vi "COD主界面（列队使用）.vi"() -> (8 "多列列表框":i32(listbox))   [LabVIEW 2016, in "斯坦道CODMn.lvlib"]
uses:
  <vilib>/Analysis/6fits.llb/Curve Fitting Criteria.ctl
  <vilib>/Utility/miscctls.llb/LVPointTypeDef.ctl
  <vilib>/Utility/config.llb/Read Key (I32).vi
  <vilib>/Utility/config.llb/Read Key (Double).vi
  <vilib>/Utility/config.llb/Read Key (Boolean).vi
  <vilib>/Utility/config.llb/Write Key (Double).vi
  <vilib>/Utility/config.llb/Write Key (Boolean).vi
  <vilib>/Utility/config.llb/Write Key (I32).vi
  <vilib>/Waveform/WDTFileIO.llb/Read Waveform from File.vi
  <vilib>/ptbypt/NI_PtbyPt.lvlib
  <vilib>/Utility/config.llb/NI_LVConfig.lvlib
  <vilib>/Analysis/NI_AALPro.lvlib
panel:
  out "CODMn序列号":string
  out "CODMn软件版本：":string
  in  "标样核查量程选择":enum32{"H", "L", "AUTO"}(ring)=enum."AUTO"
  in  "标样浓度":dbl
  in  "零点核查量程选择":enum32{"H", "L", "AUTO"}(ring)=enum."AUTO"
  in  "零点核查浓度":dbl
  out "序列号":string
  in  "采水泵排液时间/s:":i32
  in  "采水泵润洗时间/s:":i32
  in  "采水泵沉淀时间/s:":i32
  in  "采水泵进样时间/s:":i32
  in  "常规版/认证版":enum16{"常规版", "认证版", "浮台版"}(ring)
  in  "释放串口":bool
  in  "打开串口":bool
  in  "保存参数":dbl[](array[numeric])
  out "报警数字":i16
  out "CODMn工作状态":T1(ring)
  out "ORP-K":string
  out "ORP-B":string
  out "ORP-A":string
  out "x = y?":bool
  out "稀释倍数解释":string
  in  "跨度量程选择":enum32{"H", "L", "AUTO"}(ring)=enum."AUTO"
  in  "跨度液浓度":dbl
  in  "水样":dbl
  in  "蒸馏水":dbl
  in  "标液":dbl
  in  "质控样":dbl
  in  "加标回收":dbl
  in  "草酸钠":dbl
  in  "高锰酸钾":dbl
  in  "硫酸":dbl
  out "量程解释说明":string
  in  "高切低阈值:":dbl
  in  "低切高阈值:":dbl
  in  "自动切换量程:":enum16{"关闭", "自动切换测一次", "自动切换测两次"}(ring)
  in  "修正系数":dbl
  in  "标准液浓度":dbl
  in  "温度":dbl
  in  "恒温时间":dbl
  in  "基本量程":enum16{"L", "H"}(ring)
  in  "CODMn零点核查选择":enum16{"零点核查走纯水管", "零点核查走零漂管"}(ring)
  in  "锁定按钮":bool
  in  "低量程稀释倍数:":i8=1
  out "切换量程连续测两次":bool
  in  "高量程稀释倍数:":i8=2
  in  "一键写入":bool
  in  "测量模式(公式)":u16(ring)=1 items=["水样测试"=1, "标样核查"=2, "零点核查"=3, "跨度核查"=4, "空白测试"=5, "平行样"=6, "加标回收"=7]
  out "基本量程(显示)":string
  out "测量模式(显示)":string
  in  "量程切换次数":u8
  out "数据时间":string
  out "断电排液标记":bool
  out "COM":string
  in  "启用5":bool
  in  "校准5":bool
  in  "泵滴定数5":dbl
  in  "浓度5":dbl
  in  "启用4":bool
  in  "校准4":bool
  in  "泵滴定数4":dbl
  in  "浓度4":dbl
  out "波形时间":timestamp
  in  "历史波形":bool
  out "滴定数-ORP值":u16[](array[numeric]) caption="数组"
  in  "关闭 3":bool
  in  "滴定曲线":bool
  out "ORP滴定曲线":u16[](graph)
  out "空白测试标记":bool
  out "跨度核查标记":bool
  out "启动选择 2":u16(ring) items=["水样测试", "标样核查", "零点核查", "跨度核查", "空白测试", "加标回收", "平行样", "校零", "校标"]
  in  "量程选择":enum16{"低量程", "高量程", "0-2量程"}(ring)
  in  "手动控制":bool
  in  "选用水样":enum16{"葡萄糖", "草酸钠"}(ring)
  in  "方程系数":cluster{"K":dbl, "b":dbl, "X^2":dbl} {"X^2" format="%#.6g"; "b" format="%#.6g"; "K" format="%#.6g"}
  out "多项式系数":dbl[](array[numeric])
  out "XY图":cluster{"X Values":dbl[], "Y Values":dbl[]}[](graph)
  in  "模型":enum32{"线性", "多项式"}(ring)
  out "启动时间":timestamp format="%<%Y/%m/%d %H:%M:%S>T"
  in  "关闭 2":bool
  out "r^2":dbl format="%.8g"
  out "拟合公式":string
  out "b":dbl format="%#.4g"
  out "K":dbl format="%#.4f"
  out "当前校准":i32
  in  "启用3":bool
  in  "启用2":bool
  in  "启用1":bool
  in  "校准3":bool
  in  "校准2":bool
  in  "校准1":bool
  in  "泵滴定数3":dbl
  in  "泵滴定数2":dbl
  in  "泵滴定数1":dbl
  in  "浓度3":dbl
  in  "浓度2":dbl
  in  "浓度1":dbl
  in  "写入":bool
  out "测量模式数字":i32
  out "零点核查标记":bool
  out "排液故障":bool
  out "进水样超量程":bool
  out "标样核查标记":bool
  out "平行样测量":bool
  out "加标回收测量":bool
  out "质控样测量":bool
  out "待机":bool
  out "校标错误":bool
  out "校零错误":bool
  out "测量错误":bool
  out "草酸钠报警":bool
  out "高锰酸钾报警":bool
  out "加热故障":bool
  out "温控器故障":bool
  out "ORP故障":bool
  out "排液标记":bool
  out "故障标记":bool
  out "校标标记":bool
  out "校零标记":bool
  out "通讯状态":bool
  out "水样测量":bool
  in  "读取":bool
  in  "返回":bool
  in  "校准配置":bool
  in  "零点泵计量数 2":dbl
  in  "标度泵计量数 2":dbl
  out "标度滴定值":dbl
  out "零点滴定值":dbl
  in  "保存":bool
  in  "关闭":bool
  out "仪器时间":timestamp format="%<%Y/%m/%d %H:%M:%S>T"
  out "秒":u16
  out "分":u16
  out "COD浓度（mg/L)":dbl format="%.2g"
  out "进样管":dbl
  out "高锰酸钾":dbl
  out "草酸钠":dbl
  out "硫酸":dbl
  out "ORP显示":dbl
  out "温度":dbl
  out "加热":bool
  out "搅拌":bool
  out "进硫酸":bool
  out "进加标回收样":bool
  out "进零点核查样":bool
  out "进标液":bool
  out "进蒸馏水":bool
  out "进水样":bool
  out "进草酸钠":bool
  out "进高锰酸钾":bool
  out "定时启动":bool
  in  "启动":bool
  in  "故障清除":bool
  in  "参数配置":bool
  in  "停止":bool
  in  "单步启动":bool
  out "系统时间":timestamp
  in  "时间校准":bool
  out "报警簇":T2
  out "模式（受控）":u16
  # "测量时间："
  # "(水样~加标回收)"
  # "mV"
  # "℃"
  # "注：遇到加热故障和排液故障时仪器不能正常启动，\n必须排查故障并点击报警清除按钮方可运行。"
  # "mg/L"
  # "基本参数设置"
  # "校零校标结果"
  # "泵计量参数设置"
  # "校零结果："
  # "校零滴定值："
  # "加热恒温温度(℃):"
  # "水样："
  # "高锰酸钾："
  # "校标结果："
  # "标度滴定值："
  # "恒温时间(分钟):"
  # "草酸钠："
  # "蒸馏水："
  # "零点泵计量值："
  # "标准液浓度(mg/L):"
  # "硫酸："
  # "标液："
  # "标度泵计量值："
  # "修正系数："
  # "跨度核查浓度："
  # "零点核查样:"
  # "基本量程(L、H)可选:"
  # "跨度量程选择："
  # "加标回收样："
  # "零点核查浓度："
  # "标样浓度："
  # "零点量程选择："
  # "标样量程选择："
  # "是否启用"
  # "泵滴定数"
  # "浓度"
  # "辅\n助\n计\n算\n区"
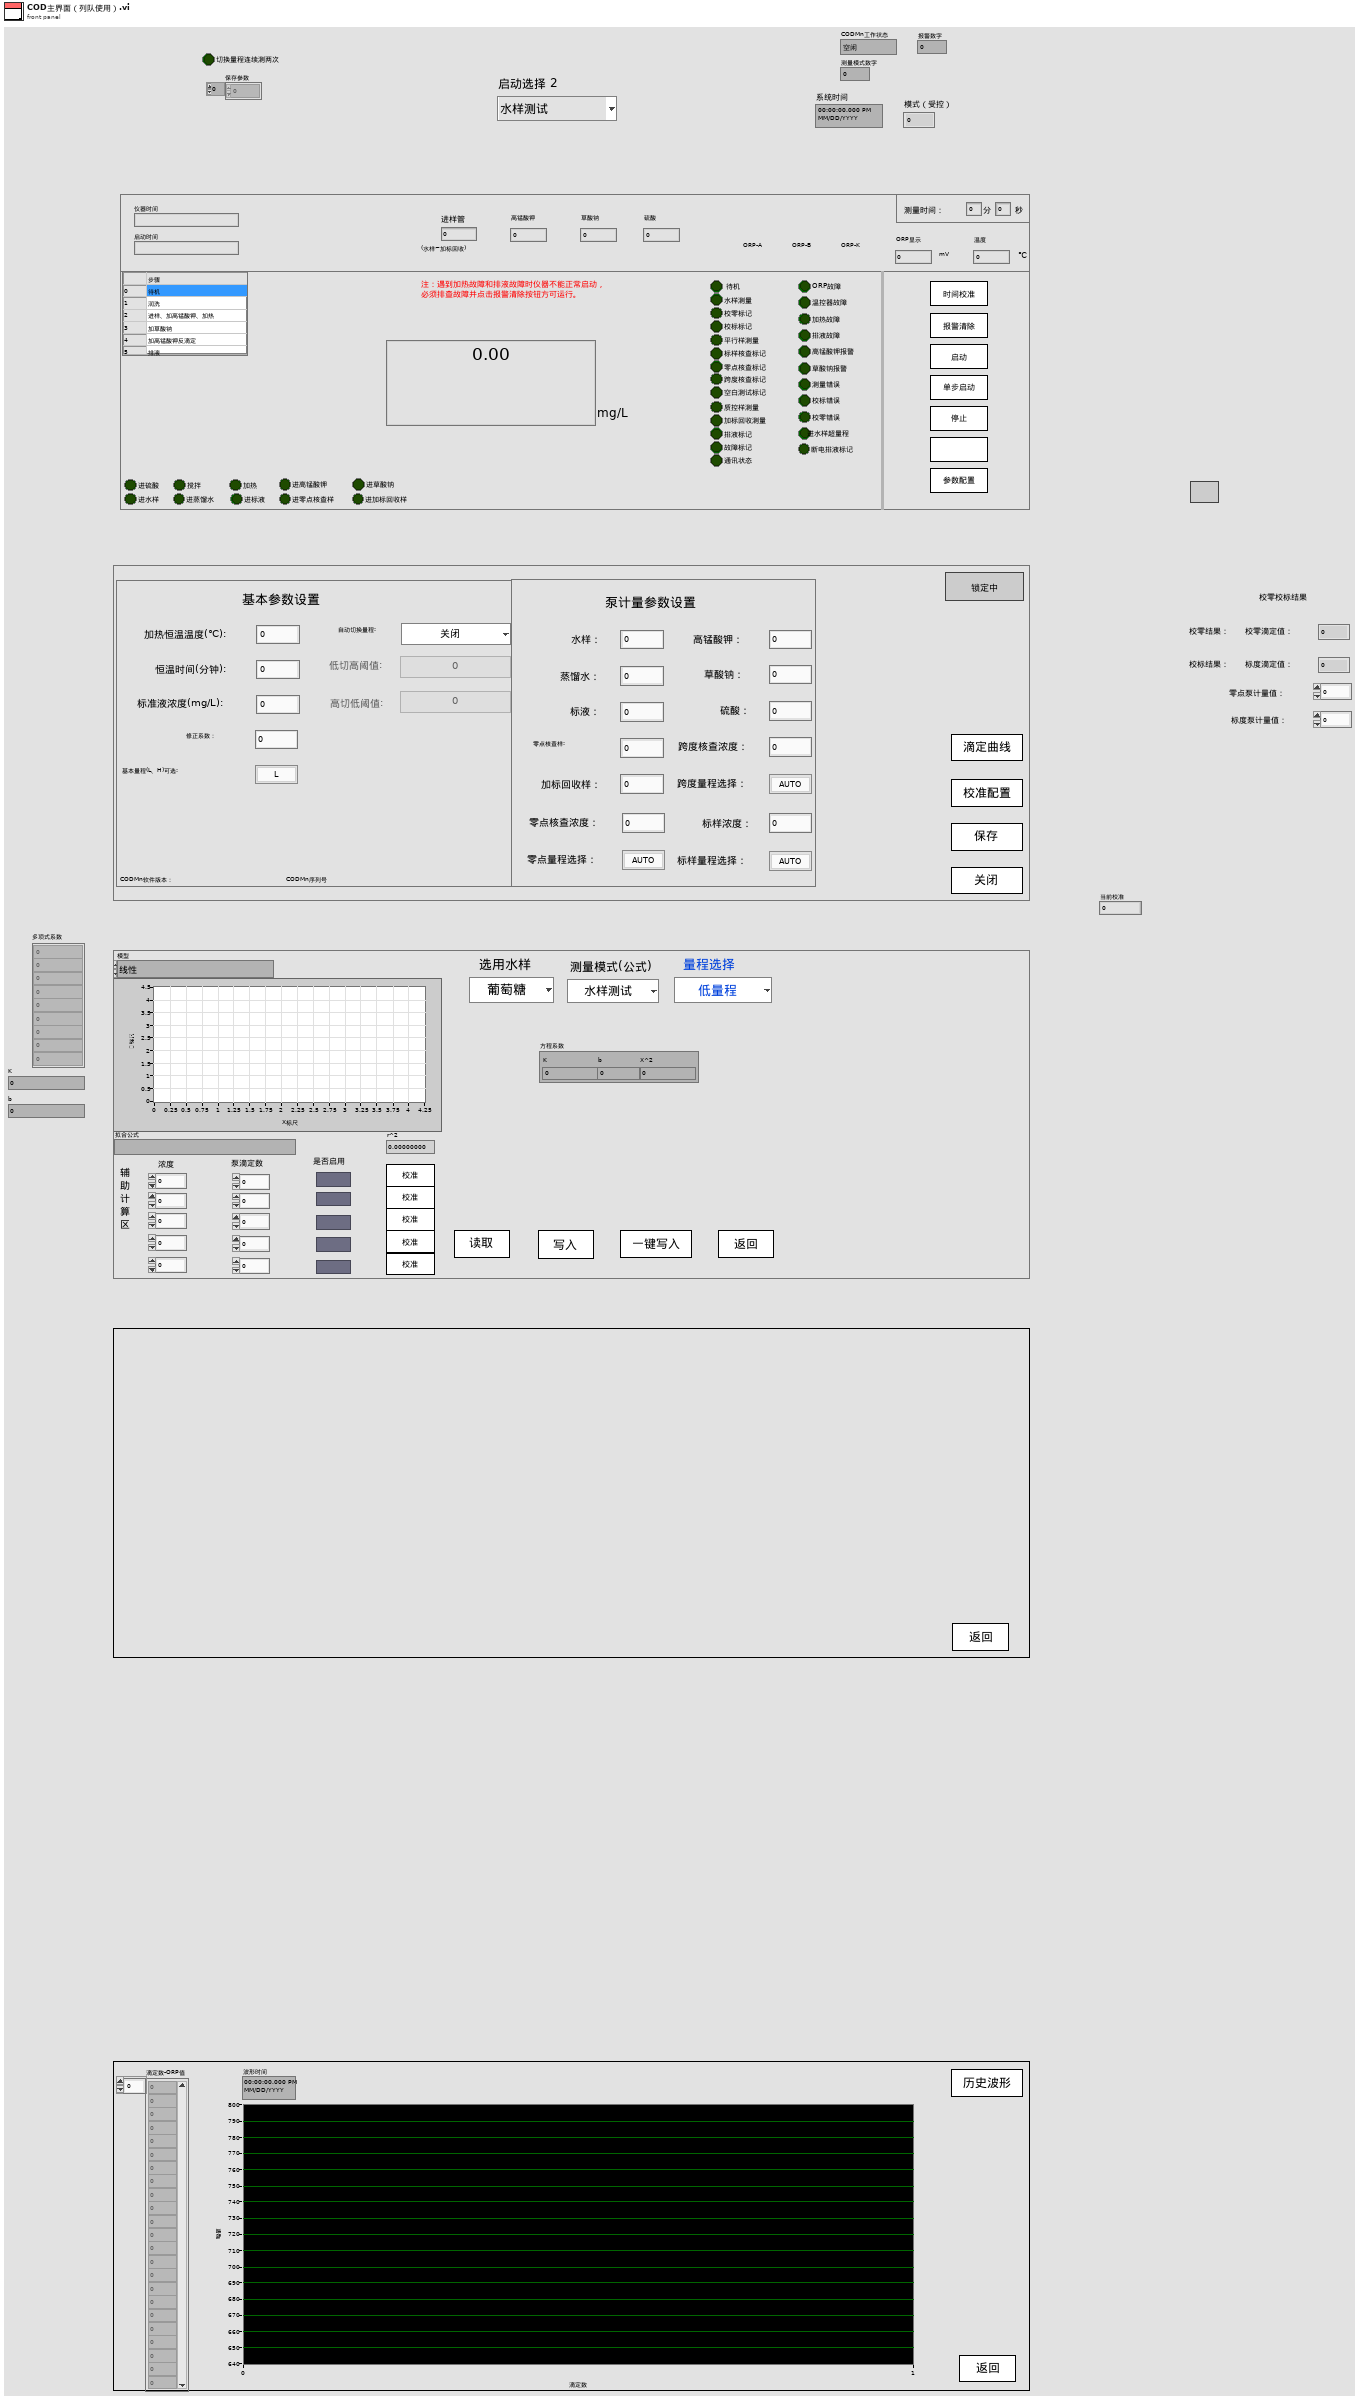
[diagram p1: front panel]
types:
  T1 = enum16{"空闲", "水样测试", "标样核查", "零点核查", "跨度核查", "空白测试", "平行样测试", "质控样", "空白校准", "标样校准", "加标回收"}
  T2 = cluster{"ORP故障":bool, "温控器故障":bool, "加热故障":bool, "高锰酸钾报警":bool, "草酸钠报警":bool, "测量错误":bool, "校零错误":bool, "校标错误":bool, " 进水样超量程":bool, "排液阀故障":bool}
  T3 = cluster{"命令":string, "测量模式":enum16{"水样测量", "标样核查", "零点核查", "跨度核查", "空白测试", "加标回收", "平行样", "校零", "校标"}, "CODMn量程切换":enum32{"H", "L", "AUTO"}}
  T4 = cluster{"时间":timestamp, "测量模式":string, "数据类型":string, "检测值":sgl, "单位":string, "数据标识":string, "因子编码":string, "标样参考值":sgl, "ORP-A":sgl, "ORP-B":sgl, "ORP-K":sgl, "COD滴定值":sgl, "高锰酸钾滴定数":sgl, "温度":sgl, "量程":sgl, "LastTime":timestamp}
  T5 = cluster{"因子编码":u32, "单位":u16, "标样参考值":sgl, "水样数据时间":timestamp, "水样实测值":sgl, "水样数据标识":string, "标样数据时间":timestamp, "标样实测值":sgl, "标样数据标识":string, "空白数据时间":timestamp, "空白实测值":sgl, "空白数据标识":string, "零点核查数据时间":timestamp, "零点核查实测值":sgl, "零点核查数据标识":string, "跨度核查数据时间":timestamp, "跨度核查实测值":sgl, "跨度核查数据标识":string, "加标回收数据时间":timestamp, "加标回收实测值":sgl, "加标回收数据标识":string, "平行样数据时间":timestamp, "平行样实测值":sgl, "平行样数据标识":string}
  T6 = enum8{"Enabled", "Disabled", "Disabled and Grayed Out"}
  T7 = typedef "NI_LVConfig.lvlib/Config Data RefNum.ctl" = refnum<k1>
  T8 = cluster{"数组 2[0]":sgl, "数组 2[1]":sgl, "数组 2[2]":sgl, "数组 2[3]":sgl, "数组 2[4]":sgl, "数组 2[5]":sgl, "数组 2[6]":sgl, "数组 2[7]":sgl, "数组 2[8]":sgl, "数组 2[9]":sgl, "数组 2[10]":sgl, "数组 2[11]":sgl, "数组 2[12]":sgl, "数组 2[13]":sgl, "数组 2[14]":sgl, "数组 2[15]":sgl, "数组 2[16]":sgl, "数组 2[17]":sgl, "数组 2[18]":sgl, "数组 2[19]":sgl, "数组 2[20]":sgl, "数组 2[21]":sgl, "数组 2[22]":sgl, "数组 2[23]":sgl, "数组 2[24]":sgl, "数组 2[25]":sgl, "数组 2[26]":sgl, "数组 2[27]":sgl, "数组 2[28]":sgl, "数组 2[29]":sgl, "数组 2[30]":sgl, "数组 2[31]":sgl, "数组 2[32]":sgl, "数组 2[33]":sgl, "数组 2[34]":sgl, "数组 2[35]":sgl, "数组 2[36]":sgl, "数组 2[37]":sgl, "数组 2[38]":sgl, "数组 2[39]":sgl, "数组 2[40]":sgl, "数组 2[41]":sgl}
  T9 = typedef "NI_AALPro.lvlib/Curve Fitting Criteria.ctl" = u16
  T10 = cluster{"测量模式":enum16{"水样测量", "标样核查", "零点核查", "跨度核查", "空白测试", "加标回收", "平行样", "校零", "校标"}}
  T11 = cluster{"仪器测试类型":enum16{"水样测试", "零点核查", "标样核查", "空白测试", "跨度核查", "加标回收", "平行样", "校零", "校标"}, "周期设置类型":enum16{"定点启动", "间隔启动"}, "定时功能启用":bool, "定时间隔":dbl, "24H周期设置":bool[]}
  T12 = typedef "LVDateTimeRec.ctl" = cluster{"秒数的小数部分":dbl, "秒":i32, "分":i32, "时":i32, "日":i32, "月":i32, "年":i32, "天数（周）":i32, "天数（年）":i32, "DST":i32}
  T13 = enum16{"水样测试", "零点核查", "标样核查", "空白测试", "跨度核查", "加标回收", "平行样", "校零", "校标"}
  T14 = cluster{"时间标识":timestamp, "设备":string, "日志信息":string}
  T15 = cluster{"时间标识":timestamp, "参数":string, "日志信息":string, "流程参数":string}
  T16 = cluster{"时间标识":timestamp, "设备":string, "日志信息":string, "流程参数":string}
  T17 = typedef "LVPointTypeDef.ctl" = cluster{"Horizontal":i16, "Vertical":i16}
  T18 = enum16{"水样测量", "标样核查", "零点核查", "跨度核查", "空白测试", "加标回收", "平行样", "校零", "校标"}
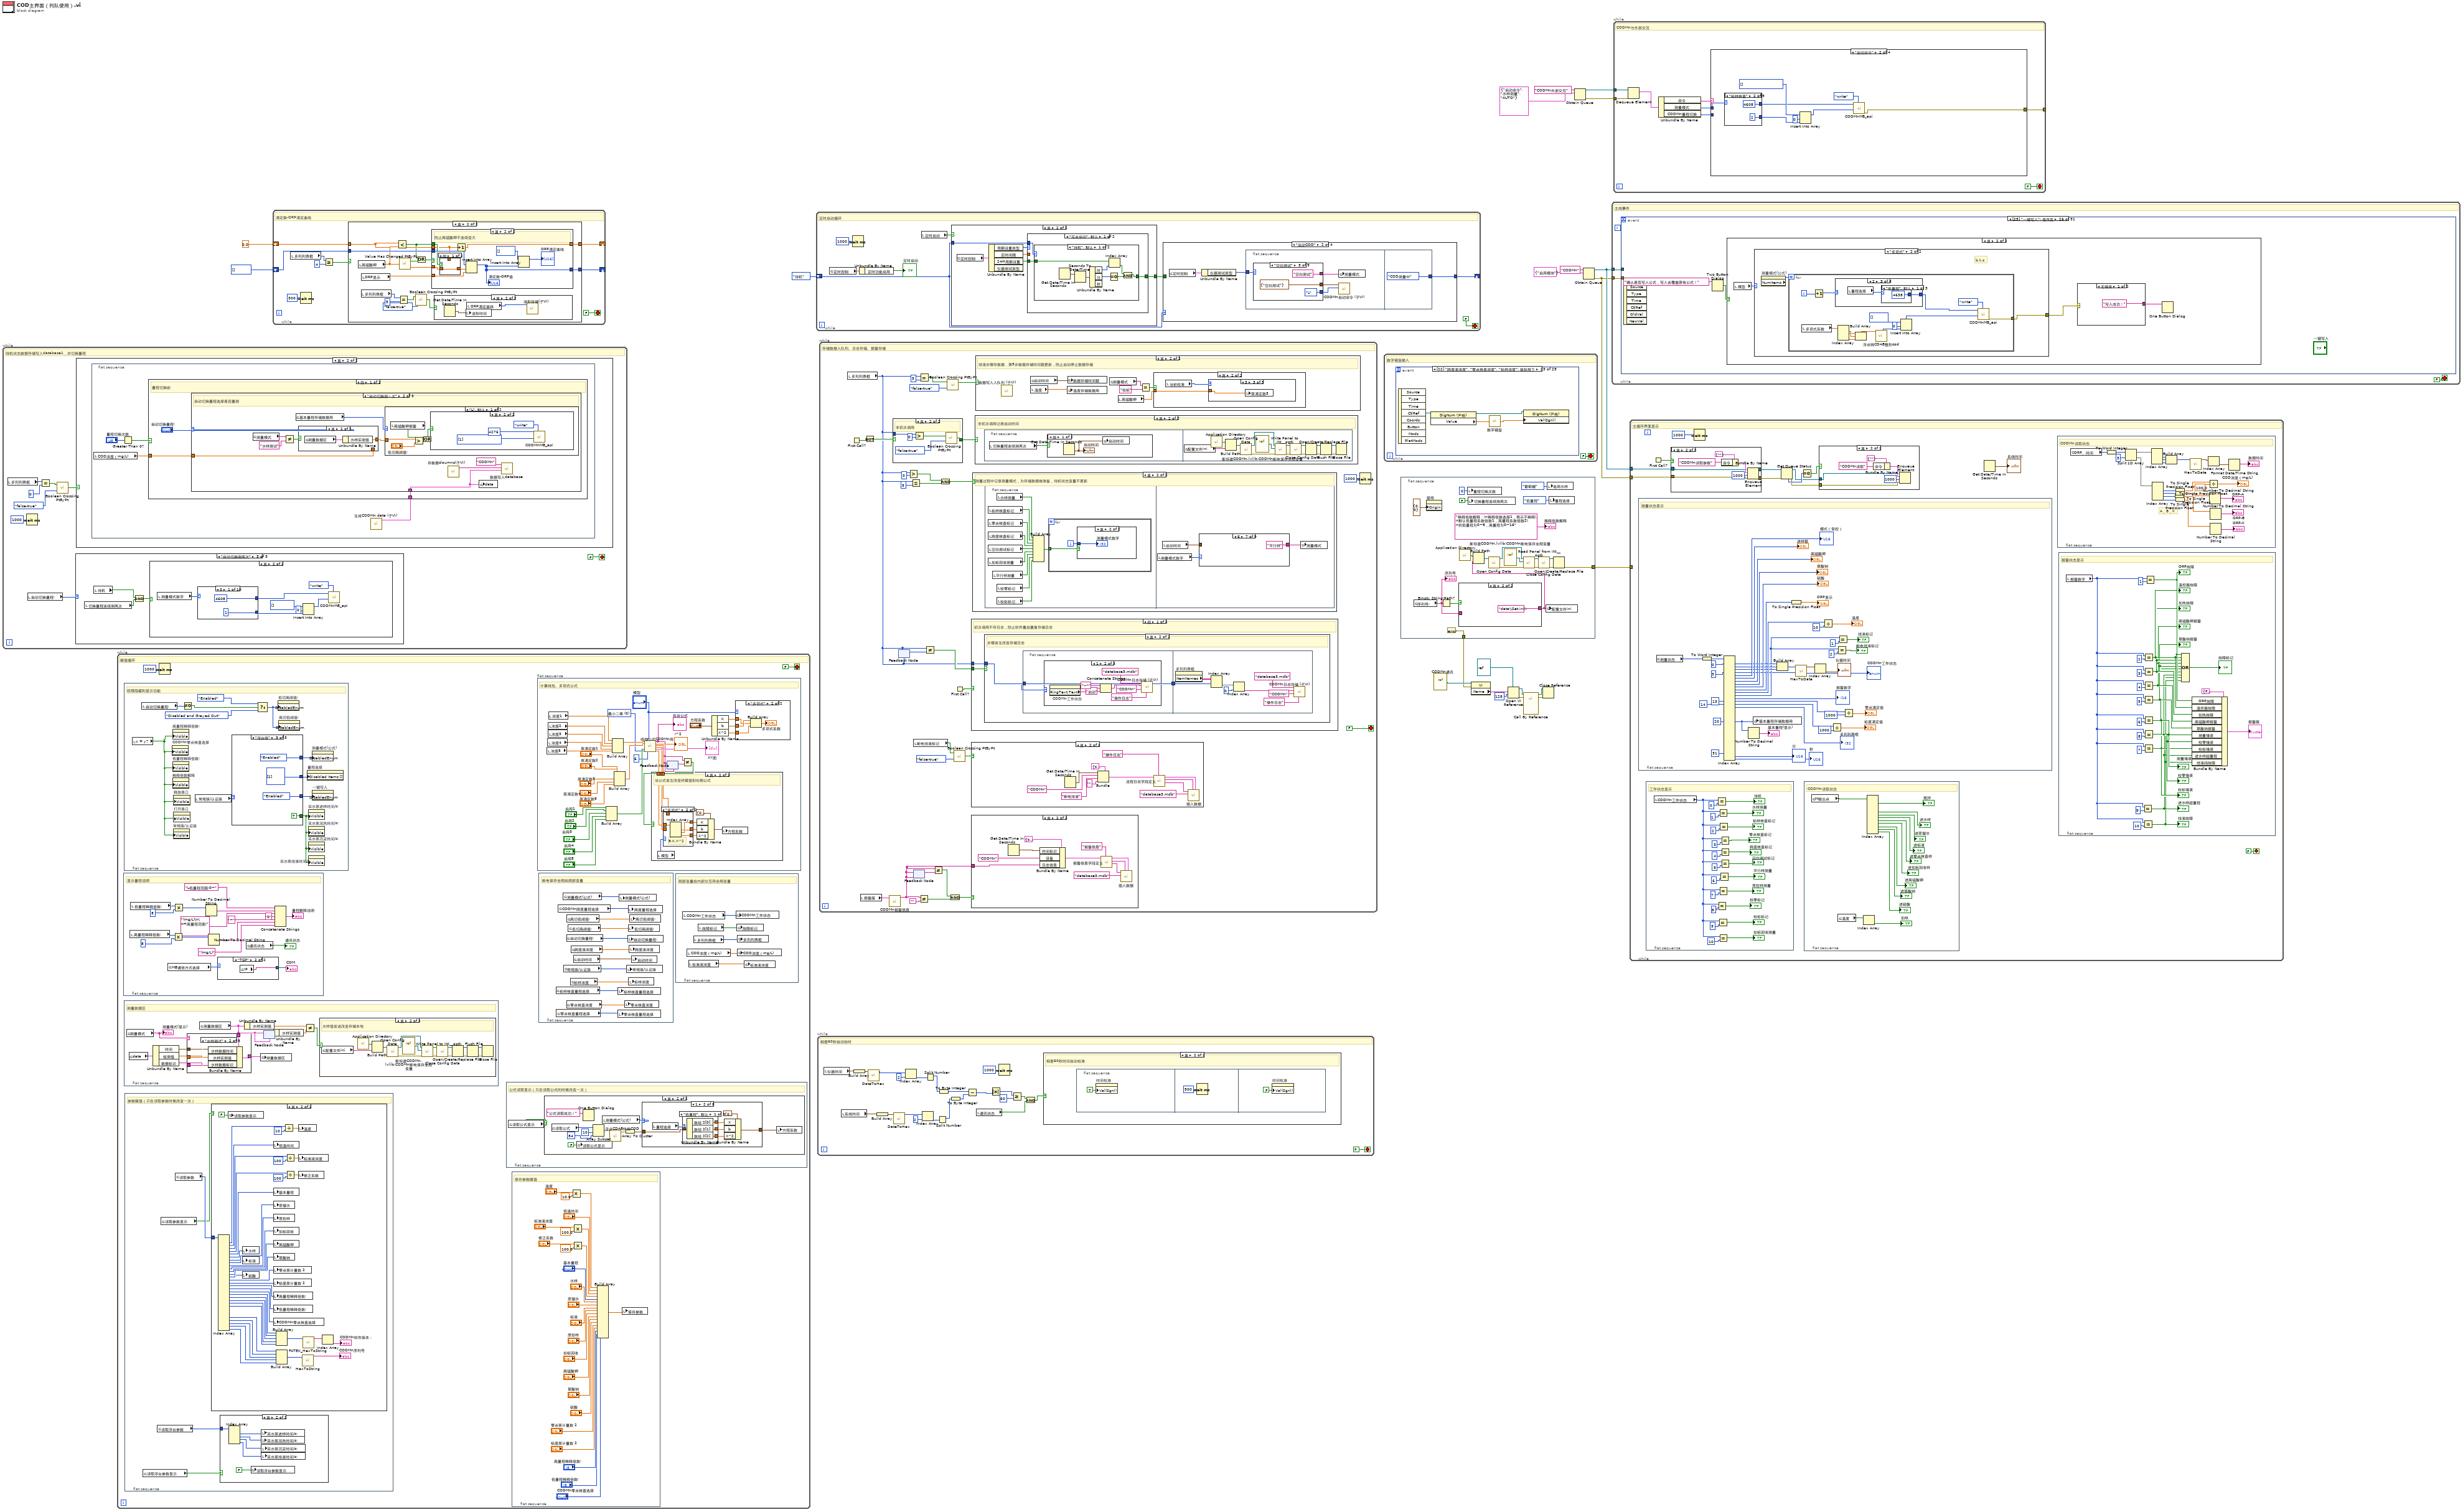
[diagram p0: block diagram]
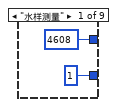
[diagram p3: hidden frame]
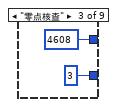
[diagram p4: hidden frame]
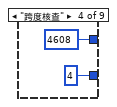
[diagram p5: hidden frame]
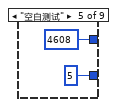
[diagram p6: hidden frame]
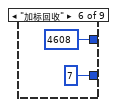
[diagram p7: hidden frame]
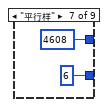
[diagram p8: hidden frame]
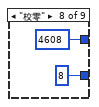
[diagram p9: hidden frame]
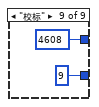
[diagram p10: hidden frame]
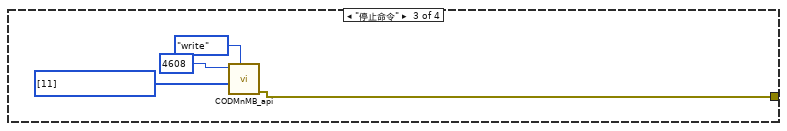
[diagram p11: hidden frame]
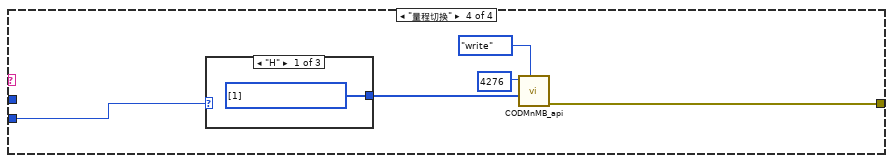
[diagram p12: hidden frame]
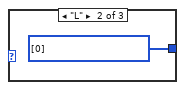
[diagram p13: hidden frame]
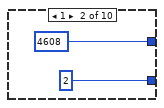
[diagram p19: hidden frame]
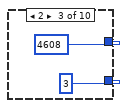
[diagram p20: hidden frame]
diagram:
  n1 = while {
    stop <- FALSE stop-if-true
    # "待机状态数据存储写入database1，并切换量程"
    n2 = local read "多列列表框"() -> (w27:i32)
    n3 = Wait (ms)(milliseconds to wait=u32 1000 ("等待时间（毫秒）")) -> ()  [unwired: 1 out]
    n4 = local read "自动切换量程:"() -> (w22:enum16{"关闭", "自动切换测一次", "自动切换测两次"})
    n5 = Equal?(x=w27, y=0) -> (x = y?=w25:bool)
    n6 = call <vilib>:"Boolean Crossing PtByPt.vi"("direction"=enum16{"either", "false-true", "true-false"}."false-true", "input"=w25) -> ("crossing"=w23:bool)  [unwired: 1 in]
    n7 = case shown="\"自动切换测两次\"" w22 {
      frame "关闭", Default {
      }
      frame "自动切换测一次" {
      }
      frame "自动切换测两次" {
        n8 = local read "切换量程连续测两次"() -> (w31:bool)
        n9 = local read "待机"() -> (w32:bool)
        n10 = Compound Arithmetic op=AND ("复合运算")(w32, w31) -> (w30:bool)
        n11 = case shown="真" w30 {
          frame False {
          }
          frame True {
            n12 = local read "测量模式数字"() -> (w36:i32)
            n13 = case shown="0" w36 {
              tunnel: [u16 4608 ("address") u16 4608 ("address") u16 4608 ("address") u16 4608 ("address") u16 4608 ("address") u16 4608 ("address") u16 4608 ("address") u16 4608 ("address") u16 4608 ("address") u16 4608 ("address")] -> w33
              tunnel: [u16 1 ("address") u16 2 ("address") u16 3 ("address") u16 4 ("address") u16 5 ("address") u16 7 ("address") u16 6 ("address") u16 8 ("address") u16 9 ("address") u16 0 ("address")] -> w39
              frame 0 {
              }
              frame 1 {
              }
              frame 2 {
              }
              frame 3 {
              }
              frame 4 {
              }
              frame 5 {
              }
              frame 6 {
              }
              frame 7 {
              }
              frame 8 {
              }
              frame 9, Default {
              }
            }
            n14 = Insert Into Array(array=u16[] [] ("values"), index=0 ("索引"), new element=w39) -> (w34:u16[])
            n15 = call "CODMnMB_api.vi"("STEP"=enum16{"open", "read", "write", "close"}."write", "values"=w34, "starting address"=w33) -> ()  [unwired: 6 in, 3 out]
          }
        }
      }
    }
    n16 = case shown="真" w23 {
      frame False {
      }
      frame True {
        n17 = flat-sequence {
          frame #0 {
            n18 = local read "COD浓度（mg/L)"() -> (w60:dbl)
            n19 = Greater Than 0?(x="量程切换次数") -> (x > 0?=w61:bool)
            n20 = call "生成CODMn data (子VI).vi"() -> ("data"=w63:T4)  [unwired: 11 in]
            n21 = case shown="假" w61 {
              tunnel: w63 -> [w65 w124]
              tunnel: w60 -> [w64 _]
              frame False {
                # "量程切换前"
                n22 = case shown="\"自动切换测一次\"" "自动切换量程:" {
                  tunnel: w65 -> [w67 w72 w98]
                  tunnel: w64 -> [_ w71 w97]
                  frame "关闭", Default {
                    # "关闭自动切换量程"
                    n23 = call "存数据cloumns(子VI).vi"() -> ("数组"=w69:string[])  [unwired: 11 in]
                    n24 = global write "COD读取DATA全局.vi" "data"(w67) -> ()
                    n25 = call "数据写入database.vi"("data"=w67, "columns"=w69, "table"="CODMn") -> ()  [unwired: 8 in, 1 out]
                  }
                  frame "自动切换测一次" {
                    # "自动切换量程选择是否重测"
                    n26 = global read "COD测量模式全局.vi" "测量模式"() -> (w78:string)
                    n27 = Not Equal?(x=w78, y="水样测试") -> (x != y?=w76:bool)
                    n28 = global read "COD读取DATA全局.vi" "基本量程存储数据用"() -> (w70:enum16{"L", "H"})
                    n29 = case shown="真" w76 {
                      tunnel: [w79 w80] -> w75
                      tunnel: w71 -> [w79 _]
                      frame False {
                      }
                      frame True {
                        n30 = global read "CODMn断电保存全局变量.vi" "测量数据区"() -> (w81:T5)
                        n31 = Unbundle By Name(w81) -> ("水样实测值"=w80:sgl)
                      }
                    }
                    n32 = case shown="\"L\", 默认" w70 {
                      tunnel: w75 -> [w84 w90]
                      frame "L", Default {
                        n33 = local read "高锰酸钾报警"() -> (w82:bool)
                        n34 = Greater?(x=w84, y="低切高阈值:") -> (0:w85:bool)
                        n35 = Or(x=w82, y=w85) -> (x .or. y?=w83:bool)
                        n36 = case shown="真" w83 {
                          frame False {
                          }
                          frame True {
                            n37 = call "CODMnMB_api.vi"("STEP"=enum16{"open", "read", "write", "close"}."write", "values"=u16[] [1], "starting address"=u16 4276) -> ()  [unwired: 6 in, 3 out]
                          }
                        }
                      }
                      frame "H" {
                        n38 = Less?(x=w90, y="高切低阈值:") -> (x < y?=w91:bool)
                        n39 = case shown="真" w91 {
                          frame False {
                          }
                          frame True {
                            n40 = call "CODMnMB_api.vi"("STEP"=enum16{"open", "read", "write", "close"}."write", "values"=u16[] [0], "starting address"=u16 4276) -> ()  [unwired: 6 in, 3 out]
                          }
                        }
                      }
                    }
                    n41 = call "存数据cloumns(子VI).vi"() -> ("数组"=w74:string[])  [unwired: 11 in]
                    n42 = global write "COD读取DATA全局.vi" "data"(w72) -> ()
                    n43 = call "数据写入database.vi"("data"=w72, "columns"=w74, "table"="CODMn") -> ()  [unwired: 8 in, 1 out]
                  }
                  frame "自动切换测两次" {
                    # "自动切换量程选择是否重测"
                    n44 = global read "COD读取DATA全局.vi" "基本量程存储数据用"() -> (w96:enum16{"L", "H"})
                    n45 = case shown="\"L\", 默认" w96 {
                      tunnel: w97 -> [w102 w113]
                      tunnel: w98 -> [w101 w112]
                      frame "L", Default {
                        n46 = local read "低切高阈值:"() -> (w103:dbl)
                        n47 = local read "高锰酸钾报警"() -> (w99:bool)
                        n48 = Greater?(x=w102, y=w103) -> (0:w104:bool)
                        n49 = Or(x=w104, y=w99) -> (x .or. y?=w100:bool)
                        n50 = case shown="真" w100 {
                          tunnel: w101 -> [w105 _]
                          frame False {
                            n51 = call "存数据cloumns(子VI).vi"() -> ("数组"=w107:string[])  [unwired: 11 in]
                            n52 = global write "COD读取DATA全局.vi" "data"(w105) -> ()
                            n53 = call "数据写入database.vi"("data"=w105, "columns"=w107, "table"="CODMn") -> ()  [unwired: 8 in, 1 out]
                          }
                          frame True {
                            n54 = call "CODMnMB_api.vi"("STEP"=enum16{"open", "read", "write", "close"}."write", "values"=u16[] [1], "starting address"=u16 4276) -> ()  [unwired: 6 in, 3 out]
                            "切换量程连续测两次" <- TRUE ("切换量程连续测两次")
                          }
                        }
                      }
                      frame "H" {
                        n55 = local read "高切低阈值:"() -> (w114:dbl)
                        n56 = Less?(x=w113, y=w114) -> (x < y?=w115:bool)
                        n57 = case shown="真" w115 {
                          tunnel: w112 -> [w116 _]
                          frame False {
                            n58 = call "存数据cloumns(子VI).vi"() -> ("数组"=w118:string[])  [unwired: 11 in]
                            n59 = global write "COD读取DATA全局.vi" "data"(w116) -> ()
                            n60 = call "数据写入database.vi"("data"=w116, "columns"=w118, "table"="CODMn") -> ()  [unwired: 8 in, 1 out]
                          }
                          frame True {
                            # "重测第一次不存数据"
                            n61 = call "CODMnMB_api.vi"("STEP"=enum16{"open", "read", "write", "close"}."write", "values"=u16[] [0], "starting address"=u16 4276) -> ()  [unwired: 6 in, 3 out]
                            n62 = local write "切换量程连续测两次"(TRUE ("切换量程连续测两次")) -> ()
                          }
                        }
                      }
                    }
                  }
                }
              }
              frame True {
                # "防止无限切量程"
                n63 = local write "量程切换次数"(u8 0 ("量程切换次数")) -> ()
                n64 = call "存数据cloumns(子VI).vi"() -> ("数组"=w126:string[])  [unwired: 11 in]
                n65 = call "数据写入database.vi"("data"=w124, "columns"=w126, "table"="CODMn") -> ()  [unwired: 8 in, 1 out]
                n66 = global write "COD读取DATA全局.vi" "data"(w124) -> ()
              }
            }
          }
        }
      }
    }
  }
  n67 = while {
    stop <- FALSE stop-if-true
    # "赋值循环"
    n68 = flat-sequence {
      frame #0 {
        # "显示量程说明"
        n69 = local read "高量程稀释倍数:"() -> (w487:i8)
        n70 = local read "低量程稀释倍数:"() -> (w497:i8)
        n71 = global read "CODMn断电保存全局变量.vi" "MB通信方式选择"() -> (w483:enum16{"串口", "TCP"})
        n72 = Multiply(x=w487, y=i8 8) -> (x*y=w485:i8)
        n73 = Multiply(x=w497, y=i8 8) -> (x*y=w489:i8)
        n74 = Number To Decimal String(number=w489) -> (decimal integer string=w494:string)  [unwired: 1 in]
        n75 = Number To Decimal String(number=w485) -> (decimal integer string=w492:string)  [unwired: 1 in]
        n76 = case shown="\"TCP\"" w483 {
          tunnel: [w500 w501] -> w488
          frame "串口", Default {
            n77 = global read "CODMn断电保存全局变量.vi" "VISA resource name"() -> (w500:refnum<visa-resource-name>)
          }
          frame "TCP" {
            n78 = global read "CODMn断电保存全局变量.vi" "IP"() -> (w501:string)
          }
        }
        "COM" <- w488
        n79 = global read "COD读取DATA全局.vi" "通讯状态"() -> (→"通讯状态":bool)
        n80 = Concatenate Strings("L低量程范围:0~" ("量程解释说明"), w494, "(mg/L)\n\nH高量程范围:" ("量程解释说明"), "0" ("字符串"), "~" ("量程解释说明"), w492, "(mg/L)" ("量程解释说明")) -> (→"量程解释说明":string)
      }
    }
    n81 = flat-sequence {
      frame #0 {
        # "权限隐藏和显示功能"
        n82 = local read "x = y?"() -> (w502:bool)
        n83 = local read "自动切换量程:"() -> (w509:enum16{"关闭", "自动切换测一次", "自动切换测两次"})
        n84 = property on="CODMn零点核查选择" class="Enum (严格)"("Visible"=w502) -> ()  [unwired: 2 in, 2 out]
        n85 = property on="高量程稀释倍数:" class="DigNum (严格)"("Visible"=w502) -> ()  [unwired: 2 in, 2 out]
        n86 = property on="低量程稀释倍数:" class="DigNum (严格)"("Visible"=w502) -> ()  [unwired: 2 in, 2 out]
        n87 = property on="稀释倍数解释" class="Str"("Visible"=w502) -> ()  [unwired: 2 in, 2 out]
        n88 = property on="常规版/认证版" class="Enum (严格)"("Visible"=w502) -> ()  [unwired: 2 in, 2 out]
        n89 = property on="释放串口" class="Bool"("Visible"=w502) -> ()  [unwired: 2 in, 2 out]
        n90 = property on="打开串口" class="Bool"("Visible"=w502) -> ()  [unwired: 2 in, 2 out]
        n91 = Not Equal To 0?(x=w509) -> (x != 0?=w508:bool)
        n92 = local read "常规版/认证版"() -> (w507:enum16{"常规版", "认证版", "浮台版"})
        n93 = case shown="\"浮台版\"" w507 {
          tunnel: [T6."Enabled" ("禁用") T6."Disabled and Grayed Out" ("禁用") T6."Enabled" ("禁用")] -> w506
          tunnel: [i32[] [2] ("禁用项[]") i32[] [] ("禁用项[]") i32[] [2] ("禁用项[]")] -> w505
          tunnel: [T6."Enabled" ("禁用") T6."Disabled and Grayed Out" ("禁用") T6."Enabled" ("禁用")] -> w504
          tunnel: [FALSE FALSE TRUE] -> w503
          frame "常规版", Default {
          }
          frame "认证版" {
            w518 = u16 1 items=["水样测试"=1, "标样核查"=2, "零点核查"=3, "跨度核查"=4, "空白测试"=5, "平行样"=6, "加标回收"=7] ("测量模式(公式)")
            n94 = global write "CODMn断电保存全局变量.vi" "测量模式(公式)"(w518) -> ()
          }
          frame "浮台版" {
          }
        }
        n95 = Select(t=T6."Enabled" ("禁用"), s=w508, f=T6."Disabled and Grayed Out" ("禁用")) -> (s? t:f=w510:T6)
        n96 = property on="低切高阈值:" class="DigNum (严格)"("DisabledEnum"=w510) -> ()  [unwired: 2 in, 2 out]
        n97 = property on="高切低阈值:" class="DigNum (严格)"("DisabledEnum"=w510) -> ()  [unwired: 2 in, 2 out]
        n98 = property on="量程选择" class="Enum (严格)"("Disabled Items []"=w505) -> ()  [unwired: 2 in, 2 out]
        n99 = property on="采水泵进样时间/s:" class="DigNum (严格)"("Visible"=w503) -> ()  [unwired: 2 in, 2 out]
        n100 = property on="采水泵润洗时间/s:" class="DigNum (严格)"("Visible"=w503) -> ()  [unwired: 2 in, 2 out]
        n101 = property on="采水泵沉淀时间/s:" class="DigNum (严格)"("Visible"=w503) -> ()  [unwired: 2 in, 2 out]
        n102 = property on="采水泵排液时间/s:" class="DigNum (严格)"("Visible"=w503) -> ()  [unwired: 2 in, 2 out]
        n103 = property on="测量模式(公式)" class="Ring (严格)"("DisabledEnum"=w506) -> ()  [unwired: 2 in, 2 out]
        n104 = property on="一键写入" class="Bool (严格)"("DisabledEnum"=w504) -> ()  [unwired: 2 in, 2 out]
      }
    }
    n105 = flat-sequence {
      frame #0 {
        # "测量数据区"
        n106 = global read "COD测量模式全局.vi" "测量模式"() -> (w416:string)
        "测量模式(显示)" <- w416
        n107 = global read "COD读取DATA全局.vi" "data"() -> (w420:T4)
        n108 = Unbundle By Name(w420) -> ("时间"=w419:timestamp, "检测值"=w418:sgl, "数据标识"=w417:string)
        n109 = global read "CODMn断电保存全局变量.vi" "测量数据区"() -> (w414:T5)
        n110 = case shown="\"水样测试\"" w416 {
          tunnel: w414 -> [w435 w440 w445 w450 w455 w460 w465 w470]
          tunnel: [w435 w439 w441 w449 w454 w459 w461 w469] -> w415
          tunnel: w419 -> [_ w438 w444 w448 w453 w458 w464 w468]
          tunnel: w418 -> [_ w437 w443 w447 w452 w457 w463 w467]
          tunnel: w417 -> [_ w436 w442 w446 w451 w456 w462 w466]
          frame "", Default {
          }
          frame "水样测试" {
            n111 = Bundle By Name(cluster=w440, "水样数据时间"=w438, "水样实测值"=w437, "水样数据标识"=w436) -> (w439:T5)
          }
          frame "标样核查" {
            n112 = Bundle By Name(cluster=w445, "跨度核查数据时间"=w444, "跨度核查实测值"=w443, "跨度核查数据标识"=w442) -> (w441:T5)
          }
          frame "零点核查" {
            n113 = Bundle By Name(cluster=w450, "零点核查数据时间"=w448, "零点核查实测值"=w447, "零点核查数据标识"=w446) -> (w449:T5)
          }
          frame "加标回收" {
            n114 = Bundle By Name(cluster=w455, "加标回收数据时间"=w453, "加标回收实测值"=w452, "加标回收数据标识"=w451) -> (w454:T5)
          }
          frame "平行样" {
            n115 = Bundle By Name(cluster=w460, "平行样数据时间"=w458, "平行样实测值"=w457, "平行样数据标识"=w456) -> (w459:T5)
          }
          frame "校零" {
            n116 = Bundle By Name(cluster=w465, "空白数据时间"=w464, "空白实测值"=w463, "空白数据标识"=w462) -> (w461:T5)
          }
          frame "校标" {
            n117 = Bundle By Name(cluster=w470, "标样数据时间"=w468, "标样实测值"=w467, "标样数据标识"=w466) -> (w469:T5)
          }
        }
        n118 = Unbundle By Name(w414) -> ("水样实测值"=w411:sgl)
        n119 = global write "CODMn断电保存全局变量.vi" "测量数据区"(w415) -> ()
        n120 = feedback-in #1(w414) -> ()
        n121 = feedback #1(w414) -> (w413:T5)
        n122 = Unbundle By Name(w413) -> ("水样实测值"=w412:sgl)
        n123 = Not Equal?(x=w411, y=w412) -> (x != y?=w410:bool)
        n124 = case shown="真" w410 {
          frame False {
          }
          frame True {
            # "水样值发送改变存储本地"
            n125 = global read "COD读取DATA全局.vi" "配置文件ini"() -> (w421:string)
            n126 = call <vilib>:"Application Directory.vi"() -> ("Application Directory"=w434:path)
            n127 = Build Path(base path=w434, name or relative path=w421) -> (appended path=w433:path)
            n128 = call <vilib>:"Open Config Data.vi"("configuration file path"=w433) -> ("error out"=w429:errorcluster, "refnum"=w432:T7)  [unwired: 8 in, 1 out]
            n129 = vi-ref "斯坦道CODMn.lvlib:CODMn断电保存全局变量.vi"() -> (w431:refnum<vi>)
            n130 = call <userlib>:"Write Panel to INI__ogtk.vi"("error in (no error)"=w429, "VI ref"=w431, "refnum"=w432) -> ("error out"=w428:errorcluster, "refnum out"=w430:T7)  [unwired: 7 in]
            n131 = call <vilib>:"Close Config Data.vi"("error in (no error)"=w428, "refnum"=w430) -> ("error out"=w423:errorcluster, "file path"=w422:path)  [unwired: 8 in]
            n132 = Open/Create/Replace File(file path (use dialog)=w422, error in=w423) -> (refnum out=w426:refnum<file>, error out=w427:errorcluster)  [unwired: 4 in, 1 out]
            n133 = Flush File(refnum=w426, error in=w427) -> (refnum out=w425:refnum<file>, error out=w424:errorcluster)
            n134 = Close File(refnum=w425, error in=w424) -> ()  [unwired: 2 out]
          }
        }
      }
    }
    n135 = flat-sequence {
      frame #0 {
        # "参数赋值（只在读取参数时候改变一次）"
        n136 = global read "COD读取DATA全局.vi" "读取浮台参数显示"() -> (w160:bool)
        n137 = global read "COD读取DATA全局.vi" "读取浮台参数"() -> (w159:u16[])
        n138 = global read "COD读取DATA全局.vi" "读取参数显示"() -> (w161:bool)
        n139 = global read "COD读取DATA全局.vi" "读取参数"() -> (w162:u16[])
        n140 = case shown="真" w161 {
          tunnel: w162 -> [_ w185]
          frame False {
          }
          frame True {
            n141 = Index Array(array=w185) -> (element #1=w197:u16, element #2=w209:u16, element #3=w190:u16, element #4=w195:u16, element #5=w193:u16, element #6=w192:u16, element #7=w208:u16, element #8=w207:u16, element #9=w206:u16, element #10=w205:u16, element #11=w204:u16, element #12=w203:u16, element #13=w202:u16, element #14=w201:u16, element #15=w200:u16, element #16=w188:u16, element #17=w187:u16, element #18=w186:u16, element #19=w183:u16, element #20=w182:u16, element #21=w181:u16, element #22=w180:u16, element #23=w179:u16, element #27=w175:u16, element #28=w174:u16, element #29=w173:u16, element #30=w172:u16, element #31=w171:u16)  [unwired: 31 in, 3 out]
            n142 = global write "COD读取DATA全局.vi" "读取参数显示"(FALSE ("读取参数显示")) -> ()
            n143 = local write "水样"(w192) -> ()
            n144 = local write "标液"(w207) -> ()
            n145 = local write "硫酸"(w202) -> ()
            n146 = local write "恒温时间"(w209) -> ()
            n147 = local write "基本量程"(w193) -> ()
            n148 = local write "蒸馏水"(w208) -> ()
            n149 = local write "质控样"(w206) -> ()
            n150 = local write "加标回收"(w205) -> ()
            n151 = local write "高锰酸钾"(w204) -> ()
            n152 = local write "草酸钠"(w203) -> ()
            n153 = local write "零点泵计量数 2"(w201) -> ()
            n154 = local write "标度泵计量数 2"(w200) -> ()
            n155 = local write "高量程稀释倍数:"(w188) -> ()
            n156 = local write "低量程稀释倍数:"(w187) -> ()
            n157 = local write "CODMn零点核查选择"(w186) -> ()
            n158 = Build Array(w175, w174, w173, w172, w171) -> (w170:u16[])
            n159 = Build Array(w183, w182, w181, w180, w179) -> (w178:u16[])
            n160 = Divide(x=w197, y=u16 10) -> (x/y=w198:dbl)
            n161 = Divide(x=w190, y=u16 100) -> (x/y=w189:dbl)
            n162 = Divide(x=w195, y=u16 100) -> (x/y=w194:dbl)
            n163 = local write "温度"(w198) -> ()
            n164 = local write "标准液浓度"(w189) -> ()
            n165 = local write "修正系数"(w194) -> ()
            n166 = call "HexToString.vi"("数组"=w170) -> ("字符串"=→"CODMn序列号":string)  [unwired: 10 in]
            n167 = call "FATEK_HexToString.vi"("数组"=w178) -> ("STRING"=w177:string[])  [unwired: 10 in]
            n168 = Index Array(array=w177) -> (element=→"CODMn软件版本：":string)  [unwired: 1 in]
          }
        }
        n169 = case shown="真" w160 {
          tunnel: w159 -> [_ w168]
          frame False {
          }
          frame True {
            n170 = Index Array(array=w168) -> (element #1=w167:u16, element #2=w166:u16, element #3=w165:u16, element #4=w164:u16)  [unwired: 4 in]
            n171 = global write "COD读取DATA全局.vi" "读取浮台参数显示"(FALSE ("读取参数显示")) -> ()
            n172 = local write "采水泵进样时间/s:"(w167) -> ()
            n173 = local write "采水泵润洗时间/s:"(w166) -> ()
            n174 = local write "采水泵沉淀时间/s:"(w165) -> ()
            n175 = local write "采水泵排液时间/s:"(w164) -> ()
          }
        }
      }
    }
    n176 = Wait (ms)(milliseconds to wait=u32 1000 ("等待时间（毫秒）")) -> ()  [unwired: 1 out]
    n177 = flat-sequence {
      frame #0 {
        # "公式读取显示（只在读取公式的时候改变一次）"
        n178 = global read "COD读取DATA全局.vi" "读取公式显示"() -> (w210:bool)
        n179 = case shown="真" w210 {
          frame False {
          }
          frame True {
            n180 = global read "COD读取DATA全局.vi" "读取公式"() -> (w220:u16[])
            n181 = global write "COD读取DATA全局.vi" "读取公式显示"(FALSE ("读取参数显示")) -> ()
            n182 = One Button Dialog(message="公式读取成功！" ("消息")) -> ()  [unwired: 1 in, 1 out]
            n183 = Array Subset(array=w220, index=10 ("索引"), length=84 ("长度")) -> (w215:u16[])
            n184 = local read "测量模式(公式)"() -> (w218:u16)
            n185 = call "浮点CDAB转换COD.vi"("数组"=w215) -> ("数组 2"=w216:sgl[])  [unwired: 10 in]
            n186 = Array To Cluster(array=w216) -> (cluster=w219:T8)
            n187 = case shown="1" w218 {
              tunnel: [cluster{"X":dbl, "b":dbl, "X^2":dbl} {"X"=999.0, "b"=999.0, "X^2"=999.0} ("方程系数") w223 w242 w261 w280 w299 w318 w337] -> w217
              tunnel: w219 -> [_ w222 w241 w260 w279 w298 w317 w336]
              frame 0, Default {
              }
              frame 1 {
                n188 = local read "量程选择"() -> (w225:enum16{"低量程", "高量程", "0-2量程"})
                n189 = case shown="\"低量程\", 默认" w225 {
                  tunnel: w222 -> [w232 w236 w240]
                  tunnel: [w231 w235 w239] -> w228
                  tunnel: [w230 w234 w238] -> w227
                  tunnel: [w229 w233 w237] -> w226
                  frame "低量程", Default {
                    n190 = Unbundle By Name(w232) -> ("数组 2[0]"=w231:sgl, "数组 2[1]"=w230:sgl, "数组 2[2]"=w229:sgl)
                  }
                  frame "高量程" {
                    n191 = Unbundle By Name(w236) -> ("数组 2[3]"=w235:sgl, "数组 2[4]"=w234:sgl, "数组 2[5]"=w233:sgl)
                  }
                  frame "0-2量程" {
                    n192 = Unbundle By Name(w240) -> ("数组 2[6]"=w239:sgl, "数组 2[7]"=w238:sgl, "数组 2[8]"=w237:sgl)
                  }
                }
                n193 = Bundle By Name(cluster=cluster{"X":dbl, "b":dbl, "X^2":dbl} {"X"=0.0, "b"=0.0, "X^2"=0.0} ("方程系数"), "X"=w228, "b"=w227, "X^2"=w226) -> (w223:cluster{"X":dbl, "b":dbl, "X^2":dbl})
              }
              frame 2 {
                n194 = local read "量程选择"() -> (w244:enum16{"低量程", "高量程", "0-2量程"})
                n195 = case shown="\"高量程\"" w244 {
                  tunnel: w241 -> [w251 w255 w259]
                  tunnel: [w250 w254 w258] -> w247
                  tunnel: [w249 w253 w257] -> w246
                  tunnel: [w248 w252 w256] -> w245
                  frame "低量程", Default {
                    n196 = Unbundle By Name(w251) -> ("数组 2[6]"=w250:sgl, "数组 2[7]"=w249:sgl, "数组 2[8]"=w248:sgl)
                  }
                  frame "高量程" {
                    n197 = Unbundle By Name(w255) -> ("数组 2[9]"=w254:sgl, "数组 2[10]"=w253:sgl, "数组 2[11]"=w252:sgl)
                  }
                  frame "0-2量程" {
                    n198 = Unbundle By Name(w259) -> ("数组 2[6]"=w258:sgl, "数组 2[7]"=w257:sgl, "数组 2[8]"=w256:sgl)
                  }
                }
                n199 = Bundle By Name(cluster=cluster{"X":dbl, "b":dbl, "X^2":dbl} {"X"=0.0, "b"=0.0, "X^2"=0.0} ("方程系数"), "X"=w247, "b"=w246, "X^2"=w245) -> (w242:cluster{"X":dbl, "b":dbl, "X^2":dbl})
              }
              frame 3 {
                n200 = local read "量程选择"() -> (w263:enum16{"低量程", "高量程", "0-2量程"})
                n201 = case shown="\"高量程\"" w263 {
                  tunnel: w260 -> [w270 w274 w278]
                  tunnel: [w269 w273 w277] -> w266
                  tunnel: [w268 w272 w276] -> w265
                  tunnel: [w267 w271 w275] -> w264
                  frame "低量程", Default {
                    n202 = Unbundle By Name(w270) -> ("数组 2[12]"=w269:sgl, "数组 2[13]"=w268:sgl, "数组 2[14]"=w267:sgl)
                  }
                  frame "高量程" {
                    n203 = Unbundle By Name(w274) -> ("数组 2[15]"=w273:sgl, "数组 2[16]"=w272:sgl, "数组 2[17]"=w271:sgl)
                  }
                  frame "0-2量程" {
                    n204 = Unbundle By Name(w278) -> ("数组 2[6]"=w277:sgl, "数组 2[7]"=w276:sgl, "数组 2[8]"=w275:sgl)
                  }
                }
                n205 = Bundle By Name(cluster=cluster{"X":dbl, "b":dbl, "X^2":dbl} {"X"=0.0, "b"=0.0, "X^2"=0.0} ("方程系数"), "X"=w266, "b"=w265, "X^2"=w264) -> (w261:cluster{"X":dbl, "b":dbl, "X^2":dbl})
              }
              frame 4 {
                n206 = local read "量程选择"() -> (w282:enum16{"低量程", "高量程", "0-2量程"})
                n207 = case shown="\"高量程\"" w282 {
                  tunnel: w279 -> [w289 w293 w297]
                  tunnel: [w288 w292 w296] -> w285
                  tunnel: [w287 w291 w295] -> w284
                  tunnel: [w286 w290 w294] -> w283
                  frame "低量程", Default {
                    n208 = Unbundle By Name(w289) -> ("数组 2[18]"=w288:sgl, "数组 2[19]"=w287:sgl, "数组 2[20]"=w286:sgl)
                  }
                  frame "高量程" {
                    n209 = Unbundle By Name(w293) -> ("数组 2[21]"=w292:sgl, "数组 2[22]"=w291:sgl, "数组 2[23]"=w290:sgl)
                  }
                  frame "0-2量程" {
                    n210 = Unbundle By Name(w297) -> ("数组 2[6]"=w296:sgl, "数组 2[7]"=w295:sgl, "数组 2[8]"=w294:sgl)
                  }
                }
                n211 = Bundle By Name(cluster=cluster{"X":dbl, "b":dbl, "X^2":dbl} {"X"=0.0, "b"=0.0, "X^2"=0.0} ("方程系数"), "X"=w285, "b"=w284, "X^2"=w283) -> (w280:cluster{"X":dbl, "b":dbl, "X^2":dbl})
              }
              frame 5 {
                n212 = local read "量程选择"() -> (w301:enum16{"低量程", "高量程", "0-2量程"})
                n213 = case shown="\"高量程\"" w301 {
                  tunnel: w298 -> [w308 w312 w316]
                  tunnel: [w307 w311 w315] -> w304
                  tunnel: [w306 w310 w314] -> w303
                  tunnel: [w305 w309 w313] -> w302
                  frame "低量程", Default {
                    n214 = Unbundle By Name(w308) -> ("数组 2[24]"=w307:sgl, "数组 2[25]"=w306:sgl, "数组 2[26]"=w305:sgl)
                  }
                  frame "高量程" {
                    n215 = Unbundle By Name(w312) -> ("数组 2[27]"=w311:sgl, "数组 2[28]"=w310:sgl, "数组 2[29]"=w309:sgl)
                  }
                  frame "0-2量程" {
                    n216 = Unbundle By Name(w316) -> ("数组 2[6]"=w315:sgl, "数组 2[7]"=w314:sgl, "数组 2[8]"=w313:sgl)
                  }
                }
                n217 = Bundle By Name(cluster=cluster{"X":dbl, "b":dbl, "X^2":dbl} {"X"=0.0, "b"=0.0, "X^2"=0.0} ("方程系数"), "X"=w304, "b"=w303, "X^2"=w302) -> (w299:cluster{"X":dbl, "b":dbl, "X^2":dbl})
              }
              frame 6 {
                n218 = local read "量程选择"() -> (w320:enum16{"低量程", "高量程", "0-2量程"})
                n219 = case shown="\"高量程\"" w320 {
                  tunnel: w317 -> [w327 w331 w335]
                  tunnel: [w326 w330 w334] -> w323
                  tunnel: [w325 w329 w333] -> w322
                  tunnel: [w324 w328 w332] -> w321
                  frame "低量程", Default {
                    n220 = Unbundle By Name(w327) -> ("数组 2[30]"=w326:sgl, "数组 2[31]"=w325:sgl, "数组 2[32]"=w324:sgl)
                  }
                  frame "高量程" {
                    n221 = Unbundle By Name(w331) -> ("数组 2[33]"=w330:sgl, "数组 2[34]"=w329:sgl, "数组 2[35]"=w328:sgl)
                  }
                  frame "0-2量程" {
                    n222 = Unbundle By Name(w335) -> ("数组 2[6]"=w334:sgl, "数组 2[7]"=w333:sgl, "数组 2[8]"=w332:sgl)
                  }
                }
                n223 = Bundle By Name(cluster=cluster{"X":dbl, "b":dbl, "X^2":dbl} {"X"=0.0, "b"=0.0, "X^2"=0.0} ("方程系数"), "X"=w323, "b"=w322, "X^2"=w321) -> (w318:cluster{"X":dbl, "b":dbl, "X^2":dbl})
              }
              frame 7 {
                n224 = local read "量程选择"() -> (w339:enum16{"低量程", "高量程", "0-2量程"})
                n225 = case shown="\"高量程\"" w339 {
                  tunnel: w336 -> [w346 w350 w354]
                  tunnel: [w345 w349 w353] -> w342
                  tunnel: [w344 w348 w352] -> w341
                  tunnel: [w343 w347 w351] -> w340
                  frame "低量程", Default {
                    n226 = Unbundle By Name(w346) -> ("数组 2[36]"=w345:sgl, "数组 2[37]"=w344:sgl, "数组 2[38]"=w343:sgl)
                  }
                  frame "高量程" {
                    n227 = Unbundle By Name(w350) -> ("数组 2[39]"=w349:sgl, "数组 2[40]"=w348:sgl, "数组 2[41]"=w347:sgl)
                  }
                  frame "0-2量程" {
                    n228 = Unbundle By Name(w354) -> ("数组 2[6]"=w353:sgl, "数组 2[7]"=w352:sgl, "数组 2[8]"=w351:sgl)
                  }
                }
                n229 = Bundle By Name(cluster=cluster{"X":dbl, "b":dbl, "X^2":dbl} {"X"=0.0, "b"=0.0, "X^2"=0.0} ("方程系数"), "X"=w342, "b"=w341, "X^2"=w340) -> (w337:cluster{"X":dbl, "b":dbl, "X^2":dbl})
              }
            }
            n230 = local write "方程系数"(w217) -> ()
          }
        }
      }
    }
    n231 = flat-sequence {
      frame #0 {
        # "保存参数赋值"
        n232 = Multiply(x="温度", y=10.0) -> (x*y=w139:dbl)
        n233 = Multiply(x="标准液浓度", y=100.0) -> (x*y=w133:dbl)
        n234 = Multiply(x="修正系数", y=100.0) -> (x*y=w136:dbl)
        n235 = Build Array(w139, "恒温时间", w133, w136, "基本量程", "水样", "蒸馏水", "标液", "质控样", "加标回收", "高锰酸钾", "草酸钠", "硫酸", "零点泵计量数 2", "标度泵计量数 2", "高量程稀释倍数:", "低量程稀释倍数:", "CODMn零点核查选择") -> (w130:dbl[])
        n236 = local write "保存参数"(w130) -> ()
      }
    }
    n237 = flat-sequence {
      frame #0 {
        w382 = T9 0 items=["最小二乘", "最小绝对残差", "Bisquare"] ("method")
        # "计算线性、多项式公式"
        n238 = local read "浓度5"() -> (w376:dbl)
        n239 = local read "浓度4"() -> (w377:dbl)
        n240 = local read "浓度2"() -> (w386:dbl)
        n241 = local read "浓度3"() -> (w387:dbl)
        n242 = local read "浓度1"() -> (w385:dbl)
        n243 = Build Array("启用1", "启用2", "启用3", "启用4", "启用5") -> (w370:bool[])
        n244 = Build Array(w385, w386, w387, w377, w376) -> (w384:dbl[])
        n245 = Build Array("泵滴定数1", "泵滴定数2", "泵滴定数3", "泵滴定数4", "泵滴定数5") -> (w383:dbl[])
        n246 = call "线性公式CODMn用.vi"("标液浓度"=w384, "监测浓度"=w383, "启用"=w370, "method"=w382, "模型"="模型", "精度"=6) -> ("拟合方程"=w363:string, "r^2"=→"r^2":dbl, "slope"=w361:dbl, "intercept"=w362:dbl, "XY图"=→"XY图":cluster{"X Values":dbl[], "Y Values":dbl[]}[], "Polynomial Coefficients"=w378:dbl[])  [unwired: 8 in]
        "拟合公式" <- w363
        n247 = feedback-in #2(w363) -> ()
        n248 = feedback #2(w363) -> (w364:string)
        n249 = Not Equal?(x=w363, y=w364) -> (x != y?=w360:bool)
        n250 = case shown="真" w360 {
          tunnel: w378 -> [_ w395]
          tunnel: w362 -> [_ w397]
          tunnel: w361 -> [_ w398]
          frame False {
          }
          frame True {
            # "当公式发生改变时赋值到右侧公式"
            n251 = local read "模型"() -> (w400:enum32{"线性", "多项式"})
            n252 = case shown="\"多项式\"" w400 {
              tunnel: [w405 w407] -> w399
              tunnel: w398 -> [w405 _]
              tunnel: w397 -> [w404 _]
              tunnel: [w404 w408] -> w396
              tunnel: w395 -> [_ w409]
              tunnel: [0.0 ("数值") w406] -> w394
              frame "线性", Default {
              }
              frame "多项式" {
                # "B,K,X^2"
                n253 = Index Array(array=w409) -> (element #1=w408:dbl, element #2=w407:dbl, element #3=w406:dbl)  [unwired: 3 in]
              }
            }
            n254 = Bundle By Name(cluster=cluster{"K":dbl, "b":dbl, "X^2":dbl} {"K"=0.0, "b"=0.0, "X^2"=0.0} ("方程系数"), "K"=w399, "b"=w396, "X^2"=w394) -> (w401:cluster{"K":dbl, "b":dbl, "X^2":dbl})
            n255 = local write "方程系数"(w401) -> ()
          }
        }
        n256 = Unbundle By Name("方程系数") -> ("K"=w357:dbl, "b"=w356:dbl, "X^2"=w355:dbl)
        n257 = case shown="\"多项式\"" "模型" {
          tunnel: w357 -> [w389 w392]
          tunnel: w356 -> [w388 w393]
          tunnel: w355 -> [_ w391]
          frame "线性", Default {
            "K" <- w389
            "b" <- w388
          }
          frame "多项式" {
            n258 = Build Array(w393, w392, w391) -> (→"多项式系数":dbl[])
          }
        }
      }
    }
    n259 = flat-sequence {
      frame #0 {
        # "断电保存全局给局部变量"
        n260 = global read "CODMn断电保存全局变量.vi" "标样核查量程选择"() -> (w471:enum32{"H", "L", "AUTO"})
        n261 = global read "CODMn断电保存全局变量.vi" "零点核查量程选择"() -> (w473:enum32{"H", "L", "AUTO"})
        n262 = global read "CODMn断电保存全局变量.vi" "CODMn跨度量程选择"() -> (w481:enum32{"H", "L", "AUTO"})
        n263 = global read "CODMn断电保存全局变量.vi" "测量模式(公式)"() -> (w482:u16)
        n264 = global read "CODMn断电保存全局变量.vi" "常规版/认证版"() -> (w475:enum16{"常规版", "认证版", "浮台版"})
        n265 = global read "CODMn断电保存全局变量.vi" "自动切换量程:"() -> (w478:enum16{"关闭", "自动切换测一次", "自动切换测两次"})
        n266 = global read "CODMn断电保存全局变量.vi" "零点核查浓度"() -> (w472:dbl)
        n267 = global read "CODMn断电保存全局变量.vi" "高切低阈值:"() -> (w480:dbl)
        n268 = global read "CODMn断电保存全局变量.vi" "低切高阈值:"() -> (w479:dbl)
        n269 = global read "CODMn断电保存全局变量.vi" "标样浓度"() -> (w474:dbl)
        n270 = global read "CODMn断电保存全局变量.vi" "跨度液浓度"() -> (w477:dbl)
        n271 = global read "CODMn断电保存全局变量.vi" "启动时间"() -> (w476:timestamp)
        n272 = local write "标样核查量程选择"(w471) -> ()
        n273 = local write "零点核查量程选择"(w473) -> ()
        n274 = local write "测量模式(公式)"(w482) -> ()
        n275 = local write "零点核查浓度"(w472) -> ()
        n276 = local write "常规版/认证版"(w475) -> ()
        n277 = local write "自动切换量程:"(w478) -> ()
        n278 = local write "跨度量程选择"(w481) -> ()
        n279 = local write "低切高阈值:"(w479) -> ()
        n280 = local write "标样浓度"(w474) -> ()
        n281 = local write "跨度液浓度"(w477) -> ()
        n282 = local write "高切低阈值:"(w480) -> ()
        n283 = local write "启动时间"(w476) -> ()
      }
    }
    n284 = flat-sequence {
      frame #0 {
        # "局部变量给内部交互用全局变量"
        n285 = local read "CODMn工作状态"() -> (w158:T1)
        n286 = local read "COD浓度（mg/L)"() -> (w155:dbl)
        n287 = local read "标准液浓度"() -> (w154:dbl)
        n288 = local read "多列列表框"() -> (w156:i32)
        n289 = local read "故障标记"() -> (w157:bool)
        n290 = global write "COD测量模式全局.vi" "CODMn工作状态"(w158) -> ()
        n291 = global write "COD读取DATA全局.vi" "故障标记"(w157) -> ()
        n292 = global write "运行时序全局变量.vi" "多列列表框"(w156) -> ()
        n293 = global write "COD浓度全局变量.vi" "COD浓度（mg/L)"(w155) -> ()
        n294 = global write "COD浓度全局变量.vi" "标准液浓度"(w154) -> ()
      }
    }
  }
  n295 = while {
    shift-right: [w531] -> _
    shift-left: u16[] [] ("ORP滴定曲线") -> [w532]
    shift-right: [w526] -> _
    shift-left: 0.0 -> [w527]
    stop <- FALSE stop-if-true
    # "滴定数-ORP滴定曲线"
    n296 = local read "多列列表框"() -> (w530:i32)
    n297 = Wait (ms)(milliseconds to wait=u32 300 ("等待时间（毫秒）")) -> ()  [unwired: 1 out]
    n298 = Greater Or Equal?(x=w530, y=4) -> (x >= y?=w528:bool)
    n299 = case shown="真" w528 {
      tunnel: w532 -> [_ w551]
      tunnel: [u16[] [] ("ORP滴定曲线") w550] -> w531
      tunnel: w527 -> [_ w539]
      tunnel: [0.0 w538] -> w526
      frame False {
      }
      frame True {
        n300 = local read "高锰酸钾"() -> (w541:dbl)
        n301 = local read "多列列表框"() -> (w546:i32)
        n302 = local read "ORP显示"() -> (w547:dbl)
        n303 = Less?(x=w539, y=w541) -> (x < y?=w537:bool)
        n304 = Equal?(x=w546, y=5) -> (x = y?=w544:bool)
        n305 = call <vilib>:"Value Has Changed PtByPt.vi"("input data point"=w541) -> ("has changed"=w549:bool, "output data point"=w548:dbl)  [unwired: 1 in]
        n306 = call <vilib>:"Boolean Crossing PtByPt.vi"("direction"=enum16{"either", "false-true", "true-false"}."false-true", "input"=w544) -> ("crossing"=w542:bool)  [unwired: 1 in]
        n307 = Or(x=w537, y=w549) -> (x .or. y?=w540:bool)
        n308 = case shown="真" w540 {
          tunnel: w551 -> [w558 w572]
          tunnel: [w557 w571] -> w550
          tunnel: w548 -> [w559 w565]
          tunnel: w547 -> [w555 w570]
          tunnel: w539 -> [w554 w567]
          tunnel: [w554 w569] -> w538
          tunnel: w537 -> [_ w568]
          frame False {
            n309 = Equal To 0?(x=w559) -> (x = 0?=w556:bool)
            n310 = case shown="真" w556 {
              tunnel: [w560 w563] -> w557
              tunnel: w558 -> [w560 _]
              tunnel: w555 -> [_ w562]
              frame False {
              }
              frame True {
                n311 = Insert Into Array(array=u16[] [] ("ORP滴定曲线"), index=0 ("索引"), new element=w562) -> (w563:u16[])
                n312 = local write "滴定数-ORP值"(w563) -> ()
              }
            }
          }
          frame True {
            # "防止高锰酸钾不连续变大"
            n313 = case shown="假" w568 {
              tunnel: w567 -> [_ w576]
              tunnel: [w575 w576] -> w566
              tunnel: w565 -> [w575 _]
              frame False {
              }
              frame True {
              }
            }
            n314 = Increment(x=w567) -> (x+1=w569:dbl)
            n315 = Insert Into Array(array=w572, index=w566, new element=w570) -> (w571:u16[])
            "滴定数-ORP值" <- w571
            n316 = Insert Into Array(array=u16[] [] ("ORP滴定曲线"), new element=w571) -> (→"ORP滴定曲线":u16[])  [unwired: 1 in]
          }
        }
        n317 = case shown="真" w542 {
          frame False {
          }
          frame True {
            n318 = Get Date/Time In Seconds() -> (seconds since 1Jan1904=w552:timestamp)
            n319 = local write "波形时间"(w552) -> ()
            n320 = local read "ORP滴定曲线"() -> (w553:u16[])
            n321 = call "波形存储(子VI).vi"("ORP滴定曲线"=w553) -> ()  [unwired: 11 in]
          }
        }
      }
    }
  }
  n322 = while {
    shift-right: [w582] -> _
    shift-left: enum16{"待机", "启动COD", "COD测量中", "延时"}."待机" -> [w581]
    stop <- FALSE stop-if-true
    # "定时启动循环"
    n323 = global read "CODMn断电保存全局变量.vi" "定时控制"() -> (w578:T11)
    n324 = Wait (ms)(milliseconds to wait=u32 1000 ("等待时间（毫秒）")) -> ()  [unwired: 1 out]
    n325 = Unbundle By Name(w578) -> ("定时功能启用"=→"定时启动":bool)
    n326 = local read "定时启动"() -> (w579:bool)
    n327 = case shown="真" w579 {
      tunnel: w581 -> [_ w637]
      tunnel: [_ w636] -> w580
      frame False {
      }
      frame True {
        n328 = global read "CODMn断电保存全局变量.vi" "定时控制"() -> (w635:T11)
        n329 = Unbundle By Name(w635) -> ("周期设置类型"=w638:enum16{"定点启动", "间隔启动"}, "定时间隔"=w639:dbl, "24H周期设置"=w640:bool[])  [unwired: 1 out]
        n330 = case shown="\"定点启动\", 默认" w638 {
          tunnel: w639 -> [_ w655]
          tunnel: w640 -> [w643 _]
          tunnel: w637 -> [w641 w658]
          tunnel: [w642 w653] -> w636
          frame "定点启动", Default {
            n331 = case shown="\"待机\", 默认" w641 {
              tunnel: w643 -> [w649 _]
              tunnel: [w644 _] -> w642
              frame "待机", Default {
                n332 = Get Date/Time In Seconds() -> (seconds since 1Jan1904=w651:timestamp)
                n333 = Seconds To Date/Time(time stamp (now)=w651) -> (date time rec=w650:T12)  [unwired: 1 in]
                n334 = Unbundle By Name(w650) -> ("时"=w648:i32, "分"=w647:i32)  [unwired: 1 out]
                n335 = Equal To 0?(x=w647) -> (x = 0?=w645:bool)
                n336 = Index Array(array=w649, index=w648) -> (element=w646:bool)
                n337 = Compound Arithmetic op=AND ("复合运算")(w646, w645) -> (w644:bool)
              }
              frame "启动COD" {
              }
            }
          }
          frame "间隔启动" {
            n338 = Multiply(x=w655, y=60.0) -> (x*y=w652:dbl)
            n339 = feedback #3(w652) -> (w657:dbl)
            n340 = case shown="\"待机\"" w658 {
              tunnel: w657 -> [_ w660]
              tunnel: [_ w659] -> w656
              frame Default {
              }
              frame "待机" {
                n341 = Increment(x=w660) -> (x+1=w659:dbl)
              }
            }
            n342 = feedback-in #3(w656) -> ()
            n343 = Greater Or Equal?(x=w656, y=w652) -> (x >= y?=w653:bool)
          }
        }
      }
    }
    n344 = case shown="\"启动COD\"" w581 {
      tunnel: [w585 w591 w625 enum16{"待机", "启动COD", "COD测量中", "延时"}."待机"] -> w582
      tunnel: w580 -> [w588 _ _ _]
      frame "待机", Default {
        n345 = Select(t=enum16{"待机", "启动COD", "COD测量中", "延时"}."启动COD", s=w588, f=enum16{"待机", "启动COD", "COD测量中", "延时"}."待机") -> (s? t:f=w585:enum16{"待机", "启动COD", "COD测量中", "延时"})
      }
      frame "启动COD" {
        n346 = global read "CODMn断电保存全局变量.vi" "定时控制"() -> (w589:T11)
        n347 = Unbundle By Name(w589) -> ("仪器测试类型"=w590:T13)
        n348 = flat-sequence {
          tunnel: w590 -> [w595]
          tunnel: [enum16{"待机", "启动COD", "COD测量中", "延时"}."COD测量中"] -> w591
          frame #0 {
            n349 = case shown="\"空白测试\"" w595 {
              tunnel: [T10 {"测量模式"=enum."水样测量"} ("启动测量模式") T10 {"测量模式"=enum."标样核查"} ("启动测量模式") T10 {"测量模式"=enum."空白测试"} ("启动测量模式") T10 {"测量模式"=enum."跨度核查"} ("启动测量模式") T10 {"测量模式"=enum."加标回收"} ("启动测量模式") T10 {"测量模式"=enum."平行样"} ("启动测量模式") T10 {"测量模式"=enum."校零"} ("启动测量模式") T10 {"测量模式"=enum."校标"} ("启动测量模式") T10 {"测量模式"=enum."零点核查"} ("启动测量模式")] -> w594
              tunnel: ["水样测试" ("测量模式") "标样核查" ("测量模式") "空白测试" ("测量模式") "跨度核查" ("测量模式") "加标回收" ("测量模式") "平行样" ("测量模式") "校零" ("测量模式") "校标" ("测量模式") "零点核查" ("测量模式")] -> w593
              tunnel: [enum32{"H", "L", "AUTO"}."AUTO" ("CODMn跨度量程选择") w599 enum32{"H", "L", "AUTO"}."L" ("CODMn跨度量程选择") w605 enum32{"H", "L", "AUTO"}."AUTO" ("CODMn跨度量程选择") enum32{"H", "L", "AUTO"}."AUTO" ("CODMn跨度量程选择") enum32{"H", "L", "AUTO"}."L" ("CODMn跨度量程选择") enum32{"H", "L", "AUTO"}."AUTO" ("CODMn跨度量程选择") w620] -> w592
              frame "水样测试", Default {
              }
              frame "标样核查" {
                n350 = local read "标样核查量程选择"() -> (w599:enum32{"H", "L", "AUTO"})
              }
              frame "空白测试" {
              }
              frame "跨度核查" {
                n351 = local read "跨度量程选择"() -> (w605:enum32{"H", "L", "AUTO"})
              }
              frame "加标回收" {
              }
              frame "平行样" {
              }
              frame "校零" {
              }
              frame "校标" {
              }
              frame "零点核查" {
                n352 = local read "零点核查量程选择"() -> (w620:enum32{"H", "L", "AUTO"})
              }
            }
            n353 = global write "COD测量模式全局.vi" "测量模式"(w593) -> ()
            n354 = call "CODMn启动命令 (子VI).vi"("CODMn量程切换"=w592, "启动测量模式"=w594) -> ()  [unwired: 10 in]
          }
          frame #1 {
          }
        }
      }
      frame "COD测量中" {
        n355 = flat-sequence {
          tunnel: [w626] -> w624
          tunnel: [w633] -> w625
          tunnel: w624 -> [w633]
          frame #0 {
            n356 = global read "运行时序全局变量.vi" "多列列表框"() -> (w631:i32)
            n357 = Equal?(x=w631, y=0) -> (x = y?=w629:bool)
            n358 = Select(t=enum16{"待机", "启动COD", "COD测量中", "延时"}."延时", s=w629, f=enum16{"待机", "启动COD", "COD测量中", "延时"}."COD测量中") -> (s? t:f=w626:enum16{"待机", "启动COD", "COD测量中", "延时"})
          }
          frame #1 {
            n359 = Wait (ms)(milliseconds to wait=u32 5000 ("等待时间（毫秒）")) -> ()  [unwired: 1 out]
          }
        }
      }
      frame "延时" {
      }
    }
  }
  n360 = while {
    stop <- FALSE stop-if-true
    # "相差60秒自动校时"
    n361 = local read "仪器时间"() -> (w664:timestamp)
    n362 = local read "系统时间"() -> (w665:timestamp)
    n363 = Build Array(w664) -> (w663:timestamp[])
    n364 = call "DateToHex.vi"("DATE"=w663) -> ("数组"=w676:u16[])  [unwired: 10 in]
    n365 = Build Array(w665) -> (w682:timestamp[])
    n366 = call "DateToHex.vi"("DATE"=w682) -> ("数组"=w681:u16[])  [unwired: 10 in]
    n367 = Index Array(array=w676, index=2 ("索引")) -> (element=w678:u16)
    n368 = Index Array(array=w681, index=2 ("索引")) -> (element=w679:u16)
    n369 = Split Number(x=w678) -> (hi(x)=w672:u8)  [unwired: 1 out]
    n370 = Split Number(x=w679) -> (hi(x)=w675:u8)  [unwired: 1 out]
    n371 = To Byte Integer(number=w672) -> (8bit integer=w671:i8)
    n372 = To Byte Integer(number=w675) -> (8bit integer=w674:i8)
    n373 = Subtract(x=w671, y=w674) -> (x-y=w673:i8)
    n374 = local read "通讯状态"() -> (w667:bool)
    n375 = Absolute Value(x=w673) -> (abs(x)=w670:i8)
    n376 = Wait (ms)(milliseconds to wait=u32 1000 ("等待时间（毫秒）")) -> ()  [unwired: 1 out]
    n377 = Greater Or Equal?(x=w670, y=i8 60) -> (x >= y?=w668:bool)
    n378 = And(x=w668, y=w667) -> (x .and. y?=w666:bool)
    n379 = case shown="真" w666 {
      frame False {
      }
      frame True {
        # "相差60秒时间自动校准"
        n380 = flat-sequence {
          frame #0 {
            n381 = property on="时间校准" class="Bool (严格)"("Val(Sgnl)"=TRUE ("值(信号)")) -> ()  [unwired: 2 in, 2 out]
          }
          frame #1 {
            n382 = Wait (ms)(milliseconds to wait=u32 500 ("等待时间（毫秒）")) -> ()  [unwired: 1 out]
          }
          frame #2 {
            n383 = property on="时间校准" class="Bool (严格)"("Val(Sgnl)"=FALSE ("值(信号)")) -> ()  [unwired: 2 in, 2 out]
          }
        }
      }
    }
  }
  n384 = while {
    stop <- FALSE stop-if-true
    # "存储数据入队列、日志存储、报警存储"
    n385 = local read "多列列表框"() -> (w686:i32)
    n386 = First Call?() -> (First Call?: T/F=w689:bool)
    n387 = local read "报警簇"() -> (w690:T2)
    n388 = Not(x=w689) -> (.not. x?=w687:bool)
    n389 = call "CODMn报警信息.vi"("报警簇"=w690) -> ("CODMN报警信息"=w691:string)  [unwired: 10 in]
    n390 = case shown="真" w687 {
      selector: w687 -> [w714 _]
      tunnel: w686 -> [_ w716]
      tunnel: [w714 w715] -> w688
      frame False {
      }
      frame True {
        # "非初次调用"
        n391 = Greater?(x=w716, y=u16 0) -> (0:w719:bool)
        n392 = call <vilib>:"Boolean Crossing PtByPt.vi"("direction"=enum16{"either", "false-true", "true-false"}."false-true", "input"=w719) -> ("crossing"=w715:bool)  [unwired: 1 in]
      }
    }
    n393 = feedback #4(w686) -> (w702:i32)
    n394 = feedback-in #4(w686) -> ()
    n395 = Greater?(x=w686, y=u16 0) -> (0:w713:bool)
    n396 = Less Or Equal?(x=w686, y=u16 5) -> (x <= y?=w710:bool)
    n397 = local read "断电排液标记"() -> (w698:bool)
    n398 = feedback #5(w691) -> (w692:string)
    n399 = feedback-in #5(w691) -> ()
    n400 = Not Equal?(x=w691, y="") -> (x != y?=w696:bool)
    n401 = Equal?(x=w686, y=u16 5) -> (x = y?=w706:bool)
    n402 = Not Equal?(x=w686, y=w702) -> (x != y?=w703:bool)
    n403 = Not Equal?(x=w691, y=w692) -> (x != y?=w693:bool)
    n404 = And(x=w713, y=w710) -> (x .and. y?=w711:bool)
    n405 = call <vilib>:"Boolean Crossing PtByPt.vi"("direction"=enum16{"either", "false-true", "true-false"}."false-true", "input"=w706) -> ("crossing"=w708:bool)  [unwired: 1 in]
    n406 = And(x=w693, y=w696) -> (x .and. y?=w694:bool)
    n407 = call <vilib>:"Boolean Crossing PtByPt.vi"("direction"=enum16{"either", "false-true", "true-false"}."false-true", "input"=w698) -> ("crossing"=w697:bool)  [unwired: 1 in]
    n408 = First Call?() -> (First Call?: T/F=w704:bool)
    n409 = case shown="假" w704 {
      tunnel: w703 -> [w742 _]
      tunnel: w686 -> [w741 _]
      frame False {
        # "初次调用不存日志，防止软件重启重复存储日志"
        n410 = case shown="真" w742 {
          tunnel: w741 -> [_ w744]
          frame False {
          }
          frame True {
            # "步骤发生改变存储日志"
            n411 = flat-sequence {
              tunnel: w744 -> [w745]
              tunnel: [w745] -> w743
              tunnel: w743 -> [w765]
              frame #0 {
                n412 = case shown="1" w745 {
                  frame 0 {
                    n413 = global read "COD测量模式全局.vi" "测量模式"() -> (w752:string)
                    n414 = Concatenate Strings("-->", w752, "结束" ("字符串")) -> (w751:string)
                    n415 = call "CODMn日志存储 (子VI).vi"("table输入"="操作日志", "参数"="CODMn" ("table输入"), "日志信息"=w751, "database"="database3.mdb") -> ()  [unwired: 8 in]
                  }
                  frame 1 {
                    n416 = property on="CODMn工作状态" class="Enum (严格)"() -> ("RingText.Text"=w755:string)  [unwired: 2 in, 2 out]
                    n417 = Concatenate Strings("-->", w755, "启动" ("字符串")) -> (w753:string)
                    n418 = call "CODMn日志存储 (子VI).vi"("table输入"="操作日志", "参数"="CODMn" ("table输入"), "日志信息"=w753, "database"="database3.mdb") -> ()  [unwired: 8 in]
                  }
                  frame 2, Default {
                  }
                }
              }
              frame #1 {
                n419 = property on="多列列表框" class="MCListbox (严格)"() -> ("ItemNames"=w763:string[][])  [unwired: 2 in, 2 out]
                n420 = Index Array(array=w763, index (row)=w765) -> (element=w762:string[])  [unwired: 1 in]
                n421 = Index Array(array=w762, index=0 ("索引")) -> (element=w760:string)
                n422 = call "CODMn日志存储 (子VI).vi"("table输入"="操作日志", "参数"="CODMn" ("table输入"), "日志信息"=w760, "database"="database3.mdb") -> ()  [unwired: 8 in]
              }
            }
          }
        }
      }
      frame True {
      }
    }
    n423 = case shown="真" w697 {
      frame False {
      }
      frame True {
        n424 = Get Date/Time In Seconds() -> (seconds since 1Jan1904=w735:timestamp)
        n425 = Bundle(cluster=T15 {"时间标识"=timestamp(0 s since 1904-01-01), "参数"="", "日志信息"="", "流程参数"=""} ("data in"), "时间标识"=w735, "参数"="CODMn" ("table输入"), "日志信息"="断电排液", "流程参数"="" ("table输入")) -> (w733:T15)
        n426 = call "流程日志字段定义.vi"("table输入"="操作日志", "data in"=w733) -> ("table输出"=w738:string, "columns"=w739:string[], "data out"=w740:T16)  [unwired: 7 in]
        n427 = call "插入数据.vi"("data"=w740, "columns"=w739, "database"="database3.mdb", "table"=w738) -> ()  [unwired: 7 in, 1 out]
      }
    }
    n428 = case shown="真" w694 {
      tunnel: w691 -> [_ w720]
      frame False {
      }
      frame True {
        n429 = Get Date/Time In Seconds() -> (seconds since 1Jan1904=w722:timestamp)
        n430 = Bundle By Name(cluster=T14 {"时间标识"=timestamp(0 s since 1904-01-01), "设备"="", "日志信息"=""} ("data in"), "时间标识"=w722, "设备"="CODMn", "日志信息"=w720) -> (w723:T14)
        n431 = call "报警信息字段定义.vi"("table输入"="报警信息", "data in"=w723) -> ("table输出"=w727:string, "columns"=w728:string[], "data out"=w729:T14)  [unwired: 7 in]
        n432 = call "插入数据.vi"("data"=w729, "columns"=w728, "database"="database3.mdb", "table"=w727) -> ()  [unwired: 7 in, 1 out]
      }
    }
    n433 = case shown="真" w711 {
      frame False {
      }
      frame True {
        # "测量过程中记录测量模式，为存储数据做准备，待机状态变量不更新"
        n434 = flat-sequence {
          frame #0 {
            n435 = local read "标样核查标记"() -> (w793:bool)
            n436 = local read "零点核查标记"() -> (w792:bool)
            n437 = local read "跨度核查标记"() -> (w790:bool)
            n438 = local read "空白测试标记"() -> (w789:bool)
            n439 = local read "加标回收测量"() -> (w788:bool)
            n440 = local read "平行样测量"() -> (w787:bool)
            n441 = local read "水样测量"() -> (w794:bool)
            n442 = local read "校零标记"() -> (w786:bool)
            n443 = local read "校标标记"() -> (w785:bool)
            n444 = Build Array(w794, w793, w792, w790, w789, w788, w787, w786, w785) -> (w791:bool[])
            n445 = for {
              tunnel: w791 -> [w796] mode=indexing
              i -> [w795]
              n446 = case shown="真" w796 {
                tunnel: w795 -> [_ w797]
                frame False {
                }
                frame True {
                  "测量模式数字" <- w797
                }
              }
            }
          }
          frame #1 {
            n447 = local read "测量模式数字"() -> (w800:i32)
            n448 = local read "启动时间"() -> (w798:timestamp)
            n449 = case shown="6" w800 {
              tunnel: ["水样测试" ("测量模式") "标样核查" ("测量模式") "零点核查" ("测量模式") "跨度核查" ("测量模式") "空白测试" ("测量模式") "加标回收" ("测量模式") "平行样" ("测量模式") "校零" ("测量模式") "校标" ("测量模式")] -> w799
              tunnel: w798 -> [w801 _ _ _ _ w807 _ _ _]
              frame 0, Default {
                n450 = global write "COD测量模式全局.vi" "水样启动时间"(w801) -> ()
              }
              frame 1 {
              }
              frame 2 {
              }
              frame 3 {
              }
              frame 4 {
              }
              frame 5 {
                n451 = global write "COD测量模式全局.vi" "加标回收启动时间"(w807) -> ()
              }
              frame 6 {
              }
              frame 7 {
              }
              frame 8 {
              }
            }
            n452 = global write "COD测量模式全局.vi" "测量模式"(w799) -> ()
          }
        }
      }
    }
    n453 = case shown="真" w688 {
      frame False {
      }
      frame True {
        # "非初次调用记录启动时间"
        n454 = flat-sequence {
          frame #0 {
            n455 = local read "切换量程连续测两次"() -> (w768:bool)
            n456 = case shown="假" w768 {
              frame False {
                n457 = Get Date/Time In Seconds() -> (seconds since 1Jan1904=w769:timestamp)
                "启动时间" <- w769
                n458 = global write "CODMn断电保存全局变量.vi" "启动时间"(w769) -> ()
              }
              frame True {
                n459 = local write "切换量程连续测两次"(FALSE ("切换量程连续测两次")) -> ()
              }
            }
          }
          frame #1 {
            n460 = global read "COD读取DATA全局.vi" "配置文件ini"() -> (w771:string)
            n461 = call <vilib>:"Application Directory.vi"() -> ("Application Directory"=w784:path)
            n462 = Build Path(base path=w784, name or relative path=w771) -> (appended path=w783:path)
            n463 = call <vilib>:"Open Config Data.vi"("configuration file path"=w783) -> ("error out"=w779:errorcluster, "refnum"=w782:T7)  [unwired: 8 in, 1 out]
            n464 = vi-ref "斯坦道CODMn.lvlib:CODMn断电保存全局变量.vi"() -> (w781:refnum<vi>)
            n465 = call <userlib>:"Write Panel to INI__ogtk.vi"("error in (no error)"=w779, "VI ref"=w781, "refnum"=w782) -> ("error out"=w778:errorcluster, "refnum out"=w780:T7)  [unwired: 7 in]
            n466 = call <vilib>:"Close Config Data.vi"("error in (no error)"=w778, "refnum"=w780) -> ("error out"=w773:errorcluster, "file path"=w772:path)  [unwired: 8 in]
            n467 = Open/Create/Replace File(file path (use dialog)=w772, error in=w773) -> (refnum out=w776:refnum<file>, error out=w777:errorcluster)  [unwired: 4 in, 1 out]
            n468 = Flush File(refnum=w776, error in=w777) -> (refnum out=w775:refnum<file>, error out=w774:errorcluster)
            n469 = Close File(refnum=w775, error in=w774) -> ()  [unwired: 2 out]
          }
        }
      }
    }
    n470 = case shown="真" w708 {
      frame False {
      }
      frame True {
        # "排液步骤存数据，第5步数据存储时间戳更新，防止启动停止数据存储"
        n471 = call "数据写入入队列 (子VI).vi"() -> ()  [unwired: 12 in]
        n472 = global read "CODMn断电保存全局变量.vi" "启动时间"() -> (w817:timestamp)
        n473 = local read "温度"() -> (w812:dbl)
        n474 = global write "COD读取DATA全局.vi" "温度存储数据用"(w812) -> ()
        n475 = global write "COD读取DATA全局.vi" "数据存储时间戳"(w817) -> ()
        n476 = global read "COD测量模式全局.vi" "测量模式"() -> (w816:string)
        n477 = local read "高锰酸钾"() -> (w813:dbl)
        n478 = Equal?(x=w816, y="校标") -> (x = y?=w814:bool)
        n479 = case shown="真" w814 {
          tunnel: w813 -> [_ w818]
          frame False {
          }
          frame True {
            n480 = local read "当前校准"() -> (w819:i32)
            n481 = case shown="3" w819 {
              tunnel: w818 -> [w820 w821 w822 w823 w824]
              frame 1, Default {
                n482 = local write "泵滴定数1"(w820) -> ()
              }
              frame 2 {
                n483 = local write "泵滴定数2"(w821) -> ()
              }
              frame 3 {
                n484 = local write "泵滴定数3"(w822) -> ()
              }
              frame 4 {
                n485 = local write "泵滴定数4"(w823) -> ()
              }
              frame 5 {
                n486 = local write "泵滴定数5"(w824) -> ()
              }
            }
          }
        }
      }
    }
    n487 = Wait (ms)(milliseconds to wait=u32 1000 ("等待时间（毫秒）")) -> ()  [unwired: 1 out]
  }
  n488 = while {
    stop <- FALSE stop-if-true
    # "数字键盘输入"
    n489 = event shown="[22] \"跨度液浓度\", \"零点核查浓度\", \"标样浓度\": 鼠标按下" {
      selector: _ -> [_ _ _ _ _ _ _ _ _ _ _ _ _ _ _ _ _ _ _ _ _ _ _ _ _ _ _ _ _]
      dyn-events: _ -> [_ _ _ _ _ _ _ _ _ _ _ _ _ _ _ _ _ _ _ _ _ _ _ _ _ _ _ _ _]
      timeout: _ -> [_ _ _ _ _ _ _ _ _ _ _ _ _ _ _ _ _ _ _ _ _ _ _ _ _ _ _ _ _]
      event Timeout {
        n490 = event-data() -> ()  [unwired: 1 in, 3 out]
      }
      event "温度": Mouse Down {
        n491 = event-data() -> ()  [unwired: 1 in, 8 out]
        n492 = local read "温度"() -> (w827:dbl)
        n493 = call "数字键盘.vi"("OldNumber"=w827) -> ("NewNumber"=w826:sgl)
        n494 = local write "温度"(w826) -> ()
      }
      event "恒温时间": Mouse Down {
        n495 = event-data() -> ()  [unwired: 1 in, 8 out]
        n496 = local read "恒温时间"() -> (w828:dbl)
        n497 = call "数字键盘.vi"("OldNumber"=w828) -> ("NewNumber"=w829:sgl)
        n498 = local write "恒温时间"(w829) -> ()
      }
      event "标准液浓度": Mouse Down {
        n499 = event-data() -> ()  [unwired: 1 in, 8 out]
        n500 = local read "标准液浓度"() -> (w831:dbl)
        n501 = call "数字键盘.vi"("OldNumber"=w831) -> ("NewNumber"=w830:sgl)
        n502 = local write "标准液浓度"(w830) -> ()
      }
      event "修正系数": Mouse Down {
        n503 = event-data() -> ()  [unwired: 1 in, 8 out]
        n504 = local read "修正系数"() -> (w832:dbl)
        n505 = call "数字键盘.vi"("OldNumber"=w832) -> ("NewNumber"=w833:sgl)
        n506 = local write "修正系数"(w833) -> ()
      }
      event "水样": Mouse Down {
        n507 = event-data() -> ()  [unwired: 1 in, 8 out]
        n508 = local read "水样"() -> (w834:dbl)
        n509 = call "数字键盘.vi"("OldNumber"=w834) -> ("NewNumber"=w835:sgl)
        n510 = local write "水样"(w835) -> ()
      }
      event "蒸馏水": Mouse Down {
        n511 = event-data() -> ()  [unwired: 1 in, 8 out]
        n512 = local read "蒸馏水"() -> (w836:dbl)
        n513 = call "数字键盘.vi"("OldNumber"=w836) -> ("NewNumber"=w837:sgl)
        n514 = local write "蒸馏水"(w837) -> ()
      }
      event "标液": Mouse Down {
        n515 = event-data() -> ()  [unwired: 1 in, 8 out]
        n516 = local read "标液"() -> (w838:dbl)
        n517 = call "数字键盘.vi"("OldNumber"=w838) -> ("NewNumber"=w839:sgl)
        n518 = local write "标液"(w839) -> ()
      }
      event "质控样": Mouse Down {
        n519 = event-data() -> ()  [unwired: 1 in, 8 out]
        n520 = local read "质控样"() -> (w840:dbl)
        n521 = call "数字键盘.vi"("OldNumber"=w840) -> ("NewNumber"=w841:sgl)
        n522 = local write "质控样"(w841) -> ()
      }
      event "加标回收": Mouse Down {
        n523 = event-data() -> ()  [unwired: 1 in, 8 out]
        n524 = local read "加标回收"() -> (w842:dbl)
        n525 = call "数字键盘.vi"("OldNumber"=w842) -> ("NewNumber"=w843:sgl)
        n526 = local write "加标回收"(w843) -> ()
      }
      event "草酸钠": Mouse Down {
        n527 = event-data() -> ()  [unwired: 1 in, 8 out]
        n528 = local read "草酸钠"() -> (w844:dbl)
        n529 = call "数字键盘.vi"("OldNumber"=w844) -> ("NewNumber"=w845:sgl)
        n530 = local write "草酸钠"(w845) -> ()
      }
      event "高锰酸钾": Mouse Down {
        n531 = event-data() -> ()  [unwired: 1 in, 8 out]
        n532 = local read "高锰酸钾"() -> (w846:dbl)
        n533 = call "数字键盘.vi"("OldNumber"=w846) -> ("NewNumber"=w847:sgl)
        n534 = local write "高锰酸钾"(w847) -> ()
      }
      event "硫酸": Mouse Down {
        n535 = event-data() -> ()  [unwired: 1 in, 8 out]
        n536 = local read "硫酸"() -> (w848:dbl)
        n537 = call "数字键盘.vi"("OldNumber"=w848) -> ("NewNumber"=w849:sgl)
        n538 = local write "硫酸"(w849) -> ()
      }
      event "零点泵计量数 2": Mouse Down {
        n539 = event-data() -> ()  [unwired: 1 in, 8 out]
        n540 = local read "零点泵计量数 2"() -> (w850:dbl)
        n541 = call "数字键盘.vi"("OldNumber"=w850) -> ("NewNumber"=w851:sgl)
        n542 = local write "零点泵计量数 2"(w851) -> ()
      }
      event "标度泵计量数 2": Mouse Down {
        n543 = event-data() -> ()  [unwired: 1 in, 8 out]
        n544 = local read "标度泵计量数 2"() -> (w852:dbl)
        n545 = call "数字键盘.vi"("OldNumber"=w852) -> ("NewNumber"=w853:sgl)
        n546 = local write "标度泵计量数 2"(w853) -> ()
      }
      event "高量程稀释倍数:": Mouse Down {
        n547 = event-data() -> ()  [unwired: 1 in, 8 out]
        n548 = local read "高量程稀释倍数:"() -> (w855:i8)
        n549 = call "数字键盘.vi"("OldNumber"=w855) -> ("NewNumber"=w854:sgl)
        n550 = local write "高量程稀释倍数:"(w854) -> ()
      }
      event "低量程稀释倍数:": Mouse Down {
        n551 = event-data() -> ()  [unwired: 1 in, 8 out]
        n552 = local read "低量程稀释倍数:"() -> (w857:i8)
        n553 = call "数字键盘.vi"("OldNumber"=w857) -> ("NewNumber"=w856:sgl)
        n554 = local write "低量程稀释倍数:"(w856) -> ()
      }
      event "浓度1": Mouse Down {
        n555 = event-data() -> ()  [unwired: 1 in, 8 out]
        n556 = local read "浓度1"() -> (w859:dbl)
        n557 = call "数字键盘.vi"("OldNumber"=w859) -> ("NewNumber"=w858:sgl)
        n558 = property on="浓度1" class="DigNum (严格)"("Val(Sgnl)"=w858) -> ()  [unwired: 2 in, 2 out]
      }
      event "浓度2": Mouse Down {
        n559 = event-data() -> ()  [unwired: 1 in, 8 out]
        n560 = local read "浓度2"() -> (w861:dbl)
        n561 = call "数字键盘.vi"("OldNumber"=w861) -> ("NewNumber"=w860:sgl)
        n562 = property on="浓度2" class="DigNum (严格)"("Val(Sgnl)"=w860) -> ()  [unwired: 2 in, 2 out]
      }
      event "浓度3": Mouse Down {
        n563 = event-data() -> ()  [unwired: 1 in, 8 out]
        n564 = local read "浓度3"() -> (w863:dbl)
        n565 = call "数字键盘.vi"("OldNumber"=w863) -> ("NewNumber"=w862:sgl)
        n566 = property on="浓度3" class="DigNum (严格)"("Val(Sgnl)"=w862) -> ()  [unwired: 2 in, 2 out]
      }
      event "浓度4": Mouse Down {
        n567 = event-data() -> ()  [unwired: 1 in, 8 out]
        n568 = local read "浓度4"() -> (w865:dbl)
        n569 = call "数字键盘.vi"("OldNumber"=w865) -> ("NewNumber"=w864:sgl)
        n570 = property on="浓度4" class="DigNum (严格)"("Val(Sgnl)"=w864) -> ()  [unwired: 2 in, 2 out]
      }
      event "浓度5": Mouse Down {
        n571 = event-data() -> ()  [unwired: 1 in, 8 out]
        n572 = local read "浓度5"() -> (w867:dbl)
        n573 = call "数字键盘.vi"("OldNumber"=w867) -> ("NewNumber"=w866:sgl)
        n574 = property on="浓度5" class="DigNum (严格)"("Val(Sgnl)"=w866) -> ()  [unwired: 2 in, 2 out]
      }
      event "跨度液浓度", "零点核查浓度", "标样浓度": Mouse Down {
        n575 = event-data() -> ("CtlRef"=w871:refnum<vi>)  [unwired: 1 in, 7 out]
        n576 = property class="DigNum (严格)"(reference=w871) -> (reference out=w868:refnum<vi>, "Value"=w870:dbl)  [unwired: 1 in, 1 out]
        n577 = call "数字键盘.vi"("OldNumber"=w870) -> ("NewNumber"=w869:sgl)
        n578 = property class="DigNum (严格)"(reference=w868, "Val(Sgnl)"=w869) -> ()  [unwired: 1 in, 2 out]
      }
      event "泵滴定数1": Mouse Down {
        n579 = event-data() -> ()  [unwired: 1 in, 8 out]
        n580 = local read "泵滴定数1"() -> (w873:dbl)
        n581 = call "数字键盘.vi"("OldNumber"=w873) -> ("NewNumber"=w872:sgl)
        n582 = property on="泵滴定数1" class="DigNum (严格)"("Val(Sgnl)"=w872) -> ()  [unwired: 2 in, 2 out]
      }
      event "泵滴定数2": Mouse Down {
        n583 = event-data() -> ()  [unwired: 1 in, 8 out]
        n584 = local read "泵滴定数2"() -> (w875:dbl)
        n585 = call "数字键盘.vi"("OldNumber"=w875) -> ("NewNumber"=w874:sgl)
        n586 = property on="泵滴定数2" class="DigNum (严格)"("Val(Sgnl)"=w874) -> ()  [unwired: 2 in, 2 out]
      }
      event "泵滴定数3": Mouse Down {
        n587 = event-data() -> ()  [unwired: 1 in, 8 out]
        n588 = local read "泵滴定数3"() -> (w877:dbl)
        n589 = call "数字键盘.vi"("OldNumber"=w877) -> ("NewNumber"=w876:sgl)
        n590 = property on="泵滴定数3" class="DigNum (严格)"("Val(Sgnl)"=w876) -> ()  [unwired: 2 in, 2 out]
      }
      event "泵滴定数4": Mouse Down {
        n591 = event-data() -> ()  [unwired: 1 in, 8 out]
        n592 = local read "泵滴定数4"() -> (w879:dbl)
        n593 = call "数字键盘.vi"("OldNumber"=w879) -> ("NewNumber"=w878:sgl)
        n594 = property on="泵滴定数4" class="DigNum (严格)"("Val(Sgnl)"=w878) -> ()  [unwired: 2 in, 2 out]
      }
      event "泵滴定数5": Mouse Down {
        n595 = event-data() -> ()  [unwired: 1 in, 8 out]
        n596 = local read "泵滴定数5"() -> (w881:dbl)
        n597 = call "数字键盘.vi"("OldNumber"=w881) -> ("NewNumber"=w880:sgl)
        n598 = property on="泵滴定数5" class="DigNum (严格)"("Val(Sgnl)"=w880) -> ()  [unwired: 2 in, 2 out]
      }
      event "低切高阈值:", "高切低阈值:": Mouse Down {
        n599 = event-data() -> ("CtlRef"=w885:refnum<vi>)  [unwired: 1 in, 7 out]
        n600 = property class="DigNum (严格)"(reference=w885) -> (reference out=w884:refnum<vi>, "Value"=w883:dbl)  [unwired: 1 in, 1 out]
        n601 = call "数字键盘.vi"("OldNumber"=w883) -> ("NewNumber"=w882:sgl)
        n602 = property class="DigNum (严格)"(reference=w884, "Val(Sgnl)"=w882) -> ()  [unwired: 1 in, 2 out]
      }
    }
  }
  n603 = flat-sequence {
    tunnel: [w890] -> w8
    tunnel: [errorcluster {"status"=FALSE, "code"=0, "source"=""} ("错误输出")] -> w1
    frame #0 {
      n604 = global read "COD读取DATA全局.vi" "序列号:"() -> (w887:string)
      "序列号" <- w887
      n605 = property on="窗格" class="Pane"("Origin"=T17 {"Horizontal"=0, "Vertical"=0} ("原点")) -> ()  [unwired: 2 in, 2 out]
      n606 = Empty String/Path?(string/path=w887) -> (empty?=w889:bool)
      n607 = case shown="真" w889 {
        tunnel: w887 -> [w907 _]
        tunnel: [w906 "data\\Set.ini" ("名称或相对路径")] -> w888
        frame False {
          # "与生产用上位机交互"
          n608 = Concatenate Strings("data\\" ("字符串"), "序列号" ("字符串"), w907, "Set.ini" ("名称或相对路径")) -> (w906:string)
        }
        frame True {
        }
      }
      n609 = call <vilib>:"Application Directory.vi"() -> ("Application Directory"=w899:path)
      n610 = local write "量程切换次数"(u8 0 ("量程切换次数")) -> ()
      n611 = local write "切换量程连续测两次"(FALSE ("切换量程连续测两次")) -> ()
      n612 = Build Path(base path=w899, name or relative path=w888) -> (appended path=w898:path)
      n613 = call <vilib>:"Open Config Data.vi"("configuration file path"=w898) -> ("error out"=w894:errorcluster, "refnum"=w897:T7)  [unwired: 8 in, 1 out]
      n614 = vi-ref "斯坦道CODMn.lvlib:CODMn断电保存全局变量.vi"() -> (w896:refnum<vi>)
      n615 = call <userlib>:"Read Panel from INI__ogtk.vi"("error in (no error)"=w894, "VI ref"=w896, "refnum"=w897) -> ("error out"=w893:errorcluster, "refnum out"=w895:T7)  [unwired: 7 in]
      n616 = call <vilib>:"Close Config Data.vi"("error in (no error)"=w893, "refnum"=w895) -> ("error out"=w892:errorcluster, "file path"=w891:path)  [unwired: 8 in]
      n617 = global write "COD读取DATA全局.vi" "配置文件ini"(w888) -> ()
      n618 = local write "选用水样"(enum16{"葡萄糖", "草酸钠"}."葡萄糖" ("选用水样")) -> ()
      n619 = local write "量程选择"(enum16{"低量程", "高量程", "0-2量程"}."低量程" ("量程选择")) -> ()
      n620 = Open/Create/Replace File(file path (use dialog)=w891, error in=w892) -> (error out=w890:errorcluster)  [unwired: 4 in, 2 out]
      "稀释倍数解释" <- "稀释倍数解释：\n稀释倍数选择1，表示不稀释\n默认低量程系数倍数1，高量程系数倍数2\n则低量程为0~8，高量程为0~16" ("稀释倍数解释")
    }
  }
  n621 = vi-ref "CODMn通讯.vi"() -> (w7:refnum<vi>)
  n622 = property class="VI"(reference=w7, error in=w1) -> ("Name"=w9:string)  [unwired: 2 out]
  n623 = Open VI Reference(type specifier VI Refnum (for type only)=refnum<vi> refnum, vi path=w9, options=128 ("选项")) -> (vi reference=w11:refnum<vi>, error out=w13:errorcluster)  [unwired: 3 in]
  n624 = call-by-ref "?"(reference=w11, error in=w13) -> (reference out=w15:refnum<vi>, error out=w14:errorcluster)  [unwired: 12 in]
  n625 = Close Reference(reference=w15, error in (no error)=w14) -> ()  [unwired: 1 out]
  n626 = Obtain Queue(name (unnamed)="CODMn外部交互" ("名称（未命名）"), element data type=T3 {"命令"="启动命令", "测量模式"=enum."水样测量", "CODMn量程切换"=enum."AUTO"} ("元素")) -> (queue out=w3:refnum<queue>, error out=w2:errorcluster)  [unwired: 3 in, 1 out]
  n627 = Obtain Queue(name (unnamed)="CODMn" ("名称（未命名）"), element data type=cluster{"命令":string} {"命令"="启用模块"} ("元素")) -> (queue out=w17:refnum<queue>, error out=w16:errorcluster)  [unwired: 3 in, 1 out]
  n628 = while {
    tunnel: w17 -> [w913]
    tunnel: w16 -> [w912]
    stop <- FALSE stop-if-true
    # "主线事件"
    n629 = event shown="[25] \"一键写入\": 值改变" {
      selector: _ -> [_ _ _ _ _ _ _ _ _ _ _ _ _ _ _ _ _ _ _ _ _ _ _ _ _ _ _ _ _ _ _]
      dyn-events: _ -> [_ _ _ _ _ _ _ _ _ _ _ _ _ _ _ _ _ _ _ _ _ _ _ _ _ _ _ _ _ _ _]
      timeout: _ -> [_ _ _ _ _ _ _ _ _ _ _ _ _ _ _ _ _ _ _ _ _ _ _ _ _ _ _ _ _ _ _]
      tunnel: w913 -> [_ _ _ _ _ w970 _ _ _ _ _ _ _ _ _ _ _ _ _ _ _ _ _ w1569 _ _ _ _ w1787 w1794 _]
      tunnel: w912 -> [_ _ _ _ _ w969 _ _ _ _ _ _ _ _ _ _ _ _ _ _ _ _ _ w1568 _ _ _ _ w1786 w1793 _]
      event "单步启动": Mouse Down {
        n630 = event-data() -> ()  [unwired: 1 in, 8 out]
        n631 = call "CODMn手动控制框.vi"() -> ()  [unwired: 12 in]
      }
      event "启动": Mouse Down {
        n632 = event-data() -> ()  [unwired: 1 in, 8 out]
        n633 = flat-sequence {
          tunnel: [w916] -> w915
          tunnel: w915 -> [w922]
          frame #0 {
            n634 = call "启动测量模式选择对话框.vi"() -> ("启动选择 2"=w916:u16)  [unwired: 11 in]
            "启动选择 2" <- w916
          }
          frame #1 {
            n635 = case shown="9, 默认" w922 {
              tunnel: [u16 4608 ("address") u16 4608 ("address") u16 4608 ("address") u16 4608 ("address") u16 4608 ("address") u16 4608 ("address") u16 4608 ("address") u16 4608 ("address") u16 4608 ("address") u16 4608 ("address")] -> w918
              tunnel: [u16 1 ("address") u16 2 ("address") u16 3 ("address") u16 4 ("address") u16 5 ("address") u16 7 ("address") u16 6 ("address") u16 8 ("address") u16 9 ("address") u16 0 ("address")] -> w923
              frame 0 {
              }
              frame 1 {
              }
              frame 2 {
              }
              frame 3 {
              }
              frame 4 {
              }
              frame 5 {
              }
              frame 6 {
              }
              frame 7 {
              }
              frame 8 {
              }
              frame 9, Default {
              }
            }
            n636 = Not Equal?(x=w922, y=u16 9) -> (x != y?=w920:bool)
            n637 = global write "CODMN外部API.vi" "手动启动CODMn"(w920) -> ()
            n638 = Insert Into Array(array=u16[] [] ("values"), index=0 ("索引"), new element=w923) -> (w917:u16[])
            n639 = call "CODMnMB_api.vi"("STEP"=enum16{"open", "read", "write", "close"}."write", "values"=w917, "starting address"=w918) -> ()  [unwired: 6 in, 3 out]
          }
        }
      }
      event "停止": Value Change {
        n640 = event-data() -> ()  [unwired: 1 in, 6 out]
        n641 = Two Button Dialog(message="确认是否停止？" ("消息"), 1:"否" ("F按钮名称（“取消”）"), 2:"是" ("T按钮名称（“确定”）")) -> (T button?=w948:bool)
        n642 = case shown="真" w948 {
          frame False {
          }
          frame True {
            n643 = call "CODMnMB_api.vi"("STEP"=enum16{"open", "read", "write", "close"}."write", "values"=u16[] [11], "starting address"=u16 4608) -> ()  [unwired: 6 in, 3 out]
          }
        }
      }
      event "手动控制": Value Change {
        n644 = event-data() -> ()  [unwired: 1 in, 6 out]
        n645 = call "数字密码键盘.vi"() -> ("NewNumber"=w953:sgl)  [unwired: 1 in]
        n646 = Equal?(x=w953, y=8.0) -> (x = y?=w954:bool)
        n647 = case shown="假" w954 {
          frame False {
            n648 = call "窗口弹出对话框(子VI).vi"("消息"="密码错误") -> ()  [unwired: 10 in, 1 out]
          }
          frame True {
          }
        }
      }
      event "锁定按钮": Mouse Down {
        n649 = event-data() -> ("CtlRef"=w959:refnum<vi>)  [unwired: 1 in, 7 out]
        n650 = property class="Bool (严格)"(reference=w959) -> ("Value"=w958:bool)  [unwired: 1 in, 2 out]
        n651 = case shown="真" w958 {
          selector: w958 -> [w960 _]
          tunnel: [w960 w961] -> w957
          frame False {
          }
          frame True {
            n652 = call "数字密码键盘.vi"() -> ("NewNumber"=w962:sgl)  [unwired: 1 in]
            n653 = Equal?(x=w962, y=8.0) -> (x = y?=w961:bool)
            n654 = case shown="假" w961 {
              selector: w961 -> [w965 _]
              frame False {
                n655 = One Button Dialog(message="密码错误!" ("消息")) -> ()  [unwired: 1 in, 1 out]
                n656 = local write "锁定按钮"(w965) -> ()
              }
              frame True {
                n657 = One Button Dialog(message="解锁成功!" ("消息")) -> ()  [unwired: 1 in, 1 out]
              }
            }
          }
        }
        "x = y?" <- w957
      }
      event "参数配置": Value Change {
        (unwired) u16 20 ("number of holding registers")
        (unwired) u16 4272 ("starting address")
        n658 = event-data() -> ()  [unwired: 1 in, 6 out]
        n659 = property on="窗格" class="Pane"("Origin"=T17 {"Horizontal"=0, "Vertical"=650} ("原点")) -> ()  [unwired: 2 in, 2 out]
        n660 = Bundle By Name(cluster=cluster{"命令":string} {"命令"=""} ("元素"), "命令"="CODMn读取参数" ("名称（未命名）")) -> (w971:cluster{"命令":string})
        n661 = Enqueue Element(queue=w970, element=w971, error in (no error)=w969) -> ()  [unwired: 1 in, 3 out]
        n662 = global read "COD读取DATA全局.vi" "配置文件ini"() -> (w967:string)
        n663 = call <vilib>:"Application Directory.vi"() -> ("Application Directory"=w974:path)
        n664 = Build Path(base path=w974, name or relative path=w967) -> (appended path=w975:path)
        n665 = call <vilib>:"Open Config Data.vi"("configuration file path"=w975) -> ("error out"=w979:errorcluster, "refnum"=w976:T7)  [unwired: 8 in, 1 out]
        n666 = vi-ref "斯坦道CODMn.lvlib:CODMn断电保存全局变量.vi"() -> (w977:refnum<vi>)
        n667 = call <userlib>:"Read Panel from INI__ogtk.vi"("error in (no error)"=w979, "VI ref"=w977, "refnum"=w976) -> ("error out"=w980:errorcluster, "refnum out"=w978:T7)  [unwired: 7 in]
        n668 = call <vilib>:"Close Config Data.vi"("error in (no error)"=w980, "refnum"=w978) -> ("error out"=w981:errorcluster, "file path"=w982:path)  [unwired: 8 in]
        n669 = Open/Create/Replace File(file path (use dialog)=w982, error in=w981) -> (error out=w968:errorcluster)  [unwired: 4 in, 2 out]
        n670 = call <vilib>:"Clear Errors.vi"("error in (no error)"=w968) -> ()  [unwired: 5 in, 2 out]
      }
      event "保存": Mouse Down {
        n671 = event-data() -> ()  [unwired: 1 in, 8 out]
        n672 = local read "通讯状态"() -> (w984:bool)
        n673 = Two Button Dialog(message="确定保存参数，保存参数将会替换原有参数！" ("消息")) -> (T button?=w986:bool)  [unwired: 2 in]
        n674 = case shown="假" w986 {
          tunnel: w984 -> [_ w987]
          frame False {
          }
          frame True {
            n675 = case shown="假" w987 {
              frame False {
                n676 = One Button Dialog(message="保存失败，当前无通讯！" ("消息")) -> ()  [unwired: 1 in, 1 out]
              }
              frame True {
                n677 = One Button Dialog(message="参数保存成功！" ("消息")) -> ()  [unwired: 1 in, 1 out]
                n678 = call "CODMnMB_api.vi"("STEP"=enum16{"open", "read", "write", "close"}."write", "values"="保存参数", "starting address"=u16 4272) -> ("error out"=w996:errorcluster)  [unwired: 6 in, 2 out]
                n679 = Build Array("采水泵进样时间/s:", "采水泵润洗时间/s:", "采水泵沉淀时间/s:", "采水泵排液时间/s:") -> (w990:i32[])
                n680 = call "CODMnMB_api.vi"("STEP"=enum16{"open", "read", "write", "close"}."write", "Error in"=w996, "values"=w990, "starting address"=u16 5596) -> ()  [unwired: 5 in, 3 out]
              }
            }
          }
        }
      }
      event "常规版/认证版": Value Change {
        n681 = event-data() -> ()  [unwired: 1 in, 6 out]
        n682 = flat-sequence {
          frame #0 {
            n683 = global write "CODMn断电保存全局变量.vi" "常规版/认证版"("常规版/认证版") -> ()
          }
          frame #1 {
            n684 = global read "COD读取DATA全局.vi" "配置文件ini"() -> (w1002:string)
            n685 = call <vilib>:"Application Directory.vi"() -> ("Application Directory"=w1015:path)
            n686 = Build Path(base path=w1015, name or relative path=w1002) -> (appended path=w1014:path)
            n687 = call <vilib>:"Open Config Data.vi"("configuration file path"=w1014) -> ("error out"=w1010:errorcluster, "refnum"=w1013:T7)  [unwired: 8 in, 1 out]
            n688 = vi-ref "斯坦道CODMn.lvlib:CODMn断电保存全局变量.vi"() -> (w1012:refnum<vi>)
            n689 = call <userlib>:"Write Panel to INI__ogtk.vi"("error in (no error)"=w1010, "VI ref"=w1012, "refnum"=w1013) -> ("error out"=w1009:errorcluster, "refnum out"=w1011:T7)  [unwired: 7 in]
            n690 = call <vilib>:"Close Config Data.vi"("error in (no error)"=w1009, "refnum"=w1011) -> ("error out"=w1004:errorcluster, "file path"=w1003:path)  [unwired: 8 in]
            n691 = Open/Create/Replace File(file path (use dialog)=w1003, error in=w1004) -> (refnum out=w1007:refnum<file>, error out=w1008:errorcluster)  [unwired: 4 in, 1 out]
            n692 = Flush File(refnum=w1007, error in=w1008) -> (refnum out=w1006:refnum<file>, error out=w1005:errorcluster)
            n693 = Close File(refnum=w1006, error in=w1005) -> ()  [unwired: 2 out]
          }
        }
      }
      event "校准配置": Value Change {
        n694 = event-data() -> ()  [unwired: 1 in, 6 out]
        n695 = property on="窗格" class="Pane"("Origin"=T17 {"Horizontal"=0, "Vertical"=1300} ("原点")) -> ()  [unwired: 2 in, 2 out]
        n696 = global read "COD读取DATA全局.vi" "配置文件ini"() -> (w1016:string)
        n697 = call <vilib>:"Application Directory.vi"() -> ("Application Directory"=w1066:path)
        n698 = Build Path(base path=w1066, name or relative path=w1016) -> (appended path=w1065:path)
        n699 = call <vilib>:"Open Config Data.vi"("configuration file path"=w1065) -> ("error out"=w1035:errorcluster, "refnum"=w1036:T7)  [unwired: 8 in, 1 out]
        n700 = local read "量程选择"() -> (w1042:enum16{"低量程", "高量程", "0-2量程"})
        n701 = call-poly <vilib>:"Read Key.vi"("section"="CODMn模型选择" ("key"), "error in (no error)"=w1035, "key"="线性和多项式", "refnum"=w1036) -> ("error out"=w1032:errorcluster, "value"=w1034:i32, "refnum out"=w1033:T7)  [unwired: 4 in, 1 out]
        n702 = case shown="\"0-2量程\"" w1042 {
          tunnel: ["低量程" "高量程" "0-2量程"] -> w1040
          frame "低量程", Default {
          }
          frame "高量程" {
          }
          frame "0-2量程" {
          }
        }
        n703 = local write "模型"(w1034) -> ()
        n704 = call-poly <vilib>:"Read Key.vi"("section"="标线选择", "error in (no error)"=w1032, "key"="选用水样", "refnum"=w1033) -> ("error out"=w1030:errorcluster, "value"=w1017:i32, "refnum out"=w1031:T7)  [unwired: 4 in, 1 out]
        n705 = case shown="0, 默认" w1017 {
          tunnel: ["葡萄糖标线" ("section") "草酸钠标线" ("section")] -> w1041
          frame 0, Default {
          }
          frame 1 {
          }
        }
        n706 = local write "选用水样"(w1017) -> ()
        n707 = Concatenate Strings(w1041, w1040) -> (w1039:string)
        n708 = call-poly <vilib>:"Read Key.vi"("section"=w1039, "error in (no error)"=w1030, "key"="浓度1", "refnum"=w1031) -> ("error out"=w1070:errorcluster, "value"=w1068:dbl, "refnum out"=w1069:T7)  [unwired: 4 in, 1 out]
        n709 = local write "浓度1"(w1068) -> ()
        n710 = call-poly <vilib>:"Read Key.vi"("section"=w1039, "error in (no error)"=w1070, "key"="浓度2", "refnum"=w1069) -> ("error out"=w1084:errorcluster, "value"=w1071:dbl, "refnum out"=w1083:T7)  [unwired: 4 in, 1 out]
        n711 = local write "浓度2"(w1071) -> ()
        n712 = call-poly <vilib>:"Read Key.vi"("section"=w1039, "error in (no error)"=w1084, "key"="浓度3", "refnum"=w1083) -> ("error out"=w1085:errorcluster, "value"=w1073:dbl, "refnum out"=w1082:T7)  [unwired: 4 in, 1 out]
        n713 = local write "浓度3"(w1073) -> ()
        n714 = call-poly <vilib>:"Read Key.vi"("section"=w1039, "error in (no error)"=w1085, "key"="泵滴定数1", "refnum"=w1082) -> ("error out"=w1086:errorcluster, "value"=w1075:dbl, "refnum out"=w1081:T7)  [unwired: 4 in, 1 out]
        n715 = local write "泵滴定数1"(w1075) -> ()
        n716 = call-poly <vilib>:"Read Key.vi"("section"=w1039, "error in (no error)"=w1086, "key"="泵滴定数2", "refnum"=w1081) -> ("error out"=w1080:errorcluster, "value"=w1078:dbl, "refnum out"=w1087:T7)  [unwired: 4 in, 1 out]
        n717 = local write "泵滴定数2"(w1078) -> ()
        n718 = call-poly <vilib>:"Read Key.vi"("section"=w1039, "error in (no error)"=w1080, "key"="泵滴定数3", "refnum"=w1087) -> ("error out"=w1092:errorcluster, "value"=w1091:dbl, "refnum out"=w1088:T7)  [unwired: 4 in, 1 out]
        n719 = local write "泵滴定数3"(w1091) -> ()
        n720 = call-poly <vilib>:"Read Key.vi"("section"=w1039, "error in (no error)"=w1092, "key"="浓度4", "refnum"=w1088) -> ("error out"=w1093:errorcluster, "value"=w1023:dbl, "refnum out"=w1089:T7)  [unwired: 4 in, 1 out]
        n721 = local write "浓度4"(w1023) -> ()
        n722 = call-poly <vilib>:"Read Key.vi"("section"=w1039, "error in (no error)"=w1093, "key"="浓度5", "refnum"=w1089) -> ("error out"=w1028:errorcluster, "value"=w1022:dbl, "refnum out"=w1029:T7)  [unwired: 4 in, 1 out]
        n723 = local write "浓度5"(w1022) -> ()
        n724 = call-poly <vilib>:"Read Key.vi"("section"=w1039, "error in (no error)"=w1028, "key"="泵滴定数4", "refnum"=w1029) -> ("error out"=w1094:errorcluster, "value"=w1021:dbl, "refnum out"=w1090:T7)  [unwired: 4 in, 1 out]
        n725 = local write "泵滴定数4"(w1021) -> ()
        n726 = call-poly <vilib>:"Read Key.vi"("section"=w1039, "error in (no error)"=w1094, "key"="泵滴定数5", "refnum"=w1090) -> ("error out"=w1026:errorcluster, "value"=w1020:dbl, "refnum out"=w1027:T7)  [unwired: 4 in, 1 out]
        n727 = local write "泵滴定数5"(w1020) -> ()
        n728 = call-poly <vilib>:"Read Key.vi"("section"=w1039, "error in (no error)"=w1026, "key"="当前选用的校准", "refnum"=w1027) -> ("error out"=w1061:errorcluster, "value"=w1063:i32, "refnum out"=w1062:T7)  [unwired: 4 in, 1 out]
        n729 = local write "当前校准"(w1063) -> ()
        n730 = call-poly <vilib>:"Read Key.vi"("section"=w1039, "error in (no error)"=w1061, "key"="启用1", "refnum"=w1062) -> ("error out"=w1058:errorcluster, "value"=w1047:bool, "refnum out"=w1059:T7)  [unwired: 4 in, 1 out]
        n731 = local write "启用1"(w1047) -> ()
        n732 = call-poly <vilib>:"Read Key.vi"("section"=w1039, "error in (no error)"=w1058, "key"="启用2", "refnum"=w1059) -> ("error out"=w1056:errorcluster, "value"=w1046:bool, "refnum out"=w1057:T7)  [unwired: 4 in, 1 out]
        n733 = local write "启用2"(w1046) -> ()
        n734 = call-poly <vilib>:"Read Key.vi"("section"=w1039, "error in (no error)"=w1056, "key"="启用3", "refnum"=w1057) -> ("error out"=w1054:errorcluster, "value"=w1045:bool, "refnum out"=w1055:T7)  [unwired: 4 in, 1 out]
        n735 = local write "启用3"(w1045) -> ()
        n736 = call-poly <vilib>:"Read Key.vi"("section"=w1039, "error in (no error)"=w1054, "key"="启用4", "refnum"=w1055) -> ("error out"=w1052:errorcluster, "value"=w1019:bool, "refnum out"=w1053:T7)  [unwired: 4 in, 1 out]
        n737 = local write "启用4"(w1019) -> ()
        n738 = call-poly <vilib>:"Read Key.vi"("section"=w1039, "error in (no error)"=w1052, "key"="启用5", "refnum"=w1053) -> ("error out"=w1024:errorcluster, "value"=w1018:bool, "refnum out"=w1025:T7)  [unwired: 4 in, 1 out]
        n739 = local write "启用5"(w1018) -> ()
        n740 = call <vilib>:"Close Config Data.vi"("error in (no error)"=w1024, "refnum"=w1025) -> ()  [unwired: 8 in, 2 out]
      }
      event "选用水样": Value Change {
        (unwired) "浓度6" ("key")
        n741 = event-data() -> ()  [unwired: 1 in, 6 out]
        n742 = property on="窗格" class="Pane"("Origin"=T17 {"Horizontal"=0, "Vertical"=1300} ("原点")) -> ()  [unwired: 2 in, 2 out]
        n743 = local read "量程选择"() -> (w1119:enum16{"低量程", "高量程", "0-2量程"})
        n744 = global read "COD读取DATA全局.vi" "配置文件ini"() -> (w1105:string)
        n745 = case shown="\"0-2量程\"" w1119 {
          tunnel: ["低量程" "高量程" "0-2量程"] -> w1120
          frame "低量程", Default {
          }
          frame "高量程" {
          }
          frame "0-2量程" {
          }
        }
        n746 = case shown="\"葡萄糖\", 默认" "选用水样" {
          tunnel: ["葡萄糖标线" ("section") "草酸钠标线" ("section")] -> w1121
          frame "葡萄糖", Default {
          }
          frame "草酸钠" {
          }
        }
        n747 = call <vilib>:"Application Directory.vi"() -> ("Application Directory"=w1144:path)
        n748 = Build Path(base path=w1144, name or relative path=w1105) -> (appended path=w1143:path)
        n749 = call <vilib>:"Open Config Data.vi"("configuration file path"=w1143) -> ("error out"=w1145:errorcluster, "refnum"=w1146:T7)  [unwired: 8 in, 1 out]
        n750 = Concatenate Strings(w1121, w1120) -> (w1118:string)
        n751 = call-poly <vilib>:"Read Key.vi"("section"=w1118, "error in (no error)"=w1145, "key"="浓度1", "refnum"=w1146) -> ("error out"=w1150:errorcluster, "value"=w1148:dbl, "refnum out"=w1149:T7)  [unwired: 4 in, 1 out]
        n752 = local write "浓度1"(w1148) -> ()
        n753 = call-poly <vilib>:"Read Key.vi"("section"=w1118, "error in (no error)"=w1150, "key"="浓度2", "refnum"=w1149) -> ("error out"=w1164:errorcluster, "value"=w1151:dbl, "refnum out"=w1163:T7)  [unwired: 4 in, 1 out]
        n754 = local write "浓度2"(w1151) -> ()
        n755 = call-poly <vilib>:"Read Key.vi"("section"=w1118, "error in (no error)"=w1164, "key"="浓度3", "refnum"=w1163) -> ("error out"=w1165:errorcluster, "value"=w1153:dbl, "refnum out"=w1162:T7)  [unwired: 4 in, 1 out]
        n756 = local write "浓度3"(w1153) -> ()
        n757 = call-poly <vilib>:"Read Key.vi"("section"=w1118, "error in (no error)"=w1165, "key"="泵滴定数1", "refnum"=w1162) -> ("error out"=w1166:errorcluster, "value"=w1155:dbl, "refnum out"=w1161:T7)  [unwired: 4 in, 1 out]
        n758 = local write "泵滴定数1"(w1155) -> ()
        n759 = call-poly <vilib>:"Read Key.vi"("section"=w1118, "error in (no error)"=w1166, "key"="泵滴定数2", "refnum"=w1161) -> ("error out"=w1160:errorcluster, "value"=w1158:dbl, "refnum out"=w1167:T7)  [unwired: 4 in, 1 out]
        n760 = local write "泵滴定数2"(w1158) -> ()
        n761 = call-poly <vilib>:"Read Key.vi"("section"=w1118, "error in (no error)"=w1160, "key"="泵滴定数3", "refnum"=w1167) -> ("error out"=w1172:errorcluster, "value"=w1171:dbl, "refnum out"=w1168:T7)  [unwired: 4 in, 1 out]
        n762 = local write "泵滴定数3"(w1171) -> ()
        n763 = call-poly <vilib>:"Read Key.vi"("section"=w1118, "error in (no error)"=w1172, "key"="浓度4", "refnum"=w1168) -> ("error out"=w1173:errorcluster, "value"=w1113:dbl, "refnum out"=w1169:T7)  [unwired: 4 in, 1 out]
        n764 = local write "浓度4"(w1113) -> ()
        n765 = call-poly <vilib>:"Read Key.vi"("section"=w1118, "error in (no error)"=w1173, "key"="浓度5", "refnum"=w1169) -> ("error out"=w1116:errorcluster, "value"=w1112:dbl, "refnum out"=w1117:T7)  [unwired: 4 in, 1 out]
        n766 = local write "浓度5"(w1112) -> ()
        n767 = call-poly <vilib>:"Read Key.vi"("section"=w1118, "error in (no error)"=w1116, "key"="泵滴定数4", "refnum"=w1117) -> ("error out"=w1174:errorcluster, "value"=w1111:dbl, "refnum out"=w1170:T7)  [unwired: 4 in, 1 out]
        n768 = local write "泵滴定数4"(w1111) -> ()
        n769 = call-poly <vilib>:"Read Key.vi"("section"=w1118, "error in (no error)"=w1174, "key"="泵滴定数5", "refnum"=w1170) -> ("error out"=w1114:errorcluster, "value"=w1110:dbl, "refnum out"=w1115:T7)  [unwired: 4 in, 1 out]
        n770 = local write "泵滴定数5"(w1110) -> ()
        n771 = call-poly <vilib>:"Read Key.vi"("section"=w1118, "error in (no error)"=w1114, "key"="当前选用的校准", "refnum"=w1115) -> ("error out"=w1139:errorcluster, "value"=w1141:i32, "refnum out"=w1140:T7)  [unwired: 4 in, 1 out]
        n772 = call-poly <vilib>:"Read Key.vi"("section"=w1118, "error in (no error)"=w1139, "key"="启用1", "refnum"=w1140) -> ("error out"=w1136:errorcluster, "value"=w1125:bool, "refnum out"=w1137:T7)  [unwired: 4 in, 1 out]
        n773 = local write "当前校准"(w1141) -> ()
        n774 = local write "启用1"(w1125) -> ()
        n775 = call-poly <vilib>:"Read Key.vi"("section"=w1118, "error in (no error)"=w1136, "key"="启用2", "refnum"=w1137) -> ("error out"=w1134:errorcluster, "value"=w1124:bool, "refnum out"=w1135:T7)  [unwired: 4 in, 1 out]
        n776 = local write "启用2"(w1124) -> ()
        n777 = call-poly <vilib>:"Read Key.vi"("section"=w1118, "error in (no error)"=w1134, "key"="启用3", "refnum"=w1135) -> ("error out"=w1132:errorcluster, "value"=w1123:bool, "refnum out"=w1133:T7)  [unwired: 4 in, 1 out]
        n778 = local write "启用3"(w1123) -> ()
        n779 = call-poly <vilib>:"Read Key.vi"("section"=w1118, "error in (no error)"=w1132, "key"="启用4", "refnum"=w1133) -> ("error out"=w1130:errorcluster, "value"=w1107:bool, "refnum out"=w1131:T7)  [unwired: 4 in, 1 out]
        n780 = local write "启用4"(w1107) -> ()
        n781 = call-poly <vilib>:"Read Key.vi"("section"=w1118, "error in (no error)"=w1130, "key"="启用5", "refnum"=w1131) -> ("error out"=w1108:errorcluster, "value"=w1106:bool, "refnum out"=w1109:T7)  [unwired: 4 in, 1 out]
        n782 = local write "启用5"(w1106) -> ()
        n783 = call <vilib>:"Close Config Data.vi"("error in (no error)"=w1108, "refnum"=w1109) -> ()  [unwired: 8 in, 2 out]
      }
      event "量程选择": Value Change {
        n784 = event-data() -> ()  [unwired: 1 in, 6 out]
        n785 = local read "选用水样"() -> (w1202:enum16{"葡萄糖", "草酸钠"})
        n786 = global read "COD读取DATA全局.vi" "配置文件ini"() -> (w1185:string)
        n787 = property on="窗格" class="Pane"("Origin"=T17 {"Horizontal"=0, "Vertical"=1300} ("原点")) -> ()  [unwired: 2 in, 2 out]
        n788 = case shown="\"葡萄糖\", 默认" w1202 {
          tunnel: ["葡萄糖标线" ("section") "草酸钠标线" ("section")] -> w1201
          frame "葡萄糖", Default {
          }
          frame "草酸钠" {
          }
        }
        n789 = case shown="\"0-2量程\"" "量程选择" {
          tunnel: ["低量程" "高量程" "0-2量程"] -> w1198
          frame "低量程", Default {
          }
          frame "高量程" {
          }
          frame "0-2量程" {
          }
        }
        n790 = call <vilib>:"Application Directory.vi"() -> ("Application Directory"=w1224:path)
        n791 = Build Path(base path=w1224, name or relative path=w1185) -> (appended path=w1223:path)
        n792 = call <vilib>:"Open Config Data.vi"("configuration file path"=w1223) -> ("error out"=w1225:errorcluster, "refnum"=w1226:T7)  [unwired: 8 in, 1 out]
        n793 = Concatenate Strings(w1201, w1198) -> (w1200:string)
        n794 = call-poly <vilib>:"Read Key.vi"("section"=w1200, "error in (no error)"=w1225, "key"="浓度1", "refnum"=w1226) -> ("error out"=w1230:errorcluster, "value"=w1228:dbl, "refnum out"=w1229:T7)  [unwired: 4 in, 1 out]
        n795 = local write "浓度1"(w1228) -> ()
        n796 = call-poly <vilib>:"Read Key.vi"("section"=w1200, "error in (no error)"=w1230, "key"="浓度2", "refnum"=w1229) -> ("error out"=w1244:errorcluster, "value"=w1231:dbl, "refnum out"=w1243:T7)  [unwired: 4 in, 1 out]
        n797 = local write "浓度2"(w1231) -> ()
        n798 = call-poly <vilib>:"Read Key.vi"("section"=w1200, "error in (no error)"=w1244, "key"="浓度3", "refnum"=w1243) -> ("error out"=w1245:errorcluster, "value"=w1233:dbl, "refnum out"=w1242:T7)  [unwired: 4 in, 1 out]
        n799 = local write "浓度3"(w1233) -> ()
        n800 = call-poly <vilib>:"Read Key.vi"("section"=w1200, "error in (no error)"=w1245, "key"="泵滴定数1", "refnum"=w1242) -> ("error out"=w1246:errorcluster, "value"=w1235:dbl, "refnum out"=w1241:T7)  [unwired: 4 in, 1 out]
        n801 = local write "泵滴定数1"(w1235) -> ()
        n802 = call-poly <vilib>:"Read Key.vi"("section"=w1200, "error in (no error)"=w1246, "key"="泵滴定数2", "refnum"=w1241) -> ("error out"=w1240:errorcluster, "value"=w1238:dbl, "refnum out"=w1247:T7)  [unwired: 4 in, 1 out]
        n803 = local write "泵滴定数2"(w1238) -> ()
        n804 = call-poly <vilib>:"Read Key.vi"("section"=w1200, "error in (no error)"=w1240, "key"="泵滴定数3", "refnum"=w1247) -> ("error out"=w1252:errorcluster, "value"=w1251:dbl, "refnum out"=w1248:T7)  [unwired: 4 in, 1 out]
        n805 = local write "泵滴定数3"(w1251) -> ()
        n806 = call-poly <vilib>:"Read Key.vi"("section"=w1200, "error in (no error)"=w1252, "key"="浓度4", "refnum"=w1248) -> ("error out"=w1253:errorcluster, "value"=w1189:dbl, "refnum out"=w1249:T7)  [unwired: 4 in, 1 out]
        n807 = local write "浓度4"(w1189) -> ()
        n808 = call-poly <vilib>:"Read Key.vi"("section"=w1200, "error in (no error)"=w1253, "key"="浓度5", "refnum"=w1249) -> ("error out"=w1196:errorcluster, "value"=w1188:dbl, "refnum out"=w1197:T7)  [unwired: 4 in, 1 out]
        n809 = local write "浓度5"(w1188) -> ()
        n810 = call-poly <vilib>:"Read Key.vi"("section"=w1200, "error in (no error)"=w1196, "key"="泵滴定数4", "refnum"=w1197) -> ("error out"=w1254:errorcluster, "value"=w1187:dbl, "refnum out"=w1250:T7)  [unwired: 4 in, 1 out]
        n811 = local write "泵滴定数4"(w1187) -> ()
        n812 = call-poly <vilib>:"Read Key.vi"("section"=w1200, "error in (no error)"=w1254, "key"="泵滴定数5", "refnum"=w1250) -> ("error out"=w1194:errorcluster, "value"=w1186:dbl, "refnum out"=w1195:T7)  [unwired: 4 in, 1 out]
        n813 = local write "泵滴定数5"(w1186) -> ()
        n814 = call-poly <vilib>:"Read Key.vi"("section"=w1200, "error in (no error)"=w1194, "key"="当前选用的校准", "refnum"=w1195) -> ("error out"=w1219:errorcluster, "value"=w1221:i32, "refnum out"=w1220:T7)  [unwired: 4 in, 1 out]
        n815 = local write "当前校准"(w1221) -> ()
        n816 = call-poly <vilib>:"Read Key.vi"("section"=w1200, "error in (no error)"=w1219, "key"="启用1", "refnum"=w1220) -> ("error out"=w1216:errorcluster, "value"=w1205:bool, "refnum out"=w1217:T7)  [unwired: 4 in, 1 out]
        n817 = local write "启用1"(w1205) -> ()
        n818 = call-poly <vilib>:"Read Key.vi"("section"=w1200, "error in (no error)"=w1216, "key"="启用2", "refnum"=w1217) -> ("error out"=w1214:errorcluster, "value"=w1204:bool, "refnum out"=w1215:T7)  [unwired: 4 in, 1 out]
        n819 = local write "启用2"(w1204) -> ()
        n820 = call-poly <vilib>:"Read Key.vi"("section"=w1200, "error in (no error)"=w1214, "key"="启用3", "refnum"=w1215) -> ("error out"=w1212:errorcluster, "value"=w1203:bool, "refnum out"=w1213:T7)  [unwired: 4 in, 1 out]
        n821 = local write "启用3"(w1203) -> ()
        n822 = call-poly <vilib>:"Read Key.vi"("section"=w1200, "error in (no error)"=w1212, "key"="启用4", "refnum"=w1213) -> ("error out"=w1210:errorcluster, "value"=w1191:bool, "refnum out"=w1211:T7)  [unwired: 4 in, 1 out]
        n823 = local write "启用4"(w1191) -> ()
        n824 = call-poly <vilib>:"Read Key.vi"("section"=w1200, "error in (no error)"=w1210, "key"="启用5", "refnum"=w1211) -> ("error out"=w1192:errorcluster, "value"=w1190:bool, "refnum out"=w1193:T7)  [unwired: 4 in, 1 out]
        n825 = local write "启用5"(w1190) -> ()
        n826 = call <vilib>:"Close Config Data.vi"("error in (no error)"=w1192, "refnum"=w1193) -> ()  [unwired: 8 in, 2 out]
      }
      event "返回": Value Change {
        w1279 = "CODMn" ("section")
        n827 = event-data() -> ()  [unwired: 1 in, 6 out]
        n828 = global read "COD读取DATA全局.vi" "配置文件ini"() -> (w1265:string)
        n829 = property on="窗格" class="Pane"("Origin"=T17 {"Horizontal"=0, "Vertical"=0} ("原点")) -> ()  [unwired: 2 in, 2 out]
        n830 = call <vilib>:"Application Directory.vi"() -> ("Application Directory"=w1331:path)
        n831 = Build Path(base path=w1331, name or relative path=w1265) -> (appended path=w1330:path)
        n832 = local read "浓度1"() -> (w1326:dbl)
        n833 = call <vilib>:"Open Config Data.vi"("configuration file path"=w1330) -> ("error out"=w1328:errorcluster, "refnum"=w1329:T7)  [unwired: 8 in, 1 out]
        n834 = local read "浓度2"() -> (w1310:dbl)
        n835 = call-poly <vilib>:"Write Key.vi"("section"=w1279, "error in (no error)"=w1328, "value"=w1326, "key"="浓度1", "refnum"=w1329) -> ("error out"=w1325:errorcluster, "refnum out"=w1324:T7)  [unwired: 4 in, 1 out]
        n836 = local read "浓度3"() -> (w1306:dbl)
        n837 = call-poly <vilib>:"Write Key.vi"("section"=w1279, "error in (no error)"=w1325, "value"=w1310, "key"="浓度2", "refnum"=w1324) -> ("error out"=w1323:errorcluster, "refnum out"=w1322:T7)  [unwired: 4 in, 1 out]
        n838 = local read "泵滴定数1"() -> (w1304:dbl)
        n839 = call-poly <vilib>:"Write Key.vi"("section"=w1279, "error in (no error)"=w1323, "value"=w1306, "key"="浓度3", "refnum"=w1322) -> ("error out"=w1321:errorcluster, "refnum out"=w1320:T7)  [unwired: 4 in, 1 out]
        n840 = call-poly <vilib>:"Write Key.vi"("section"=w1279, "error in (no error)"=w1321, "value"=w1304, "key"="泵滴定数1", "refnum"=w1320) -> ("error out"=w1319:errorcluster, "refnum out"=w1318:T7)  [unwired: 4 in, 1 out]
        n841 = local read "泵滴定数2"() -> (w1302:dbl)
        n842 = call-poly <vilib>:"Write Key.vi"("section"=w1279, "error in (no error)"=w1319, "value"=w1302, "key"="泵滴定数2", "refnum"=w1318) -> ("error out"=w1317:errorcluster, "refnum out"=w1316:T7)  [unwired: 4 in, 1 out]
        n843 = local read "泵滴定数3"() -> (w1300:dbl)
        n844 = local read "浓度4"() -> (w1267:dbl)
        n845 = call-poly <vilib>:"Write Key.vi"("section"=w1279, "error in (no error)"=w1317, "value"=w1300, "key"="泵滴定数3", "refnum"=w1316) -> ("error out"=w1315:errorcluster, "refnum out"=w1314:T7)  [unwired: 4 in, 1 out]
        n846 = call-poly <vilib>:"Write Key.vi"("section"=w1279, "error in (no error)"=w1315, "value"=w1267, "key"="浓度4", "refnum"=w1314) -> ("error out"=w1308:errorcluster, "refnum out"=w1309:T7)  [unwired: 4 in, 1 out]
        n847 = local read "浓度5"() -> (w1266:dbl)
        n848 = call-poly <vilib>:"Write Key.vi"("section"=w1279, "error in (no error)"=w1308, "value"=w1266, "key"="浓度5", "refnum"=w1309) -> ("error out"=w1276:errorcluster, "refnum out"=w1277:T7)  [unwired: 4 in, 1 out]
        n849 = local read "泵滴定数4"() -> (w1268:dbl)
        n850 = call-poly <vilib>:"Write Key.vi"("section"=w1279, "error in (no error)"=w1276, "value"=w1268, "key"="泵滴定数4", "refnum"=w1277) -> ("error out"=w1313:errorcluster, "refnum out"=w1312:T7)  [unwired: 4 in, 1 out]
        n851 = local read "泵滴定数5"() -> (w1269:dbl)
        n852 = call-poly <vilib>:"Write Key.vi"("section"=w1279, "error in (no error)"=w1313, "value"=w1269, "key"="泵滴定数5", "refnum"=w1312) -> ("error out"=w1274:errorcluster, "refnum out"=w1275:T7)  [unwired: 4 in, 1 out]
        n853 = local read "启用1"() -> (w1288:bool)
        n854 = call-poly <vilib>:"Write Key.vi"("section"=w1279, "error in (no error)"=w1274, "value"=w1288, "key"="启用1", "refnum"=w1275) -> ("error out"=w1284:errorcluster, "refnum out"=w1287:T7)  [unwired: 4 in, 1 out]
        n855 = local read "启用2"() -> (w1285:bool)
        n856 = call-poly <vilib>:"Write Key.vi"("section"=w1279, "error in (no error)"=w1284, "value"=w1285, "key"="启用2", "refnum"=w1287) -> ("error out"=w1295:errorcluster, "refnum out"=w1294:T7)  [unwired: 4 in, 1 out]
        n857 = local read "启用3"() -> (w1283:bool)
        n858 = call-poly <vilib>:"Write Key.vi"("section"=w1279, "error in (no error)"=w1295, "value"=w1283, "key"="启用3", "refnum"=w1294) -> ("error out"=w1293:errorcluster, "refnum out"=w1292:T7)  [unwired: 4 in, 1 out]
        n859 = local read "启用4"() -> (w1271:bool)
        n860 = call-poly <vilib>:"Write Key.vi"("section"=w1279, "error in (no error)"=w1293, "value"=w1271, "key"="启用4", "refnum"=w1292) -> ("error out"=w1291:errorcluster, "refnum out"=w1290:T7)  [unwired: 4 in, 1 out]
        n861 = local read "启用5"() -> (w1270:bool)
        n862 = call-poly <vilib>:"Write Key.vi"("section"=w1279, "error in (no error)"=w1291, "value"=w1270, "key"="启用5", "refnum"=w1290) -> ("error out"=w1272:errorcluster, "refnum out"=w1273:T7)  [unwired: 4 in, 1 out]
        n863 = call <vilib>:"Close Config Data.vi"("error in (no error)"=w1272, "refnum"=w1273) -> ()  [unwired: 8 in, 2 out]
      }
      event "关闭", "关闭 2", "关闭 3": Value Change {
        n864 = event-data() -> ()  [unwired: 1 in, 6 out]
        n865 = property on="窗格" class="Pane"("Origin"=T17 {"Horizontal"=0, "Vertical"=0} ("原点")) -> ()  [unwired: 2 in, 2 out]
      }
      event Application Instance Close {
        n866 = event-data() -> ()  [unwired: 1 in, 4 out]
      }
      event "时间校准": Value Change {
        n867 = event-data() -> ()  [unwired: 1 in, 6 out]
        n868 = Get Date/Time In Seconds() -> (seconds since 1Jan1904=w1341:timestamp)
        n869 = Build Array(w1341) -> (w1340:timestamp[])
        n870 = call "DateToHex.vi"("DATE"=w1340) -> ("数组"=w1338:u16[])  [unwired: 10 in]
        n871 = Insert Into Array(array=u16[] [1] ("values"), index=1 ("索引"), new element=w1338) -> (w1334:u16[])
        n872 = call "CODMnMB_api.vi"("STEP"=enum16{"open", "read", "write", "close"}."write", "values"=w1334, "starting address"=u16 4612) -> ("error out"=w1333:errorcluster)  [unwired: 6 in, 2 out]
        n873 = call <vilib>:"Clear Errors.vi"("error in (no error)"=w1333) -> ()  [unwired: 5 in, 2 out]
      }
      event "故障清除": Value Change {
        n874 = event-data() -> ()  [unwired: 1 in, 6 out]
        n875 = call "CODMnMB_api.vi"("STEP"=enum16{"open", "read", "write", "close"}."write", "values"=u16[] [1], "starting address"=u16 4611) -> ()  [unwired: 6 in, 3 out]
      }
      event "定时启动": Mouse Down {
        n876 = event-data() -> ()  [unwired: 1 in, 8 out]
        n877 = flat-sequence {
          frame #0 {
            n878 = global read "CODMn断电保存全局变量.vi" "定时控制"() -> (w1346:T11)
            n879 = call "周期设置.vi"("定时控制参数输入"=w1346) -> ("定时控制参数输出"=w1345:T11)  [unwired: 10 in]
            n880 = global write "CODMn断电保存全局变量.vi" "定时控制"(w1345) -> ()
          }
          frame #1 {
            n881 = global read "COD读取DATA全局.vi" "配置文件ini"() -> (w1347:string)
            n882 = call <vilib>:"Application Directory.vi"() -> ("Application Directory"=w1360:path)
            n883 = Build Path(base path=w1360, name or relative path=w1347) -> (appended path=w1359:path)
            n884 = call <vilib>:"Open Config Data.vi"("configuration file path"=w1359) -> ("error out"=w1355:errorcluster, "refnum"=w1358:T7)  [unwired: 8 in, 1 out]
            n885 = vi-ref "斯坦道CODMn.lvlib:CODMn断电保存全局变量.vi"() -> (w1357:refnum<vi>)
            n886 = call <userlib>:"Write Panel to INI__ogtk.vi"("error in (no error)"=w1355, "VI ref"=w1357, "refnum"=w1358) -> ("error out"=w1354:errorcluster, "refnum out"=w1356:T7)  [unwired: 7 in]
            n887 = call <vilib>:"Close Config Data.vi"("error in (no error)"=w1354, "refnum"=w1356) -> ("error out"=w1349:errorcluster, "file path"=w1348:path)  [unwired: 8 in]
            n888 = Open/Create/Replace File(file path (use dialog)=w1348, error in=w1349) -> (refnum out=w1352:refnum<file>, error out=w1353:errorcluster)  [unwired: 4 in, 1 out]
            n889 = Flush File(refnum=w1352, error in=w1353) -> (refnum out=w1351:refnum<file>, error out=w1350:errorcluster)
            n890 = Close File(refnum=w1351, error in=w1350) -> ()  [unwired: 2 out]
          }
        }
      }
      event "测量模式(公式)": Value Change {
        n891 = event-data() -> ()  [unwired: 1 in, 6 out]
        n892 = flat-sequence {
          frame #0 {
            n893 = global write "CODMn断电保存全局变量.vi" "测量模式(公式)"("测量模式(公式)") -> ()
          }
          frame #1 {
            n894 = global read "COD读取DATA全局.vi" "配置文件ini"() -> (w1362:string)
            n895 = call <vilib>:"Application Directory.vi"() -> ("Application Directory"=w1375:path)
            n896 = Build Path(base path=w1375, name or relative path=w1362) -> (appended path=w1374:path)
            n897 = call <vilib>:"Open Config Data.vi"("configuration file path"=w1374) -> ("error out"=w1370:errorcluster, "refnum"=w1373:T7)  [unwired: 8 in, 1 out]
            n898 = vi-ref "斯坦道CODMn.lvlib:CODMn断电保存全局变量.vi"() -> (w1372:refnum<vi>)
            n899 = call <userlib>:"Write Panel to INI__ogtk.vi"("error in (no error)"=w1370, "VI ref"=w1372, "refnum"=w1373) -> ("error out"=w1369:errorcluster, "refnum out"=w1371:T7)  [unwired: 7 in]
            n900 = call <vilib>:"Close Config Data.vi"("error in (no error)"=w1369, "refnum"=w1371) -> ("error out"=w1364:errorcluster, "file path"=w1363:path)  [unwired: 8 in]
            n901 = Open/Create/Replace File(file path (use dialog)=w1363, error in=w1364) -> (refnum out=w1367:refnum<file>, error out=w1368:errorcluster)  [unwired: 4 in, 1 out]
            n902 = Flush File(refnum=w1367, error in=w1368) -> (refnum out=w1366:refnum<file>, error out=w1365:errorcluster)
            n903 = Close File(refnum=w1366, error in=w1365) -> ()  [unwired: 2 out]
          }
        }
      }
      event "跨度量程选择", "跨度液浓度", "零点核查量程选择", "零点核查浓度", "标样浓度", "标样核查量程选择": Value Change {
        n904 = event-data() -> ()  [unwired: 1 in, 6 out]
        n905 = flat-sequence {
          frame #0 {
            n906 = global write "CODMn断电保存全局变量.vi" "标样浓度"("标样浓度") -> ()
            n907 = global write "CODMn断电保存全局变量.vi" "标样核查量程选择"("标样核查量程选择") -> ()
            n908 = global write "CODMn断电保存全局变量.vi" "零点核查浓度"("零点核查浓度") -> ()
            n909 = global write "CODMn断电保存全局变量.vi" "CODMn跨度量程选择"("跨度量程选择") -> ()
            n910 = global write "CODMn断电保存全局变量.vi" "跨度液浓度"("跨度液浓度") -> ()
            n911 = global write "CODMn断电保存全局变量.vi" "零点核查量程选择"("零点核查量程选择") -> ()
          }
          frame #1 {
            n912 = global read "COD读取DATA全局.vi" "配置文件ini"() -> (w1382:string)
            n913 = call <vilib>:"Application Directory.vi"() -> ("Application Directory"=w1395:path)
            n914 = Build Path(base path=w1395, name or relative path=w1382) -> (appended path=w1394:path)
            n915 = call <vilib>:"Open Config Data.vi"("configuration file path"=w1394) -> ("error out"=w1390:errorcluster, "refnum"=w1393:T7)  [unwired: 8 in, 1 out]
            n916 = vi-ref "斯坦道CODMn.lvlib:CODMn断电保存全局变量.vi"() -> (w1392:refnum<vi>)
            n917 = call <userlib>:"Write Panel to INI__ogtk.vi"("error in (no error)"=w1390, "VI ref"=w1392, "refnum"=w1393) -> ("error out"=w1389:errorcluster, "refnum out"=w1391:T7)  [unwired: 7 in]
            n918 = call <vilib>:"Close Config Data.vi"("error in (no error)"=w1389, "refnum"=w1391) -> ("error out"=w1384:errorcluster, "file path"=w1383:path)  [unwired: 8 in]
            n919 = Open/Create/Replace File(file path (use dialog)=w1383, error in=w1384) -> (refnum out=w1387:refnum<file>, error out=w1388:errorcluster)  [unwired: 4 in, 1 out]
            n920 = Flush File(refnum=w1387, error in=w1388) -> (refnum out=w1386:refnum<file>, error out=w1385:errorcluster)
            n921 = Close File(refnum=w1386, error in=w1385) -> ()  [unwired: 2 out]
          }
        }
      }
      event "校准1", "校准2", "校准3", "校准4", "校准5": Value Change {
        n922 = event-data() -> ()  [unwired: 1 in, 6 out]
        n923 = flat-sequence {
          frame #0 {
            n924 = Build Array("校准1", "校准2", "校准3", "校准4", "校准5") -> (w1398:bool[])
            n925 = for {
              tunnel: w1398 -> [w1409] mode=indexing
              i -> [w1402]
              n926 = case shown="4" w1402 {
                tunnel: ["浓度1" "浓度2" "浓度3" "浓度4" "浓度5"] -> w1405
                frame 0, Default {
                }
                frame 1 {
                }
                frame 2 {
                }
                frame 3 {
                }
                frame 4 {
                }
              }
              n927 = Multiply(x=w1405, y=100.0) -> (x*y=w1403:dbl)
              n928 = Insert Into Array(array=u16[] [] ("values"), index=0 ("索引"), new element=w1403) -> (w1406:u16[])
              n929 = case shown="真" w1409 {
                tunnel: w1406 -> [_ w1416]
                tunnel: w1402 -> [_ w1419]
                frame False {
                }
                frame True {
                  n930 = Increment(x=w1419) -> (x+1=→"当前校准":i32)
                  n931 = call "CODMnMB_api.vi"("STEP"=enum16{"open", "read", "write", "close"}."write", "values"=w1416, "starting address"=u16 4274) -> ()  [unwired: 6 in, 3 out]
                }
              }
            }
          }
          frame #1 {
            n932 = local read "当前校准"() -> (w1426:i32)
            n933 = case shown="5" w1426 {
              tunnel: [w1430 w1431 w1432 w1433 w1434] -> w1425
              frame 1, Default {
                n934 = local read "浓度1"() -> (w1430:dbl)
              }
              frame 2 {
                n935 = local read "浓度2"() -> (w1431:dbl)
              }
              frame 3 {
                n936 = local read "浓度3"() -> (w1432:dbl)
              }
              frame 4 {
                n937 = local read "浓度4"() -> (w1433:dbl)
              }
              frame 5 {
                n938 = local read "浓度5"() -> (w1434:dbl)
              }
            }
            n939 = Not Equal To 0?(x=w1425) -> (x != 0?=w1423:bool)
            n940 = case shown="真" w1423 {
              tunnel: [u16 8 ("address") u16 9 ("address")] -> w1429
              tunnel: ["校零" ("测量模式") "校标" ("测量模式")] -> w1424
              frame False {
              }
              frame True {
              }
            }
            n941 = global write "COD测量模式全局.vi" "测量模式"(w1424) -> ()
            n942 = Insert Into Array(array=u16[] [] ("values"), index=0 ("索引"), new element=w1429) -> (w1420:u16[])
            n943 = call "CODMnMB_api.vi"("STEP"=enum16{"open", "read", "write", "close"}."write", "values"=w1420, "starting address"=u16 4608 ("address")) -> ()  [unwired: 6 in, 3 out]
          }
          frame #2 {
            n944 = local read "选用水样"() -> (w1442:enum16{"葡萄糖", "草酸钠"})
            n945 = local read "量程选择"() -> (w1441:enum16{"低量程", "高量程", "0-2量程"})
            n946 = case shown="\"葡萄糖\", 默认" w1442 {
              tunnel: ["葡萄糖标线" ("section") "草酸钠标线" ("section")] -> w1443
              frame "葡萄糖", Default {
              }
              frame "草酸钠" {
              }
            }
            n947 = global read "COD读取DATA全局.vi" "配置文件ini"() -> (w1439:string)
            n948 = case shown="\"0-2量程\"" w1441 {
              tunnel: ["低量程" "高量程" "0-2量程"] -> w1444
              frame "低量程", Default {
              }
              frame "高量程" {
              }
              frame "0-2量程" {
              }
            }
            n949 = call <vilib>:"Application Directory.vi"() -> ("Application Directory"=w1451:path)
            n950 = Concatenate Strings(w1443, w1444) -> (w1440:string)
            n951 = Build Path(base path=w1451, name or relative path=w1439) -> (appended path=w1452:path)
            n952 = local read "当前校准"() -> (w1447:i32)
            n953 = call <vilib>:"Open Config Data.vi"("configuration file path"=w1452) -> ("error out"=w1449:errorcluster, "refnum"=w1450:T7)  [unwired: 8 in, 1 out]
            n954 = call-poly <vilib>:"Write Key.vi"("section"=w1440, "error in (no error)"=w1449, "value"=w1447, "key"="当前选用的校准" ("section"), "refnum"=w1450) -> ("error out"=w1445:errorcluster, "refnum out"=w1446:T7)  [unwired: 4 in, 1 out]
            n955 = call <vilib>:"Close Config Data.vi"("error in (no error)"=w1445, "refnum"=w1446) -> ()  [unwired: 8 in, 2 out]
          }
        }
      }
      event "自动切换量程:", "低切高阈值:", "高切低阈值:": Value Change {
        n956 = event-data() -> ()  [unwired: 1 in, 6 out]
        n957 = flat-sequence {
          frame #0 {
            n958 = local read "自动切换量程:"() -> (w1460:enum16{"关闭", "自动切换测一次", "自动切换测两次"})
            n959 = local read "低切高阈值:"() -> (w1459:dbl)
            n960 = local read "高切低阈值:"() -> (w1458:dbl)
            n961 = global write "CODMn断电保存全局变量.vi" "自动切换量程:"(w1460) -> ()
            n962 = global write "CODMn断电保存全局变量.vi" "低切高阈值:"(w1459) -> ()
            n963 = global write "CODMn断电保存全局变量.vi" "高切低阈值:"(w1458) -> ()
          }
          frame #1 {
            n964 = global read "COD读取DATA全局.vi" "配置文件ini"() -> (w1461:string)
            n965 = call <vilib>:"Application Directory.vi"() -> ("Application Directory"=w1474:path)
            n966 = Build Path(base path=w1474, name or relative path=w1461) -> (appended path=w1473:path)
            n967 = call <vilib>:"Open Config Data.vi"("configuration file path"=w1473) -> ("error out"=w1469:errorcluster, "refnum"=w1472:T7)  [unwired: 8 in, 1 out]
            n968 = vi-ref "斯坦道CODMn.lvlib:CODMn断电保存全局变量.vi"() -> (w1471:refnum<vi>)
            n969 = call <userlib>:"Write Panel to INI__ogtk.vi"("error in (no error)"=w1469, "VI ref"=w1471, "refnum"=w1472) -> ("error out"=w1468:errorcluster, "refnum out"=w1470:T7)  [unwired: 7 in]
            n970 = call <vilib>:"Close Config Data.vi"("error in (no error)"=w1468, "refnum"=w1470) -> ("error out"=w1463:errorcluster, "file path"=w1462:path)  [unwired: 8 in]
            n971 = Open/Create/Replace File(file path (use dialog)=w1462, error in=w1463) -> (refnum out=w1466:refnum<file>, error out=w1467:errorcluster)  [unwired: 4 in, 1 out]
            n972 = Flush File(refnum=w1466, error in=w1467) -> (refnum out=w1465:refnum<file>, error out=w1464:errorcluster)
            n973 = Close File(refnum=w1465, error in=w1464) -> ()  [unwired: 2 out]
          }
        }
      }
      event "模型": Value Change {
        n974 = event-data() -> ()  [unwired: 1 in, 6 out]
        n975 = global read "COD读取DATA全局.vi" "配置文件ini"() -> (w1475:string)
        n976 = call <vilib>:"Application Directory.vi"() -> ("Application Directory"=w1484:path)
        n977 = Build Path(base path=w1484, name or relative path=w1475) -> (appended path=w1483:path)
        n978 = call <vilib>:"Open Config Data.vi"("configuration file path"=w1483) -> ("error out"=w1481:errorcluster, "refnum"=w1482:T7)  [unwired: 8 in, 1 out]
        n979 = local read "模型"() -> (w1476:enum32{"线性", "多项式"})
        n980 = call-poly <vilib>:"Write Key.vi"("section"="CODMn模型选择" ("key"), "error in (no error)"=w1481, "value"=w1476, "key"="线性和多项式", "refnum"=w1482) -> ("error out"=w1477:errorcluster, "refnum out"=w1478:T7)  [unwired: 4 in, 1 out]
        n981 = call <vilib>:"Close Config Data.vi"("error in (no error)"=w1477, "refnum"=w1478) -> ()  [unwired: 8 in, 2 out]
      }
      event "浓度1", "浓度2", "浓度3", "泵滴定数1", "泵滴定数2", "泵滴定数3", "启用1", "启用2", "启用3", "浓度4", "浓度5", "泵滴定数4", "泵滴定数5", "启用4", "启用5": Value Change {
        n982 = event-data() -> ()  [unwired: 1 in, 6 out]
        n983 = global read "COD读取DATA全局.vi" "配置文件ini"() -> (w1485:string)
        n984 = local read "选用水样"() -> (w1501:enum16{"葡萄糖", "草酸钠"})
        n985 = local read "量程选择"() -> (w1500:enum16{"低量程", "高量程", "0-2量程"})
        n986 = case shown="\"0-2量程\"" w1500 {
          tunnel: ["低量程" "高量程" "0-2量程"] -> w1498
          frame "低量程", Default {
          }
          frame "高量程" {
          }
          frame "0-2量程" {
          }
        }
        n987 = call <vilib>:"Application Directory.vi"() -> ("Application Directory"=w1559:path)
        n988 = case shown="\"葡萄糖\", 默认" w1501 {
          tunnel: ["葡萄糖标线" ("section") "草酸钠标线" ("section")] -> w1507
          frame "葡萄糖", Default {
          }
          frame "草酸钠" {
          }
        }
        n989 = Build Path(base path=w1559, name or relative path=w1485) -> (appended path=w1558:path)
        n990 = call <vilib>:"Open Config Data.vi"("configuration file path"=w1558) -> ("error out"=w1556:errorcluster, "refnum"=w1557:T7)  [unwired: 8 in, 1 out]
        n991 = local read "浓度1"() -> (w1554:dbl)
        n992 = Concatenate Strings(w1507, w1498) -> (w1499:string)
        n993 = local read "浓度2"() -> (w1538:dbl)
        n994 = call-poly <vilib>:"Write Key.vi"("section"=w1499, "error in (no error)"=w1556, "value"=w1554, "key"="浓度1", "refnum"=w1557) -> ("error out"=w1553:errorcluster, "refnum out"=w1552:T7)  [unwired: 4 in, 1 out]
        n995 = local read "浓度3"() -> (w1534:dbl)
        n996 = call-poly <vilib>:"Write Key.vi"("section"=w1499, "error in (no error)"=w1553, "value"=w1538, "key"="浓度2", "refnum"=w1552) -> ("error out"=w1551:errorcluster, "refnum out"=w1550:T7)  [unwired: 4 in, 1 out]
        n997 = local read "泵滴定数1"() -> (w1532:dbl)
        n998 = call-poly <vilib>:"Write Key.vi"("section"=w1499, "error in (no error)"=w1551, "value"=w1534, "key"="浓度3", "refnum"=w1550) -> ("error out"=w1549:errorcluster, "refnum out"=w1548:T7)  [unwired: 4 in, 1 out]
        n999 = call-poly <vilib>:"Write Key.vi"("section"=w1499, "error in (no error)"=w1549, "value"=w1532, "key"="泵滴定数1", "refnum"=w1548) -> ("error out"=w1547:errorcluster, "refnum out"=w1546:T7)  [unwired: 4 in, 1 out]
        n1000 = local read "泵滴定数2"() -> (w1530:dbl)
        n1001 = call-poly <vilib>:"Write Key.vi"("section"=w1499, "error in (no error)"=w1547, "value"=w1530, "key"="泵滴定数2", "refnum"=w1546) -> ("error out"=w1545:errorcluster, "refnum out"=w1544:T7)  [unwired: 4 in, 1 out]
        n1002 = local read "泵滴定数3"() -> (w1528:dbl)
        n1003 = local read "浓度4"() -> (w1497:dbl)
        n1004 = call-poly <vilib>:"Write Key.vi"("section"=w1499, "error in (no error)"=w1545, "value"=w1528, "key"="泵滴定数3", "refnum"=w1544) -> ("error out"=w1543:errorcluster, "refnum out"=w1542:T7)  [unwired: 4 in, 1 out]
        n1005 = local read "浓度5"() -> (w1496:dbl)
        n1006 = call-poly <vilib>:"Write Key.vi"("section"=w1499, "error in (no error)"=w1543, "value"=w1497, "key"="浓度4", "refnum"=w1542) -> ("error out"=w1536:errorcluster, "refnum out"=w1537:T7)  [unwired: 4 in, 1 out]
        n1007 = call-poly <vilib>:"Write Key.vi"("section"=w1499, "error in (no error)"=w1536, "value"=w1496, "key"="浓度5", "refnum"=w1537) -> ("error out"=w1494:errorcluster, "refnum out"=w1495:T7)  [unwired: 4 in, 1 out]
        n1008 = local read "泵滴定数4"() -> (w1493:dbl)
        n1009 = call-poly <vilib>:"Write Key.vi"("section"=w1499, "error in (no error)"=w1494, "value"=w1493, "key"="泵滴定数4", "refnum"=w1495) -> ("error out"=w1541:errorcluster, "refnum out"=w1540:T7)  [unwired: 4 in, 1 out]
        n1010 = local read "泵滴定数5"() -> (w1492:dbl)
        n1011 = call-poly <vilib>:"Write Key.vi"("section"=w1499, "error in (no error)"=w1541, "value"=w1492, "key"="泵滴定数5", "refnum"=w1540) -> ("error out"=w1490:errorcluster, "refnum out"=w1491:T7)  [unwired: 4 in, 1 out]
        n1012 = local read "启用1"() -> (w1516:bool)
        n1013 = call-poly <vilib>:"Write Key.vi"("section"=w1499, "error in (no error)"=w1490, "value"=w1516, "key"="启用1", "refnum"=w1491) -> ("error out"=w1512:errorcluster, "refnum out"=w1515:T7)  [unwired: 4 in, 1 out]
        n1014 = local read "启用2"() -> (w1513:bool)
        n1015 = call-poly <vilib>:"Write Key.vi"("section"=w1499, "error in (no error)"=w1512, "value"=w1513, "key"="启用2", "refnum"=w1515) -> ("error out"=w1523:errorcluster, "refnum out"=w1522:T7)  [unwired: 4 in, 1 out]
        n1016 = local read "启用3"() -> (w1511:bool)
        n1017 = call-poly <vilib>:"Write Key.vi"("section"=w1499, "error in (no error)"=w1523, "value"=w1511, "key"="启用3", "refnum"=w1522) -> ("error out"=w1521:errorcluster, "refnum out"=w1520:T7)  [unwired: 4 in, 1 out]
        n1018 = local read "启用4"() -> (w1486:bool)
        n1019 = call-poly <vilib>:"Write Key.vi"("section"=w1499, "error in (no error)"=w1521, "value"=w1486, "key"="启用4", "refnum"=w1520) -> ("error out"=w1519:errorcluster, "refnum out"=w1518:T7)  [unwired: 4 in, 1 out]
        n1020 = local read "启用5"() -> (w1487:bool)
        n1021 = call-poly <vilib>:"Write Key.vi"("section"=w1499, "error in (no error)"=w1519, "value"=w1487, "key"="启用5", "refnum"=w1518) -> ("error out"=w1488:errorcluster, "refnum out"=w1489:T7)  [unwired: 4 in, 1 out]
        n1022 = local read "选用水样"() -> (w1506:enum16{"葡萄糖", "草酸钠"})
        n1023 = call-poly <vilib>:"Write Key.vi"("section"="标线选择", "error in (no error)"=w1488, "value"=w1506, "key"="选用水样", "refnum"=w1489) -> ("error out"=w1503:errorcluster, "refnum out"=w1504:T7)  [unwired: 4 in, 1 out]
        n1024 = call <vilib>:"Close Config Data.vi"("error in (no error)"=w1503, "refnum"=w1504) -> ()  [unwired: 8 in, 2 out]
      }
      event "读取": Value Change {
        (unwired) u16 94 ("number of holding registers")
        (unwired) u16 4616 ("starting address")
        n1025 = event-data() -> ()  [unwired: 1 in, 6 out]
        n1026 = Bundle By Name(cluster=cluster{"命令":string} {"命令"=""} ("元素"), "命令"="CODMn读取公式" ("名称（未命名）")) -> (w1565:cluster{"命令":string})
        n1027 = Enqueue Element(queue=w1569, element=w1565, error in (no error)=w1568) -> ()  [unwired: 1 in, 3 out]
      }
      event "写入": Mouse Down {
        n1028 = event-data() -> ()  [unwired: 1 in, 8 out]
        n1029 = Two Button Dialog(message="是否将上方方程系数K、B、X^2的值写入，写入会覆盖原有公式！" ("消息")) -> (T button?=w1570:bool)  [unwired: 2 in]
        n1030 = case shown="真" w1570 {
          frame False {
          }
          frame True {
            n1031 = local read "模型"() -> (w1577:enum32{"线性", "多项式"})
            n1032 = case shown="\"多项式\"" w1577 {
              tunnel: [w1581 w1624] -> w1575
              tunnel: [w1580 w1623] -> w1574
              frame "线性", Default {
                n1033 = local read "测量模式(公式)"() -> (w1582:u16)
                n1034 = case shown="1" w1582 {
                  tunnel: [u16 4626 ("starting address") w1589 w1594 w1599 w1604 w1609 w1614 w1619] -> w1581
                  frame 0, Default {
                  }
                  frame 1 {
                    n1035 = local read "量程选择"() -> (w1588:enum16{"低量程", "高量程", "0-2量程"})
                    n1036 = case shown="\"低量程\", 默认" w1588 {
                      tunnel: [u16 4626 ("starting address") u16 4632 ("starting address") u16 4638 ("starting address")] -> w1589
                      frame "低量程", Default {
                      }
                      frame "高量程" {
                      }
                      frame "0-2量程" {
                      }
                    }
                  }
                  frame 2 {
                    n1037 = local read "量程选择"() -> (w1593:enum16{"低量程", "高量程", "0-2量程"})
                    n1038 = case shown="\"低量程\", 默认" w1593 {
                      tunnel: [u16 4638 ("starting address") u16 4644 ("starting address") u16 4638 ("starting address")] -> w1594
                      frame "低量程", Default {
                      }
                      frame "高量程" {
                      }
                      frame "0-2量程" {
                      }
                    }
                  }
                  frame 3 {
                    n1039 = local read "量程选择"() -> (w1598:enum16{"低量程", "高量程", "0-2量程"})
                    n1040 = case shown="\"低量程\", 默认" w1598 {
                      tunnel: [u16 4650 ("starting address") u16 4656 ("starting address") u16 4638 ("starting address")] -> w1599
                      frame "低量程", Default {
                      }
                      frame "高量程" {
                      }
                      frame "0-2量程" {
                      }
                    }
                  }
                  frame 4 {
                    n1041 = local read "量程选择"() -> (w1603:enum16{"低量程", "高量程", "0-2量程"})
                    n1042 = case shown="\"低量程\", 默认" w1603 {
                      tunnel: [u16 4662 ("starting address") u16 4668 ("starting address") u16 4638 ("starting address")] -> w1604
                      frame "低量程", Default {
                      }
                      frame "高量程" {
                      }
                      frame "0-2量程" {
                      }
                    }
                  }
                  frame 5 {
                    n1043 = local read "量程选择"() -> (w1608:enum16{"低量程", "高量程", "0-2量程"})
                    n1044 = case shown="\"低量程\", 默认" w1608 {
                      tunnel: [u16 4674 ("starting address") u16 4680 ("starting address") u16 4638 ("starting address")] -> w1609
                      frame "低量程", Default {
                      }
                      frame "高量程" {
                      }
                      frame "0-2量程" {
                      }
                    }
                  }
                  frame 6 {
                    n1045 = local read "量程选择"() -> (w1613:enum16{"低量程", "高量程", "0-2量程"})
                    n1046 = case shown="\"低量程\", 默认" w1613 {
                      tunnel: [u16 4686 ("starting address") u16 4692 ("starting address") u16 4638 ("starting address")] -> w1614
                      frame "低量程", Default {
                      }
                      frame "高量程" {
                      }
                      frame "0-2量程" {
                      }
                    }
                  }
                  frame 7 {
                    n1047 = local read "量程选择"() -> (w1618:enum16{"低量程", "高量程", "0-2量程"})
                    n1048 = case shown="\"低量程\", 默认" w1618 {
                      tunnel: [u16 4698 ("starting address") u16 4704 ("starting address") u16 4638 ("starting address")] -> w1619
                      frame "低量程", Default {
                      }
                      frame "高量程" {
                      }
                      frame "0-2量程" {
                      }
                    }
                  }
                }
                n1049 = local read "K"() -> (w1586:dbl)
                n1050 = local read "b"() -> (w1585:dbl)
                n1051 = Build Array(w1586, w1585, 0.0 ("元素")) -> (w1584:dbl[])
                n1052 = call "浮点转CDAB整形cod.vi"("浮点数"=w1584) -> ("CDAB整形输出"=w1580:u16[])  [unwired: 10 in]
              }
              frame "多项式" {
                # "b,k,c"
                n1053 = local read "测量模式(公式)"() -> (w1625:u16)
                n1054 = case shown="1" w1625 {
                  tunnel: [u16 4626 ("starting address") w1633 w1638 w1643 w1648 w1653 w1658 w1663] -> w1624
                  frame 0, Default {
                  }
                  frame 1 {
                    n1055 = local read "量程选择"() -> (w1632:enum16{"低量程", "高量程", "0-2量程"})
                    n1056 = case shown="\"低量程\", 默认" w1632 {
                      tunnel: [u16 4626 ("starting address") u16 4632 ("starting address") u16 4638 ("starting address")] -> w1633
                      frame "低量程", Default {
                      }
                      frame "高量程" {
                      }
                      frame "0-2量程" {
                      }
                    }
                  }
                  frame 2 {
                    n1057 = local read "量程选择"() -> (w1637:enum16{"低量程", "高量程", "0-2量程"})
                    n1058 = case shown="\"低量程\", 默认" w1637 {
                      tunnel: [u16 4638 ("starting address") u16 4644 ("starting address") u16 4638 ("starting address")] -> w1638
                      frame "低量程", Default {
                      }
                      frame "高量程" {
                      }
                      frame "0-2量程" {
                      }
                    }
                  }
                  frame 3 {
                    n1059 = local read "量程选择"() -> (w1642:enum16{"低量程", "高量程", "0-2量程"})
                    n1060 = case shown="\"低量程\", 默认" w1642 {
                      tunnel: [u16 4650 ("starting address") u16 4656 ("starting address") u16 4638 ("starting address")] -> w1643
                      frame "低量程", Default {
                      }
                      frame "高量程" {
                      }
                      frame "0-2量程" {
                      }
                    }
                  }
                  frame 4 {
                    n1061 = local read "量程选择"() -> (w1647:enum16{"低量程", "高量程", "0-2量程"})
                    n1062 = case shown="\"低量程\", 默认" w1647 {
                      tunnel: [u16 4662 ("starting address") u16 4668 ("starting address") u16 4638 ("starting address")] -> w1648
                      frame "低量程", Default {
                      }
                      frame "高量程" {
                      }
                      frame "0-2量程" {
                      }
                    }
                  }
                  frame 5 {
                    n1063 = local read "量程选择"() -> (w1652:enum16{"低量程", "高量程", "0-2量程"})
                    n1064 = case shown="\"低量程\", 默认" w1652 {
                      tunnel: [u16 4674 ("starting address") u16 4680 ("starting address") u16 4638 ("starting address")] -> w1653
                      frame "低量程", Default {
                      }
                      frame "高量程" {
                      }
                      frame "0-2量程" {
                      }
                    }
                  }
                  frame 6 {
                    n1065 = local read "量程选择"() -> (w1657:enum16{"低量程", "高量程", "0-2量程"})
                    n1066 = case shown="\"低量程\", 默认" w1657 {
                      tunnel: [u16 4686 ("starting address") u16 4692 ("starting address") u16 4638 ("starting address")] -> w1658
                      frame "低量程", Default {
                      }
                      frame "高量程" {
                      }
                      frame "0-2量程" {
                      }
                    }
                  }
                  frame 7 {
                    n1067 = local read "量程选择"() -> (w1662:enum16{"低量程", "高量程", "0-2量程"})
                    n1068 = case shown="\"低量程\", 默认" w1662 {
                      tunnel: [u16 4698 ("starting address") u16 4704 ("starting address") u16 4638 ("starting address")] -> w1663
                      frame "低量程", Default {
                      }
                      frame "高量程" {
                      }
                      frame "0-2量程" {
                      }
                    }
                  }
                }
                n1069 = local read "多项式系数"() -> (w1630:dbl[])
                n1070 = Index Array(array=w1630) -> (element #1=w1627:dbl, element #2=w1628:dbl, element #3=w1626:dbl)  [unwired: 3 in]
                n1071 = Build Array(w1628, w1627, w1626) -> (w1629:dbl[])
                n1072 = call "浮点转CDAB整形cod.vi"("浮点数"=w1629) -> ("CDAB整形输出"=w1623:u16[])  [unwired: 10 in]
              }
            }
            n1073 = call "CODMnMB_api.vi"("STEP"=enum16{"open", "read", "write", "close"}."write", "values"=w1574, "starting address"=w1575) -> ("error out"=w1573:errorcluster)  [unwired: 6 in, 2 out]
            n1074 = case shown="错误" w1573 {
              tunnel: ["写入成功！" "写入失败！"] -> w1572
              frame No Error {
              }
              frame Error {
              }
            }
            n1075 = One Button Dialog(message=w1572) -> ()  [unwired: 1 in, 1 out]
          }
        }
      }
      event "一键写入": Value Change {
        n1076 = event-data() -> ()  [unwired: 1 in, 6 out]
        n1077 = Two Button Dialog(message="确认是否写入公式，写入会覆盖原有公式！" ("消息")) -> (T button?=w1667:bool)  [unwired: 2 in]
        n1078 = case shown="真" w1667 {
          frame False {
          }
          frame True {
            n1079 = local read "模型"() -> (w1671:enum32{"线性", "多项式"})
            n1080 = case shown="\"多项式\"" w1671 {
              tunnel: [w1674 w1725] -> w1669
              frame "线性", Default {
                n1081 = property on="测量模式(公式)" class="Ring (严格)"() -> ("NumItems"=w1675:u32)  [unwired: 2 in, 2 out]
                n1082 = for {
                  N: w1675 -> [_]
                  tunnel: [w1676] -> w1674
                  i -> [w1681]
                  n1083 = Increment(x=w1681) -> (x+1=w1680:i32)
                  n1084 = local read "K"() -> (w1685:dbl)
                  n1085 = case shown="1" w1680 {
                    tunnel: [u16 4626 ("starting address") w1691 w1696 w1701 w1706 w1711 w1716 w1721] -> w1678
                    frame 0, Default {
                    }
                    frame 1 {
                      n1086 = local read "量程选择"() -> (w1690:enum16{"低量程", "高量程", "0-2量程"})
                      n1087 = case shown="\"低量程\", 默认" w1690 {
                        tunnel: [u16 4626 ("starting address") u16 4632 ("starting address") u16 4638 ("starting address")] -> w1691
                        frame "低量程", Default {
                        }
                        frame "高量程" {
                        }
                        frame "0-2量程" {
                        }
                      }
                    }
                    frame 2 {
                      n1088 = local read "量程选择"() -> (w1695:enum16{"低量程", "高量程", "0-2量程"})
                      n1089 = case shown="\"低量程\", 默认" w1695 {
                        tunnel: [u16 4638 ("starting address") u16 4644 ("starting address") u16 4638 ("starting address")] -> w1696
                        frame "低量程", Default {
                        }
                        frame "高量程" {
                        }
                        frame "0-2量程" {
                        }
                      }
                    }
                    frame 3 {
                      n1090 = local read "量程选择"() -> (w1700:enum16{"低量程", "高量程", "0-2量程"})
                      n1091 = case shown="\"低量程\", 默认" w1700 {
                        tunnel: [u16 4650 ("starting address") u16 4656 ("starting address") u16 4638 ("starting address")] -> w1701
                        frame "低量程", Default {
                        }
                        frame "高量程" {
                        }
                        frame "0-2量程" {
                        }
                      }
                    }
                    frame 4 {
                      n1092 = local read "量程选择"() -> (w1705:enum16{"低量程", "高量程", "0-2量程"})
                      n1093 = case shown="\"高量程\"" w1705 {
                        tunnel: [u16 4662 ("starting address") u16 4668 ("starting address") u16 4638 ("starting address")] -> w1706
                        frame "低量程", Default {
                        }
                        frame "高量程" {
                        }
                        frame "0-2量程" {
                        }
                      }
                    }
                    frame 5 {
                      n1094 = local read "量程选择"() -> (w1710:enum16{"低量程", "高量程", "0-2量程"})
                      n1095 = case shown="\"低量程\", 默认" w1710 {
                        tunnel: [u16 4674 ("starting address") u16 4680 ("starting address") u16 4638 ("starting address")] -> w1711
                        frame "低量程", Default {
                        }
                        frame "高量程" {
                        }
                        frame "0-2量程" {
                        }
                      }
                    }
                    frame 6 {
                      n1096 = local read "量程选择"() -> (w1715:enum16{"低量程", "高量程", "0-2量程"})
                      n1097 = case shown="\"低量程\", 默认" w1715 {
                        tunnel: [u16 4686 ("starting address") u16 4692 ("starting address") u16 4638 ("starting address")] -> w1716
                        frame "低量程", Default {
                        }
                        frame "高量程" {
                        }
                        frame "0-2量程" {
                        }
                      }
                    }
                    frame 7 {
                      n1098 = local read "量程选择"() -> (w1720:enum16{"低量程", "高量程", "0-2量程"})
                      n1099 = case shown="\"低量程\", 默认" w1720 {
                        tunnel: [u16 4698 ("starting address") u16 4704 ("starting address") u16 4638 ("starting address")] -> w1721
                        frame "低量程", Default {
                        }
                        frame "高量程" {
                        }
                        frame "0-2量程" {
                        }
                      }
                    }
                  }
                  n1100 = local read "b"() -> (w1686:dbl)
                  n1101 = Build Array(w1685, w1686, 0.0 ("元素")) -> (w1687:dbl[])
                  n1102 = call "浮点转CDAB整形cod.vi"("浮点数"=w1687) -> ("CDAB整形输出"=w1684:u16[])  [unwired: 10 in]
                  n1103 = Insert Into Array(array=u16[] [], index=0 ("索引"), new element=w1684) -> (w1677:u16[])
                  n1104 = call "CODMnMB_api.vi"("STEP"=enum16{"open", "read", "write", "close"}."write", "values"=w1677, "starting address"=w1678) -> ("error out"=w1676:errorcluster)  [unwired: 6 in, 2 out]
                }
              }
              frame "多项式" {
                # "b,k,c"
                n1105 = property on="测量模式(公式)" class="Ring (严格)"() -> ("NumItems"=w1726:u32)  [unwired: 2 in, 2 out]
                n1106 = for {
                  N: w1726 -> [_]
                  tunnel: [w1727] -> w1725
                  i -> [w1732]
                  n1107 = local read "多项式系数"() -> (w1736:dbl[])
                  n1108 = Increment(x=w1732) -> (x+1=w1731:i32)
                  n1109 = case shown="2" w1731 {
                    tunnel: [u16 4626 ("starting address") w1743 w1748 w1753 w1758 w1763 w1768 w1773] -> w1728
                    frame 0, Default {
                    }
                    frame 1 {
                      n1110 = local read "量程选择"() -> (w1742:enum16{"低量程", "高量程", "0-2量程"})
                      n1111 = case shown="\"低量程\", 默认" w1742 {
                        tunnel: [u16 4626 ("starting address") u16 4632 ("starting address") u16 4638 ("starting address")] -> w1743
                        frame "低量程", Default {
                        }
                        frame "高量程" {
                        }
                        frame "0-2量程" {
                        }
                      }
                    }
                    frame 2 {
                      n1112 = local read "量程选择"() -> (w1747:enum16{"低量程", "高量程", "0-2量程"})
                      n1113 = case shown="\"低量程\", 默认" w1747 {
                        tunnel: [u16 4638 ("starting address") u16 4644 ("starting address") u16 4638 ("starting address")] -> w1748
                        frame "低量程", Default {
                        }
                        frame "高量程" {
                        }
                        frame "0-2量程" {
                        }
                      }
                    }
                    frame 3 {
                      n1114 = local read "量程选择"() -> (w1752:enum16{"低量程", "高量程", "0-2量程"})
                      n1115 = case shown="\"低量程\", 默认" w1752 {
                        tunnel: [u16 4650 ("starting address") u16 4656 ("starting address") u16 4638 ("starting address")] -> w1753
                        frame "低量程", Default {
                        }
                        frame "高量程" {
                        }
                        frame "0-2量程" {
                        }
                      }
                    }
                    frame 4 {
                      n1116 = local read "量程选择"() -> (w1757:enum16{"低量程", "高量程", "0-2量程"})
                      n1117 = case shown="\"低量程\", 默认" w1757 {
                        tunnel: [u16 4662 ("starting address") u16 4668 ("starting address") u16 4638 ("starting address")] -> w1758
                        frame "低量程", Default {
                        }
                        frame "高量程" {
                        }
                        frame "0-2量程" {
                        }
                      }
                    }
                    frame 5 {
                      n1118 = local read "量程选择"() -> (w1762:enum16{"低量程", "高量程", "0-2量程"})
                      n1119 = case shown="\"低量程\", 默认" w1762 {
                        tunnel: [u16 4674 ("starting address") u16 4680 ("starting address") u16 4638 ("starting address")] -> w1763
                        frame "低量程", Default {
                        }
                        frame "高量程" {
                        }
                        frame "0-2量程" {
                        }
                      }
                    }
                    frame 6 {
                      n1120 = local read "量程选择"() -> (w1767:enum16{"低量程", "高量程", "0-2量程"})
                      n1121 = case shown="\"低量程\", 默认" w1767 {
                        tunnel: [u16 4686 ("starting address") u16 4692 ("starting address") u16 4638 ("starting address")] -> w1768
                        frame "低量程", Default {
                        }
                        frame "高量程" {
                        }
                        frame "0-2量程" {
                        }
                      }
                    }
                    frame 7 {
                      n1122 = local read "量程选择"() -> (w1772:enum16{"低量程", "高量程", "0-2量程"})
                      n1123 = case shown="\"低量程\", 默认" w1772 {
                        tunnel: [u16 4698 ("starting address") u16 4704 ("starting address") u16 4638 ("starting address")] -> w1773
                        frame "低量程", Default {
                        }
                        frame "高量程" {
                        }
                        frame "0-2量程" {
                        }
                      }
                    }
                  }
                  n1124 = Index Array(array=w1736) -> (element #1=w1739:dbl, element #2=w1738:dbl, element #3=w1740:dbl)  [unwired: 3 in]
                  n1125 = Build Array(w1738, w1739, w1740) -> (w1737:dbl[])
                  n1126 = call "浮点转CDAB整形cod.vi"("浮点数"=w1737) -> ("CDAB整形输出"=w1735:u16[])  [unwired: 10 in]
                  n1127 = Insert Into Array(array=u16[] [], index=0 ("索引"), new element=w1735) -> (w1729:u16[])
                  n1128 = call "CODMnMB_api.vi"("STEP"=enum16{"open", "read", "write", "close"}."write", "values"=w1729, "starting address"=w1728) -> ("error out"=w1727:errorcluster)  [unwired: 6 in, 2 out]
                }
              }
            }
            n1129 = case shown="无错误" w1669 {
              tunnel: ["写入成功！" "写入失败！"] -> w1670
              frame No Error {
              }
              frame Error {
              }
            }
            n1130 = One Button Dialog(message=w1670) -> ()  [unwired: 1 in, 1 out]
          }
        }
      }
      event "滴定曲线": Value Change {
        n1131 = event-data() -> ()  [unwired: 1 in, 6 out]
        n1132 = property on="窗格" class="Pane"("Origin"=T17 {"Horizontal"=0, "Vertical"=3200} ("原点")) -> ()  [unwired: 2 in, 2 out]
      }
      event "历史波形": Value Change {
        n1133 = event-data() -> ()  [unwired: 1 in, 6 out]
        n1134 = call-poly <vilib>:"Read Waveforms from File.vi"() -> ("error out"=w1778:errorcluster, "first waveform in record"=w1779:waveform(dbl))  [unwired: 6 in, 2 out]
        n1135 = case shown="无错误" w1778 {
          tunnel: w1779 -> [w1782 _]
          frame No Error {
            n1136 = Unbundle By Name(w1782) -> ("t0"=→"波形时间":timestamp, "Y"=w1781:dbl[])  [unwired: 2 out]
            n1137 = local write "滴定数-ORP值"(w1781) -> ()
            n1138 = local write "ORP滴定曲线"(w1781) -> ()
          }
          frame Error {
            n1139 = One Button Dialog(message="打开失败" ("消息")) -> ()  [unwired: 1 in, 1 out]
          }
        }
      }
      event "释放串口": Value Change {
        n1140 = event-data() -> ()  [unwired: 1 in, 6 out]
        n1141 = Two Button Dialog(message="确认是否释放串口，释放串口将导致通信失败！" ("消息")) -> (T button?=w1784:bool)  [unwired: 2 in]
        n1142 = case shown="真" w1784 {
          tunnel: w1787 -> [_ w1789]
          tunnel: w1786 -> [_ w1788]
          frame False {
          }
          frame True {
            n1143 = Bundle By Name(cluster=cluster{"命令":string} {"命令"=""} ("元素"), "命令"="停用模块" ("名称（未命名）")) -> (w1790:cluster{"命令":string})
            n1144 = Enqueue Element(queue=w1789, element=w1790, error in (no error)=w1788) -> ()  [unwired: 1 in, 3 out]
          }
        }
      }
      event "打开串口": Value Change {
        n1145 = event-data() -> ()  [unwired: 1 in, 6 out]
        n1146 = flat-sequence {
          tunnel: w1794 -> [w1802]
          tunnel: w1793 -> [w1801]
          frame #0 {
            n1147 = global read "CODMn断电保存全局变量.vi" "MB通信方式选择"() -> (w1798:enum16{"串口", "TCP"})
            n1148 = global read "CODMn断电保存全局变量.vi" "VISA resource name"() -> (w1805:refnum<visa-resource-name>)
            n1149 = global read "CODMn断电保存全局变量.vi" "PORT"() -> (w1796:string)
            n1150 = global read "CODMn断电保存全局变量.vi" "IP"() -> (w1797:string)
            n1151 = call "串口配置.vi"("PORT"=w1796, "IP"=w1797, "MB通信方式选择"=w1798, "请选择串口:"=w1805) -> ("PORT 2"=w1799:string, "IP 2"=w1800:string, "确认 2"=w1803:bool, "VISA资源名称 2"=w1804:refnum<visa-resource-name>, "MB通信方式选择 2"=w1795:enum16{"串口", "TCP"})  [unwired: 3 in]
            n1152 = case shown="真" w1803 {
              tunnel: w1804 -> [_ w1814]
              tunnel: w1802 -> [_ w1810]
              tunnel: w1801 -> [_ w1809]
              tunnel: w1800 -> [_ w1808]
              tunnel: w1799 -> [_ w1807]
              tunnel: w1795 -> [_ w1806]
              frame False {
              }
              frame True {
                n1153 = global write "CODMn断电保存全局变量.vi" "MB通信方式选择"(w1806) -> ()
                n1154 = global write "CODMn断电保存全局变量.vi" "VISA resource name"(w1814) -> ()
                n1155 = global write "CODMn断电保存全局变量.vi" "PORT"(w1807) -> ()
                n1156 = global write "CODMn断电保存全局变量.vi" "IP"(w1808) -> ()
                n1157 = Bundle By Name(cluster=cluster{"命令":string} {"命令"=""} ("元素"), "命令"="启用模块" ("名称（未命名）")) -> (w1811:cluster{"命令":string})
                n1158 = Enqueue Element(queue=w1810, element=w1811, error in (no error)=w1809) -> ()  [unwired: 1 in, 3 out]
              }
            }
          }
          frame #1 {
            n1159 = global read "COD读取DATA全局.vi" "配置文件ini"() -> (w1828:string)
            n1160 = call <vilib>:"Application Directory.vi"() -> ("Application Directory"=w1815:path)
            n1161 = Build Path(base path=w1815, name or relative path=w1828) -> (appended path=w1816:path)
            n1162 = call <vilib>:"Open Config Data.vi"("configuration file path"=w1816) -> ("error out"=w1820:errorcluster, "refnum"=w1817:T7)  [unwired: 8 in, 1 out]
            n1163 = vi-ref "斯坦道CODMn.lvlib:CODMn断电保存全局变量.vi"() -> (w1818:refnum<vi>)
            n1164 = call <userlib>:"Write Panel to INI__ogtk.vi"("error in (no error)"=w1820, "VI ref"=w1818, "refnum"=w1817) -> ("error out"=w1821:errorcluster, "refnum out"=w1819:T7)  [unwired: 7 in]
            n1165 = call <vilib>:"Close Config Data.vi"("error in (no error)"=w1821, "refnum"=w1819) -> ("error out"=w1826:errorcluster, "file path"=w1827:path)  [unwired: 8 in]
            n1166 = Open/Create/Replace File(file path (use dialog)=w1827, error in=w1826) -> (refnum out=w1823:refnum<file>, error out=w1822:errorcluster)  [unwired: 4 in, 1 out]
            n1167 = Flush File(refnum=w1823, error in=w1822) -> (refnum out=w1824:refnum<file>, error out=w1825:errorcluster)
            n1168 = Close File(refnum=w1824, error in=w1825) -> ()  [unwired: 2 out]
          }
        }
      }
      event Timeout {
        n1169 = event-data() -> ()  [unwired: 1 in, 3 out]
      }
    }
  }
  n1170 = while {
    tunnel: w3 -> [w1834]
    tunnel: w2 -> [w1833]
    tunnel: [w1829] -> _
    stop <- FALSE stop-if-true
    # "CODMn与外部交互"
    n1171 = Dequeue Element(queue=w1834, error in (no error)=w1833) -> (element=w1835:T3)  [unwired: 1 in, 3 out]
    n1172 = Unbundle By Name(w1835) -> ("命令"=w1832:string, "测量模式"=w1831:T18, "CODMn量程切换"=w1830:enum32{"H", "L", "AUTO"})
    n1173 = case shown="\"启动命令\"" w1832 {
      tunnel: w1831 -> [_ w1838 _ _]
      tunnel: w1830 -> [_ _ _ w1868]
      tunnel: [_ w1837 w1863 w1867] -> w1829
      frame "假", Default {
      }
      frame "启动命令" {
        n1174 = case shown="\"标样核查\"" w1838 {
          tunnel: [u16 4608 ("address") u16 4608 ("address") u16 4608 ("address") u16 4608 ("address") u16 4608 ("address") u16 4608 ("address") u16 4608 ("address") u16 4608 ("address") u16 4608 ("address")] -> w1840
          tunnel: [u16 1 ("address") u16 2 ("address") u16 3 ("address") u16 4 ("address") u16 5 ("address") u16 7 ("address") u16 6 ("address") u16 8 ("address") u16 9 ("address")] -> w1844
          frame "水样测量" {
          }
          frame "标样核查" {
          }
          frame "零点核查" {
          }
          frame "跨度核查" {
          }
          frame "空白测试" {
          }
          frame "加标回收" {
          }
          frame "平行样" {
          }
          frame "校零" {
          }
          frame "校标" {
          }
        }
        n1175 = Insert Into Array(array=u16[] [] ("values"), index=0 ("索引"), new element=w1844) -> (w1839:u16[])
        n1176 = call "CODMnMB_api.vi"("STEP"=enum16{"open", "read", "write", "close"}."write", "values"=w1839, "starting address"=w1840) -> ("error out"=w1837:errorcluster)  [unwired: 6 in, 2 out]
      }
      frame "停止命令" {
        n1177 = call "CODMnMB_api.vi"("STEP"=enum16{"open", "read", "write", "close"}."write", "values"=u16[] [11], "starting address"=u16 4608) -> ("error out"=w1863:errorcluster)  [unwired: 6 in, 2 out]
      }
      frame "量程切换" {
        n1178 = case shown="\"H\"" w1868 {
          tunnel: [u16[] [1] ("values") u16[] [0] ("values") _] -> w1871
          frame "H" {
          }
          frame "L" {
          }
          frame "AUTO", Default {
          }
        }
        n1179 = call "CODMnMB_api.vi"("STEP"=enum16{"open", "read", "write", "close"}."write", "values"=w1871, "starting address"=u16 4276) -> ("error out"=w1867:errorcluster)  [unwired: 6 in, 2 out]
      }
    }
  }
  n1180 = while {
    tunnel: w17 -> [w1883]
    tunnel: w16 -> [w1882]
    tunnel: w8 -> [_]
    stop <- FALSE stop-if-true
    # "主循环界面显示"
    n1181 = flat-sequence {
      frame #0 {
        # "测量状态显示"
        n1182 = global read "COD读取DATA全局.vi" "测量状态"() -> (w1917:u16[])
        n1183 = To Word Integer(number=w1917) -> (16bit integer=w1928:i16[])
        n1184 = Index Array(array=w1928, index #1=0 ("索引"), index #4=3 ("索引"), index #14=13 ("索引"), index #15=14 ("索引"), index #21=20 ("索引"), index #32=31 ("索引")) -> (element #1=w1933:i16, element #2=w1932:i16, element #3=w1931:i16, element #4=→"CODMn工作状态":i16, element #5=→"模式（受控）":i16, element #6=→"进样管":i16, element #7=→"高锰酸钾":i16, element #8=→"草酸钠":i16, element #9=→"硫酸":i16, element #10=w1927:i16, element #11=w1948:i16, element #12=w1923:i16, element #13=→"报警数字":i16, element #14=w1954:i16, element #15=w1939:i16, element #16=→"多列列表框":i16, element #21=w1915:i16, element #33=→"分":i16, element #34=→"秒":i16)  [unwired: 28 in, 15 out]
        n1185 = Number To Decimal String(number=w1915) -> (decimal integer string=→"基本量程(显示)":string)  [unwired: 1 in]
        n1186 = global write "COD读取DATA全局.vi" "基本量程存储数据用"(w1915) -> ()
        n1187 = Build Array(w1933, w1932, w1931) -> (w1934:i16[])
        n1188 = To Single Precision Float(number=w1927) -> (single precision float=→"ORP显示":sgl)
        n1189 = call "HexToDate.vi"("数组"=w1934) -> ("DATE"=w1929:timestamp[])  [unwired: 10 in]
        n1190 = Index Array(array=w1929) -> (element=→"仪器时间":timestamp)  [unwired: 1 in]
        n1191 = Divide(x=w1948, y=u16 10) -> (x/y=→"温度":dbl)
        n1192 = Divide(x=w1939, y=u16 1000) -> (x/y=→"标度滴定值":dbl)
        n1193 = Equal?(x=w1923, y=u16 2) -> (x = y?=→"断电排液标记":bool)
        n1194 = Equal?(x=w1923, y=u16 1) -> (x = y?=→"排液标记":bool)
        n1195 = Divide(x=w1954, y=u16 1000) -> (x/y=→"零点滴定值":dbl)
      }
    }
    n1196 = flat-sequence {
      frame #0 {
        # "工作状态显示"
        n1197 = local read "CODMn工作状态"() -> (w1892:T1)
        n1198 = Equal?(x=w1892, y=u16 0) -> (x = y?=→"待机":bool)
        n1199 = Equal?(x=w1892, y=u16 8) -> (x = y?=→"校零标记":bool)
        n1200 = Equal?(x=w1892, y=u16 9) -> (x = y?=→"校标标记":bool)
        n1201 = Equal?(x=w1892, y=u16 1) -> (x = y?=→"水样测量":bool)
        n1202 = Equal?(x=w1892, y=u16 7) -> (x = y?=→"质控样测量":bool)
        n1203 = Equal?(x=w1892, y=u16 10) -> (x = y?=→"加标回收测量":bool)
        n1204 = Equal?(x=w1892, y=u16 2) -> (x = y?=→"标样核查标记":bool)
        n1205 = Equal?(x=w1892, y=u16 6) -> (x = y?=→"平行样测量":bool)
        n1206 = Equal?(x=w1892, y=u16 3) -> (x = y?=→"零点核查标记":bool)
        n1207 = Equal?(x=w1892, y=u16 4) -> (x = y?=→"跨度核查标记":bool)
        n1208 = Equal?(x=w1892, y=u16 5) -> (x = y?=→"空白测试标记":bool)
      }
    }
    n1209 = First Call?() -> (First Call?: T/F=w1881:bool)
    n1210 = case shown="真" w1881 {
      tunnel: w1883 -> [w1982 w1987]
      tunnel: w1882 -> [w1981 w1986]
      tunnel: [w1982 w1985] -> w1879
      tunnel: [w1981 w1984] -> w1878
      frame False {
      }
      frame True {
        n1211 = Bundle By Name(cluster=cluster{"命令":string} {"命令"=""} ("元素"), "命令"="CODMn读取参数" ("名称（未命名）")) -> (w1990:cluster{"命令":string})
        n1212 = Enqueue Element(queue=w1987, element=w1990, timeout in ms (-1)=1000 ("超时毫秒(-1)"), error in (no error)=w1986) -> (queue out=w1985:refnum<queue>, error out=w1984:errorcluster)  [unwired: 1 out]
      }
    }
    n1213 = Wait (ms)(milliseconds to wait=u32 1000 ("等待时间（毫秒）")) -> ()  [unwired: 1 out]
    n1214 = Get Queue Status(queue=w1879, error in (no error)=w1878) -> (queue out=w1875:refnum<queue>, error out=w1874:errorcluster, # elements in queue=w1877:i32)  [unwired: 1 in, 5 out]
    n1215 = Equal To 0?(x=w1877) -> (x = 0?=w1876:bool)
    n1216 = flat-sequence {
      frame #0 {
        # "CODMn读取状态"
        n1217 = global read "COD读取DATA全局.vi" "M输出点"() -> (w2001:bool[])
        n1218 = global read "COD读取DATA全局.vi" "温度"() -> (w2002:bool[])
        n1219 = Index Array(array=w2002) -> (element=→"加热":bool)  [unwired: 1 in]
        n1220 = Index Array(array=w2001) -> (element #1=→"搅拌":bool, element #4=→"进水样":bool, element #5=→"进蒸馏水":bool, element #6=→"进标液":bool, element #7=→"进零点核查样":bool, element #8=→"进加标回收样":bool, element #9=→"进高锰酸钾":bool, element #10=→"进草酸钠":bool, element #11=→"进硫酸":bool)  [unwired: 11 in, 2 out]
      }
    }
    n1221 = case shown="真" w1876 {
      tunnel: w1875 -> [_ w1887]
      tunnel: w1874 -> [_ w1886]
      frame False {
      }
      frame True {
        n1222 = Bundle By Name(cluster=cluster{"命令":string} {"命令"=""} ("元素"), "命令"="CODMn读取" ("名称（未命名）")) -> (w1889:cluster{"命令":string})
        n1223 = Enqueue Element(queue=w1887, element=w1889, timeout in ms (-1)=1000 ("超时毫秒(-1)"), error in (no error)=w1886) -> ()  [unwired: 3 out]
      }
    }
    n1224 = Get Date/Time In Seconds() -> (seconds since 1Jan1904=→"系统时间":timestamp)
    n1225 = flat-sequence {
      frame #0 {
        # "A，B，K"
        # "CODMn读取状态"
        n1226 = global read "COD读取DATA全局.vi" "ORP、时间"() -> (w2005:u16[])
        n1227 = To Word Integer(number=w2005) -> (16bit integer=w2026:i16[])
        n1228 = Split 1D Array(array=w2026, index=3 ("索引")) -> (first subarray=w2007:i16[], second subarray=w2025:i16[])
        n1229 = Index Array(array=w2007) -> (element #1=w2011:i16, element #2=w2010:i16, element #3=w2009:i16)  [unwired: 3 in]
        n1230 = Index Array(array=w2025) -> (element #1=w2020:i16, element #2=w2024:i16, element #3=w2023:i16, element #4=w2022:i16)  [unwired: 4 in]
        n1231 = Build Array(w2011, w2010, w2009) -> (w2008:i16[])
        n1232 = To Single Precision Float(number=w2023) -> (single precision float=w2014:sgl)
        n1233 = To Single Precision Float(number=w2020) -> (single precision float=w2019:sgl)
        n1234 = To Single Precision Float(number=w2024) -> (single precision float=w2018:sgl)
        n1235 = To Single Precision Float(number=w2022) -> (single precision float=w2013:sgl)
        n1236 = call "HexToDate.vi"("数组"=w2008) -> ("DATE"=w2012:timestamp[])  [unwired: 10 in]
        n1237 = Divide(x=w2019, y=sgl 100.0) -> (x/y=→"COD浓度（mg/L)":sgl)
        n1238 = Index Array(array=w2012) -> (element=w2006:timestamp)  [unwired: 1 in]
        n1239 = Number To Decimal String(number=w2018) -> (decimal integer string=→"ORP-A":string)  [unwired: 1 in]
        n1240 = Number To Decimal String(number=w2014) -> (decimal integer string=→"ORP-B":string)  [unwired: 1 in]
        n1241 = Number To Decimal String(number=w2013) -> (decimal integer string=→"ORP-K":string)  [unwired: 1 in]
        n1242 = Format Date/Time String(seconds (now)=w2006) -> (date/time string=→"数据时间":string)  [unwired: 2 in]
      }
    }
    n1243 = flat-sequence {
      frame #0 {
        # "报警状态显示"
        n1244 = local read "报警数字"() -> (w1957:i16)
        n1245 = Equal?(x=w1957, y=u16 9) -> (x = y?=w1960:bool)
        "进水样超量程" <- w1960
        n1246 = Equal?(x=w1957, y=u16 10) -> (x = y?=w1959:bool)
        "排液故障" <- w1959
        n1247 = Equal?(x=w1957, y=u16 2) -> (x = y?=w1967:bool)
        "温控器故障" <- w1967
        n1248 = Equal?(x=w1957, y=u16 3) -> (x = y?=w1966:bool)
        "加热故障" <- w1966
        n1249 = Equal?(x=w1957, y=u16 4) -> (x = y?=w1965:bool)
        "高锰酸钾报警" <- w1965
        n1250 = Equal?(x=w1957, y=u16 5) -> (x = y?=w1964:bool)
        "草酸钠报警" <- w1964
        n1251 = Equal?(x=w1957, y=u16 6) -> (x = y?=w1963:bool)
        "测量错误" <- w1963
        n1252 = Equal?(x=w1957, y=u16 8) -> (x = y?=w1962:bool)
        "校零错误" <- w1962
        n1253 = Equal?(x=w1957, y=u16 7) -> (x = y?=w1961:bool)
        "校标错误" <- w1961
        n1254 = Equal?(x=w1957, y=u16 1) -> (x = y?=w1968:bool)
        "ORP故障" <- w1968
        n1255 = Compound Arithmetic op=OR ("复合运算")(w1968, w1967, w1966, w1965, w1964, w1963, w1961, w1962, w1960, w1959) -> (→"故障标记":bool)
        n1256 = Bundle By Name(cluster=T2 {"ORP故障"=FALSE, "温控器故障"=FALSE, "加热故障"=FALSE, "高锰酸钾报警"=FALSE, "草酸钠报警"=FALSE, "测量错误"=FALSE, "校零错误"=FALSE, "校标错误"=FALSE, " 进水样超量程"=FALSE, "排液阀故障"=FALSE} ("报警簇"), "ORP故障"=w1968, "温控器故障"=w1967, "加热故障"=w1966, "高锰酸钾报警"=w1965, "草酸钠报警"=w1964, "测量错误"=w1963, "校零错误"=w1962, "校标错误"=w1961, "进水样超量程"=w1960, "排液阀故障"=w1959) -> (→"报警簇":T2)
      }
    }
  }
